vi "Actor Core.vi"(8 "error in":errorcluster, 11 "Composite User Interface in":refnum<class "GUI.lvclass">) -> (0 "error out":errorcluster, 3 "Actor out":refnum<class "Actor.lvclass">)   [LabVIEW 2020, in "GUI.lvlib" / "GUI.lvclass"]
doc: "The user interface for this panel.\n----\nCopyright: MGI 2016\nAuthor: Derek Trepanier"
uses:
  GUI.lvclass
  Task selection df.ctl
  Task info df.ctl
  C:/Program Files/National Instruments/LabVIEW 2020/vi.lib/MGI/Panel Manager/Panel Actor/Panel Actor/Panel Actor.lvclass
  C:/Program Files/National Instruments/LabVIEW 2020/vi.lib/ActorFramework/Actor/Actor.lvclass
  <vilib>/ActorFramework/Actor/Actor.lvclass
  Subject and File df.ctl
  Automate df.ctl
  <vilib>/MGI/Panel Manager/Panel/Window Position/Reference Position/Ref Display/Ref Display.lvclass
  C:/Program Files/National Instruments/LabVIEW 2020/vi.lib/MGI/Panel Manager/Panel/Window Position/Window Position.lvclass
  Acceleration Markers df.ctl
  EMG channels df.ctl
  Task Active Enum df.ctl
  Logging/Logging.lvclass
  GUI.lvclass/GUI.ctl
  NI Force Task/NI Force Task.lvclass
  <vilib>/ActorFramework/Actor/Actor.lvclass/Actor.ctl
  <vilib>/ActorFramework/Message Enqueuer/Message Enqueuer.lvclass/Message Enqueuer.ctl
  NI Force Task Messages/Update Template Graph Msg/Update Template Graph Msg.lvclass/Update Template Graph Msg.ctl
  Accelerometer/Accelerometer.lvclass
  Collection Type df.ctl
  Marker Enum.ctl
  <vilib>/ActorFramework/Message Enqueuer/Init from Existing Queue.vi
  <vilib>/ActorFramework/Message Enqueuer/Enqueue.vi
  <vilib>/MGI/Panel Manager/Panel/Panel/Window/Window.lvclass
  C:/Program Files/National Instruments/LabVIEW 2020/vi.lib/MGI/Panel Manager/Panel/Panel/Panel.lvclass
  NI Force Task Messages/Update Template Graph Msg/Update Template Graph Msg.lvclass
  C:/Program Files/National Instruments/LabVIEW 2020/vi.lib/ActorFramework/Message/Message.lvclass
  <vilib>/MGI/Panel Manager/Panel/Panel/Subpanel/Subpanel.lvclass
  <vilib>/ActorFramework/Stop Msg/Stop Msg.lvclass
  <vilib>/MGI/Panel Manager/Panel/Panel/Window/Window.vi
  <vilib>/ActorFramework/Message Priority Queue/Priority Enqueue.vi
  <vilib>/MGI/Panel Manager/Panel/Panel/Subpanel/Subpanel.vi
  <vilib>/ActorFramework/Message Enqueuer/Message Enqueuer.lvclass
  <vilib>/MGI/Panel Manager/Panel Actor/Panel Actor/Panel Actor.lvclass
  <vilib>/MGI/Panel Manager/Panel/Panel.lvlib
  GUI Messages/Set Template Data Msg/Set Template Data Msg.lvclass
  NI Force Task Messages/Start Trial Msg/Start Trial Msg.lvclass
  NI Force Task Messages/Stop Trial Msg/Stop Trial Msg.lvclass
  NI Force Task Messages/External Shutdown Msg/External Shutdown Msg.lvclass
  Accelerometer Messages/Stop Trial Msg/Stop Trial Msg.lvclass
  Accelerometer Messages/Initialize Accel Task Msg/Initialize Accel Task Msg.lvclass
  Accelerometer Messages/Start Trial Msg/Start Trial Msg.lvclass
  Accelerometer Messages/External Shutdown Msg/External Shutdown Msg.lvclass
  NI Force Task Messages/Calibrate Force Msg/Calibrate Force Msg.lvclass
  NI Force Task Messages/Collect MVC Msg/Collect MVC Msg.lvclass
  GUI Messages/Does File Exist Msg/Does File Exist Msg.lvclass
  Logging Messages/TDMS Cleanup Msg/TDMS Cleanup Msg.lvclass
  GUI Messages/Save or Load Config Msg/Save or Load Config Msg.lvclass
  GUI Messages/Delete Config Msg/Delete Config Msg.lvclass
  GUI Messages/MVC Collect File Check Msg/MVC Collect File Check Msg.lvclass
  NI Force Task Messages/Launch Viewer Msg/Launch Viewer Msg.lvclass
  NI Force Task Messages/Calibrate Potentiometers Msg/Calibrate Potentiometers Msg.lvclass
  NI Force Task Messages/Initialize Movement Task Msg/Initialize Movement Task Msg.lvclass
  NI Force Task Messages/Initialize Force Task Msg/Initialize Force Task Msg.lvclass
  GUI Messages/Update Patterns Array Msg/Update Patterns Array Msg.lvclass
  C:/Program Files/National Instruments/LabVIEW 2020/vi.lib/MGI/Panel Manager/Panel/Window Position/Reference Position/Reference Position.lvclass
  C:/Program Files/National Instruments/LabVIEW 2020/vi.lib/MGI/Panel Manager/Panel/Window Position/Reference Position/Ref Display/Ref Display.lvclass
  GUI Messages/Task Type Change Msg/Task Type Change Msg.lvclass
  GUI Messages/Accel Marker Update Msg/Accel Marker Update Msg.lvclass
  NI Force Task Messages/Initiallize EMG Task Msg/Initiallize EMG Task Msg.lvclass
  Logging Messages/TDMS Cleanup EMG only Msg/TDMS Cleanup EMG only Msg.lvclass
  GUI Messages/Scale Regression Msg/Scale Regression Msg.lvclass
panel:
  out "MVC Temp":dbl
  in  "Monitor Select":refnum<class "Ref Display.lvclass">
  out "Abort Signal":bool
  in  "Subject and File":T1={"File Save Path"=path "\\\\coe-fs.engr.tamu.edu\\Grads/renee.woodruff/Documents/LabVIEW Data/Bimanual Coord DAQ", "File Name "="test"}
  in  "Tab Control":T2(tab)
  in  "Abort Task":bool caption="Preview Task"
  in  "Task Previewed?":bool
  in  "Preview Task":bool
  in  "Task Selection":T3={"Task Type Select"=enum."Frequency Task", "Input Select Type"=enum."Force Input", "Collect EMG?"=FALSE, "Collect acceleration?"=TRUE, "EMG Rate"=1000, "Acceleration Rate"=50} {"Acceleration Rate" min=5 max=1000 step=1; "EMG Rate" min=1 step=1}
  in  "Task Info Cluster":T4={"Number of Trials"=1, "Sampling Rate (Hz)"=100, "Trial Duration (s)"=8, "Adjusted MVC (N)"=5.0, "R Phase"=0, "L Phase"=0, "L Pattern"=1, "R Pattern"=1, "Time Between Trials (s)"=5, "Lissajous Speed"=10} {"Lissajous Speed" min=1 max=200; "Time Between Trials (s)" min=1 step=1; "R Pattern" min=1 max=20 step=1; "L Pattern" min=1 max=20 step=1; "L Phase" max=360 step=1; "R Phase" max=360 step=1; "Adjusted MVC (N)" min=0.1 max=50.0 step=0.10000000149011612 format="%.1f"; "Trial Duration (s)" min=1 step=1; "Sampling Rate (Hz)" min=1 step=1; "Number of Trials" min=1 step=1}
  in  "Task Start":bool caption="Force Task Start"
  in  "Delete Config":bool
  in  "Config Select":string(combo) caption="Load or Save Config:"
  in  "Collect MVC":bool
  in  "MVC Cluster input":T5={"MVC Sampling Rate"=200, "MVC Duration"=3, "MVC Percent"=15} {"MVC Percent" max=100 step=1 scale=0.0..40.0; "MVC Duration" min=1 step=1; "MVC Sampling Rate" min=1 step=1}
  out "Raw MVC Clust":cluster{"Raw MVC Left":dbl, "Raw MVC Right":dbl}
  out "Adjusted MVC Cluster":T6
  out "Slope Int":dbl[][](array[numeric])
  in  "Calc Regression":bool
  in  "TScale Calibration":dbl[][](array[numeric])
  in  "Calibrate Pot":bool caption="Calibrate"
  in  "Calibrate Transducers":bool
  out "Force Calibration Cluster":cluster{"Left":dbl, "Right":dbl}
  in  "Force Calibration Input Cluster":T7={"Force Calib Sampling Rate"=200, "Force Calib Duration"=3}
  out "Pot Calibration Cluster":cluster{"Left 2":dbl, "Right 2":dbl}
  in  "Pot Calibration Input Clust":T7={"Force Calib Sampling Rate"=200, "Force Calib Duration"=3}
  in  "EMG Master Config":T8
  in  "DAQ Physical Channels":T9={"Force Transducer: Left"="Dev1/ai6", "Force Transducer: Right "="Dev1/ai8", "EMG: Left"="Dev1/ai1", "EMG: Right"="Dev1/ai9", "Potentiometer: Left"="Dev2/ai2", "Potentiometer: Right"="Dev2/ai3"}
  out "Trial Num":i32=1
  in  "Tab Control Automation":T10(tab)
  in  "Auto Clust":T11={"Automate?"=FALSE, "Num Parabs"=1, "Patterns Array"=[], "Phase Array"=[]} {"Num Parabs" min=1 step=1}
  in  "Acceleration Markers":T12
  in  "Second Monitor":bool caption="Display task on second monitor"
  in  "Task window closed?":bool
  # "Save File Information"
  # "(do not include file type)"
  # "Task Type"
  # "Left Arm"
  # "Right Arm"
  # "Force Calibration"
  # "Regression in Use"
  # "Weight (lbs)"
  # "Left (V)"
  # "Right (V)"
  # "Slope"
  # "Int."
  # "Left"
  # "Right"
  # "Re-calculates regression line to convert volts to Newtons for transducer.\nOnly needs to be done if transducer is changed."
  # "Potentiometer Calibration"
  # "Note: running EMG Master \nMode will simultaneously \ncollect EMG data from the \nspecified channels on the right.\nOnly 1 laptop should run EMG\nMaster Mode at a time\n\nForce/potentiometer data will\nNOT be collected in this mode"
  # "- Check the Device Configuration tab before running. Make sure that the Device Name is valid for each channel by selecting the dropdown menu to see if the value is listed. If yes, change nothing. If yes, change the channel to a listed Device Name/Channel combination. \n- Re-calibrate transducers every time 'gravity' is changed or starting a test session for the day in the Calibration tab\n- In the Task Config tab, it is best when Force Sampling Rate (Hz) is a multiple of the EMG Sampling Rate (Hz). If you are not collecting EMG, this doesn't matter\n- If the cursor ever becomes 'busy', seen as a blue circle, do not select anything until the cursor is no longer busy\n- If the config drop down does not work, open '/config/config_list.txt' and type in \"Create New...\". Save the .txt and then close it. Close the program and try again\n- Make sure that the headset is connected as the secondary display, if applicable\n- Note: Acceleration Markers will be cleared for each new set of trials \n- Acceleration markers can also be added using keyboard inputs. To add markers this way, make sure the User Interface window is in focus"
  # "Patterns"
  # "Phase"
  # "Left        Right"
  # "Left        Right"
  # "Insert Acceleration Markers"
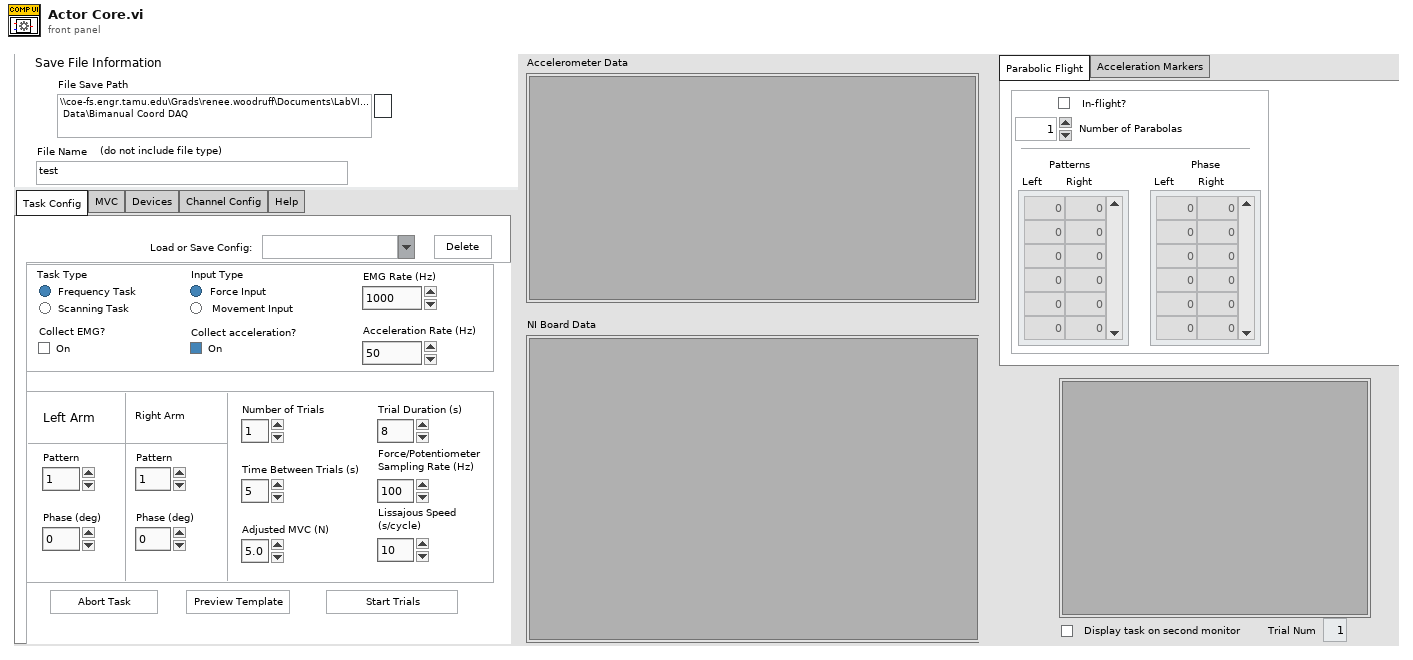
[diagram p1: front panel]
types:
  T1 = typedef "Subject and File df.ctl" = cluster{"File Save Path":path, "File Name ":string}
  T2 = enum32{"Task Config", "MVC", "Devices", "Channel Config", "Help"}
  T3 = typedef "Task selection df.ctl" = cluster{"Task Type Select":enum32{"Frequency Task", "Scanning Task"}, "Input Select Type":enum32{"Force Input", "Movement Input"}, "Collect EMG?":bool, "Collect acceleration?":bool, "EMG Rate":u16, "Acceleration Rate":u16}
  T4 = typedef "Task info df.ctl" = cluster{"Number of Trials":u8, "Sampling Rate (Hz)":u16, "Trial Duration (s)":u8, "Adjusted MVC (N)":dbl, "R Phase":i32, "L Phase":i32, "L Pattern":u8, "R Pattern":u8, "Time Between Trials (s)":u8, "Lissajous Speed":u16}
  T5 = cluster{"MVC Sampling Rate":u16, "MVC Duration":u8, "MVC Percent":u8}
  T6 = cluster{"Adjusted MVC Left":dbl, "Adjusted MVC Right":dbl}
  T7 = cluster{"Force Calib Sampling Rate":u16, "Force Calib Duration":u8}
  T8 = typedef "EMG channels df.ctl" = cluster{"EMG Master":bool, "EMGL1":tag, "EMGR1":tag, "EMGL2":tag, "EMGR2":tag, "EMGL3":tag, "EMGR3":tag, "EMGL4":tag, "EMGR4":tag, "EMGL5":tag, "EMGR5":tag, "EMGL6":tag, "EMGR6":tag, "EMGL7":tag, "EMGR7":tag, "EMGL8":tag, "EMGR8":tag}
  T9 = cluster{"Force Transducer: Left":tag, "Force Transducer: Right ":tag, "EMG: Left":tag, "EMG: Right":tag, "Potentiometer: Left":tag, "Potentiometer: Right":tag}
  T10 = enum32{"Parabolic Flight", "Acceleration Markers"}
  T11 = typedef "Automate df.ctl" = cluster{"Automate?":bool, "Num Parabs":u16, "Patterns Array":u8[][], "Phase Array":i32[][]}
  T12 = typedef "Acceleration Markers df.ctl" = cluster{"Partial g marker":bool, "1g marker":bool, "Hyper G marker":bool, "Custom Marker":bool, "Enter Marker Name":string, "Marker List":i32, "Delete Row":bool}
  T13 = typedef "Task Active Enum df.ctl" = enum16{"Idle", "Start Freq Task", "Start Freq Task and Accel", "Start Scanning Task", "Start Scanning Task and Accel", "Preview Template", "Collect MVC", "Calibrate Force", "Calibrate Potentiometers", "Stop Helper", "EMG Mode", "EMG and Accel Mode", "Task Config Update"}
  T14 = typedef "NI_LVConfig.lvlib/Config Data RefNum.ctl" = refnum<k1>
  T15 = cluster{"Preview Task":refnum<user-event>, "Calibration Val Update":refnum<user-event>, "Raw MVC update":refnum<user-event>, "Task Info Load":refnum<user-event>, "Task Select Load":refnum<user-event>, "Config Update":refnum<user-event>, "Task window update":refnum<user-event>, "Pot Cal Value Update":refnum<user-event>, "Auto Clust Update":refnum<user-event>, "Accel Markers":refnum<user-event>, "Slope Int":refnum<user-event>, "Trial Num Update":refnum<user-event>}
  T16 = cluster{"Event Registration Refnum":refnum<event-registration>, "Pnl Actor":refnum<event-registration>}
  T17 = enum8{"Enabled", "Disabled", "Disabled and Grayed Out"}
  T18 = typedef "Marker Enum.ctl" = enum16{"Predefined", "Custom", "Delete Row", "Clear all"}
  T19 = typedef "LVPoint32TypeDef.ctl" = cluster{"Horizontal":i32, "Vertical":i32}
  T20 = typedef "LVRowAndColumnTypeDef.ctl" = cluster{"Row":i32, "Column":i32}
  T21 = enum16{"open", "open or create", "create or replace", "create", "open (read-only)"}
  T22 = typedef "Collection Type df.ctl" = enum32{"Force Input", "Movement Input", "EMG only"}
  T23 = cluster{"Force Task":refnum<class "NI Force Task.lvclass">, "Window out":refnum<class "Window.lvclass">}
  T24 = cluster{"Accelerometer":refnum<class "Accelerometer.lvclass">, "Subpanel Out":refnum<class "Subpanel.lvclass">}
  T25 = cluster{"Accelerometer":refnum<class "Panel Actor.lvclass">, "Subpanel Out":refnum<class "Panel.lvclass">}[]
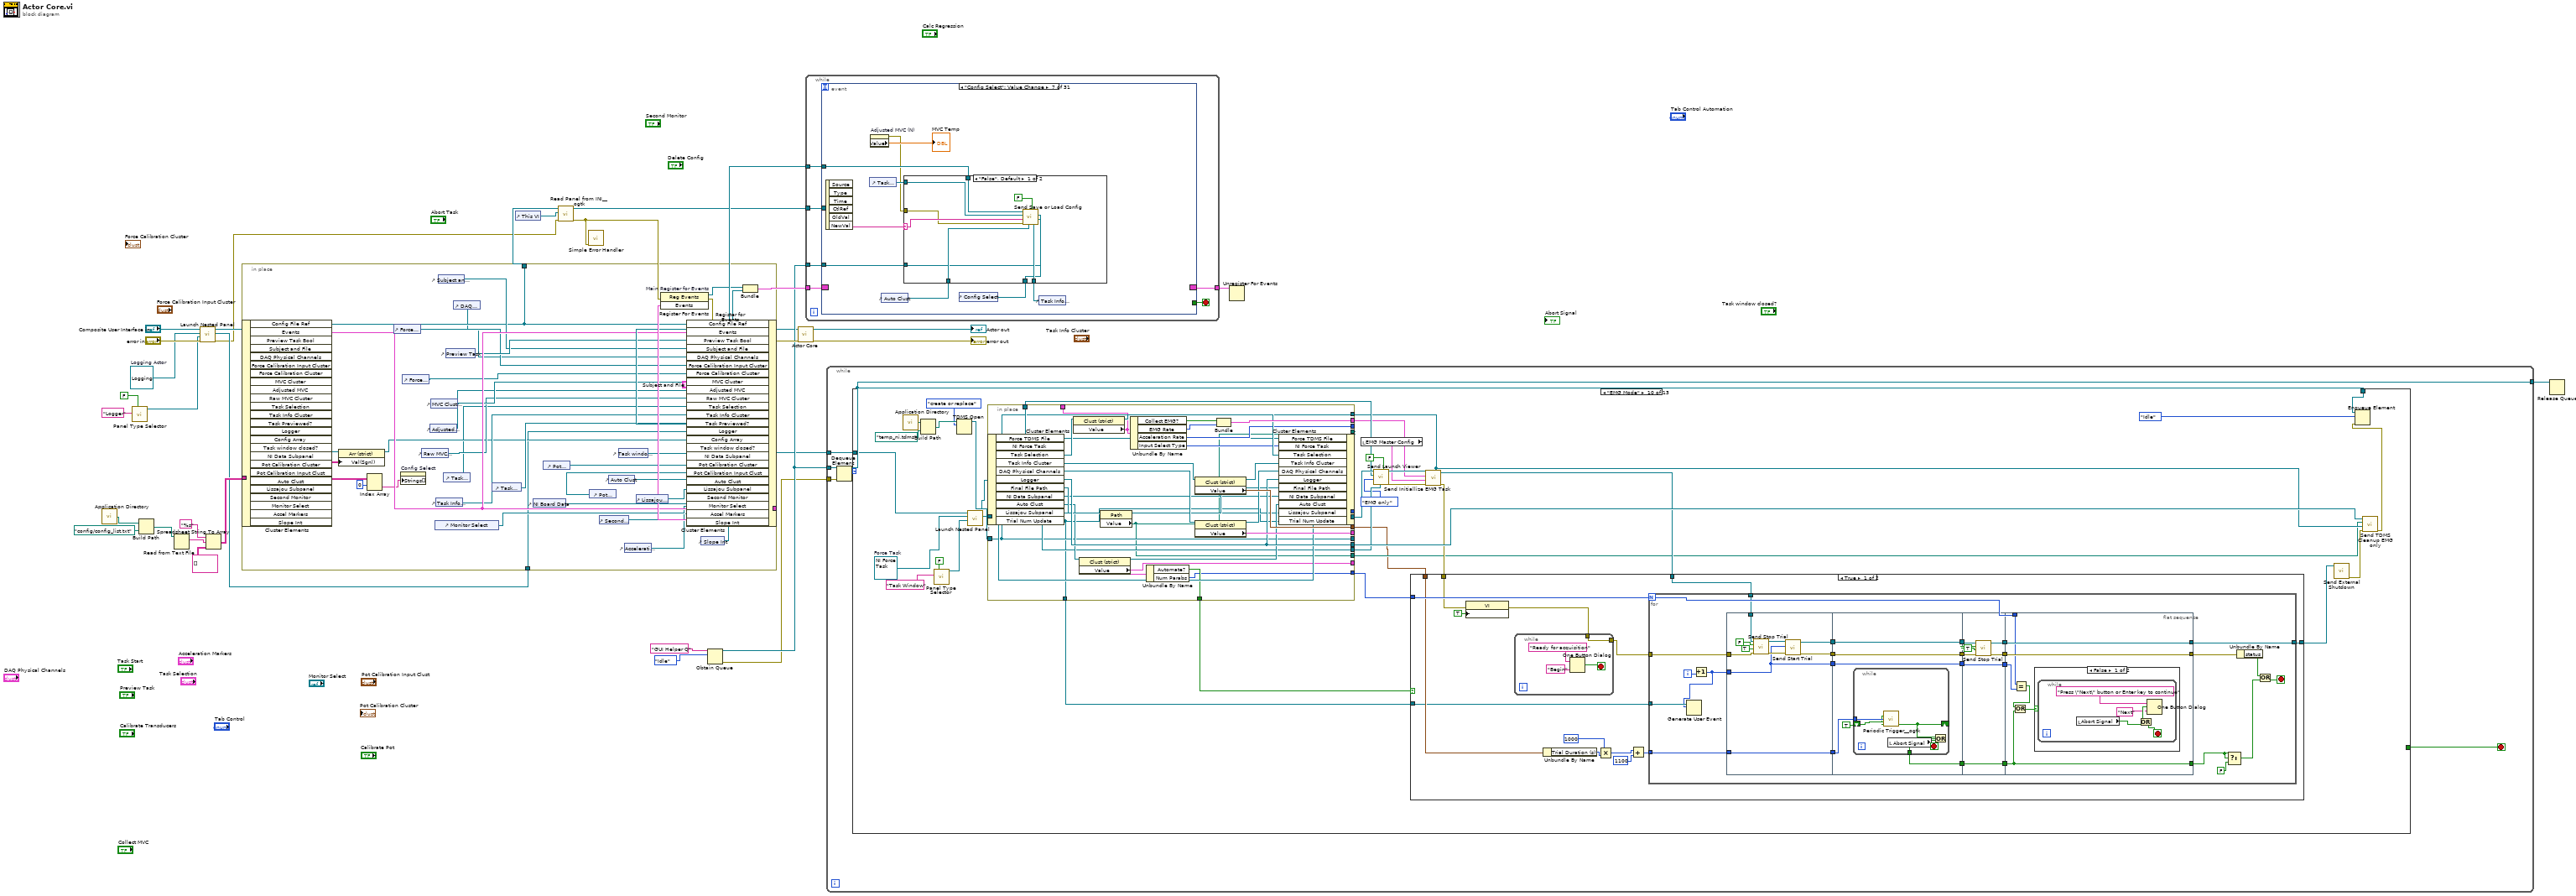
[diagram p0: block diagram]
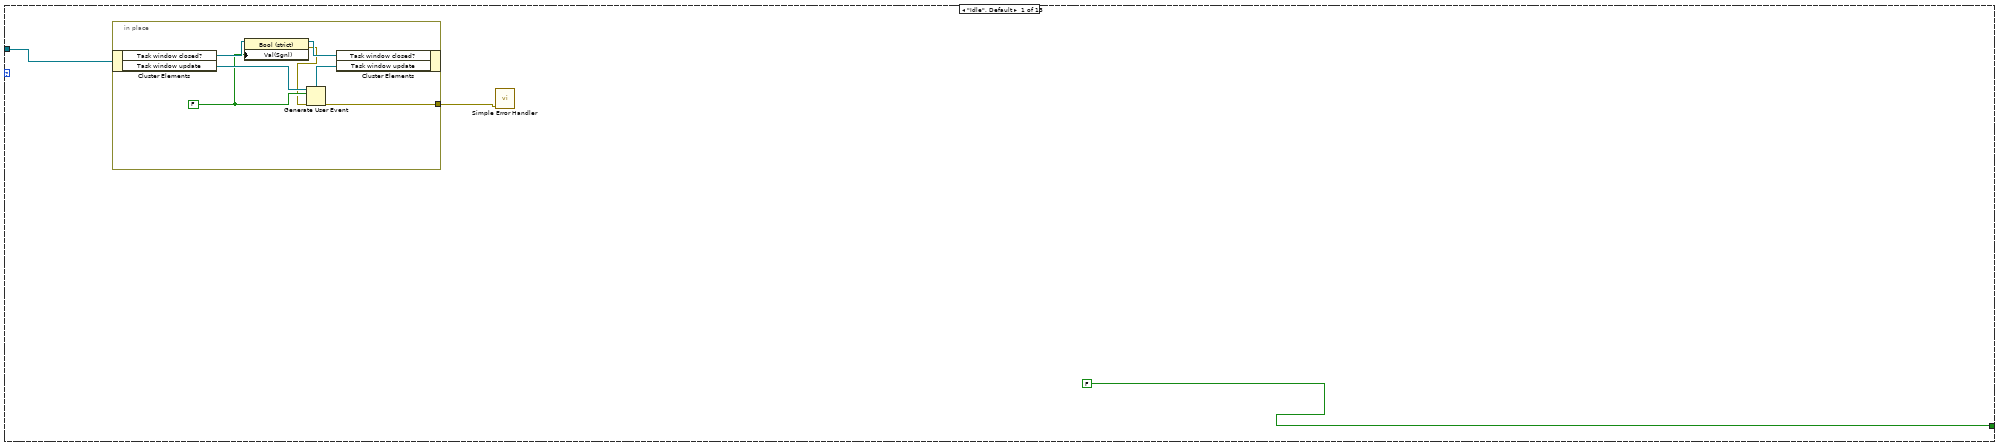
[diagram p2: hidden frame]
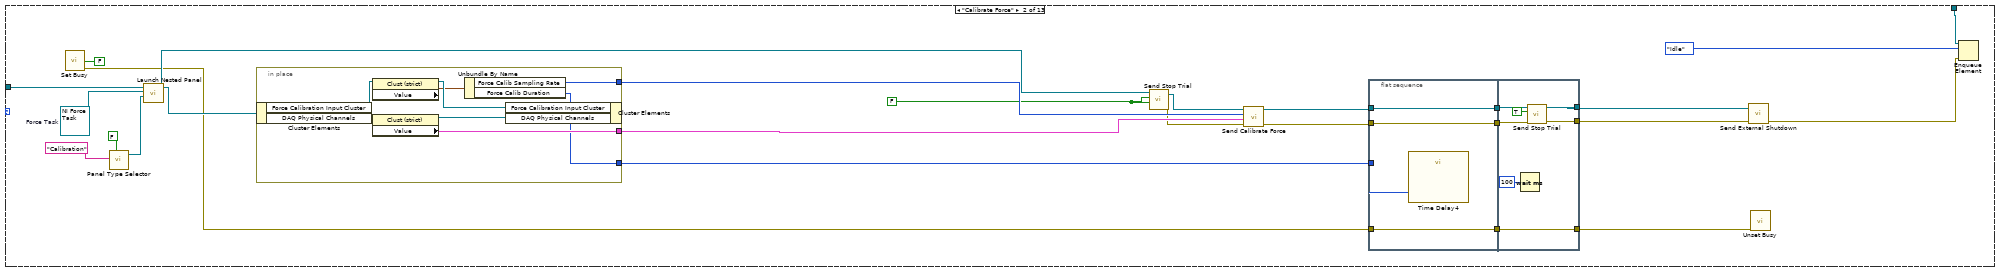
[diagram p3: hidden frame]
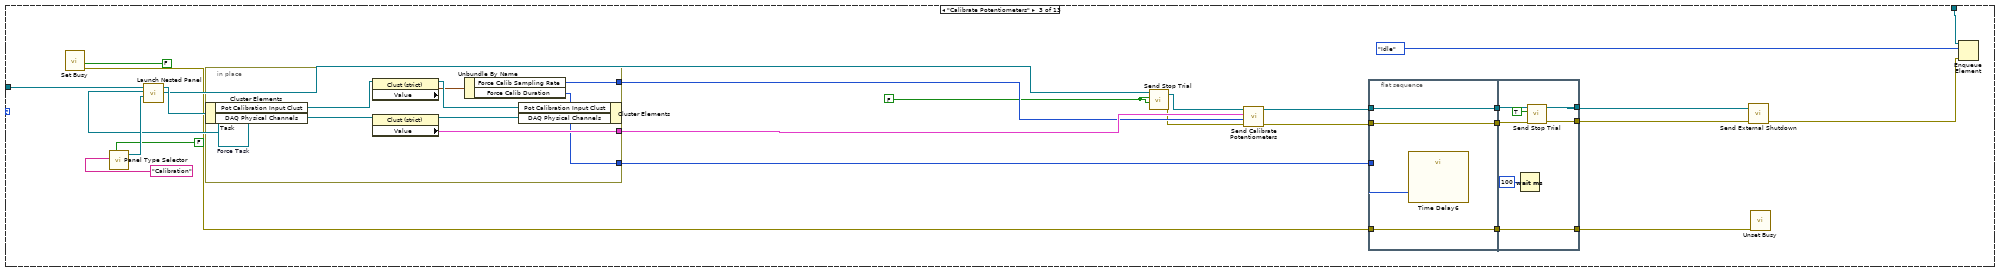
[diagram p4: hidden frame]
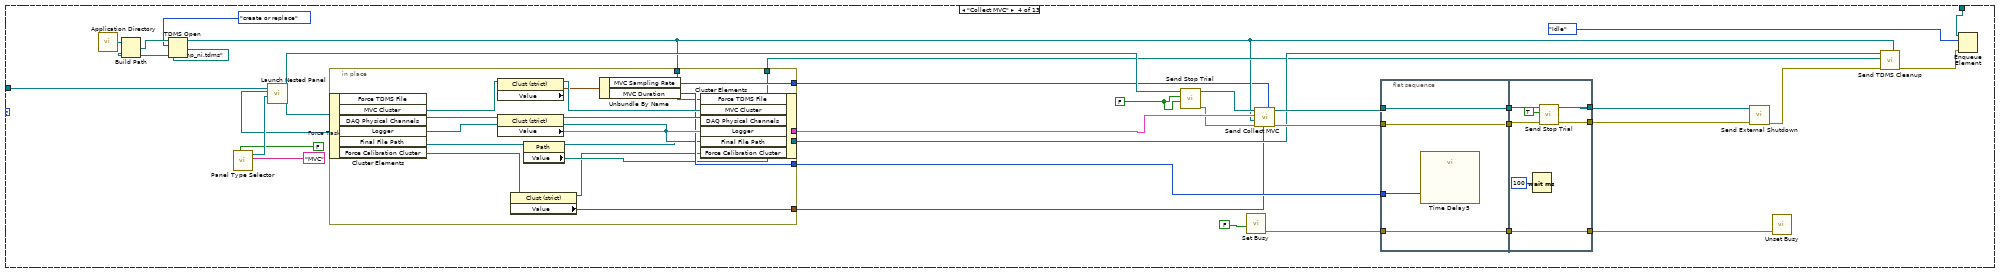
[diagram p5: hidden frame]
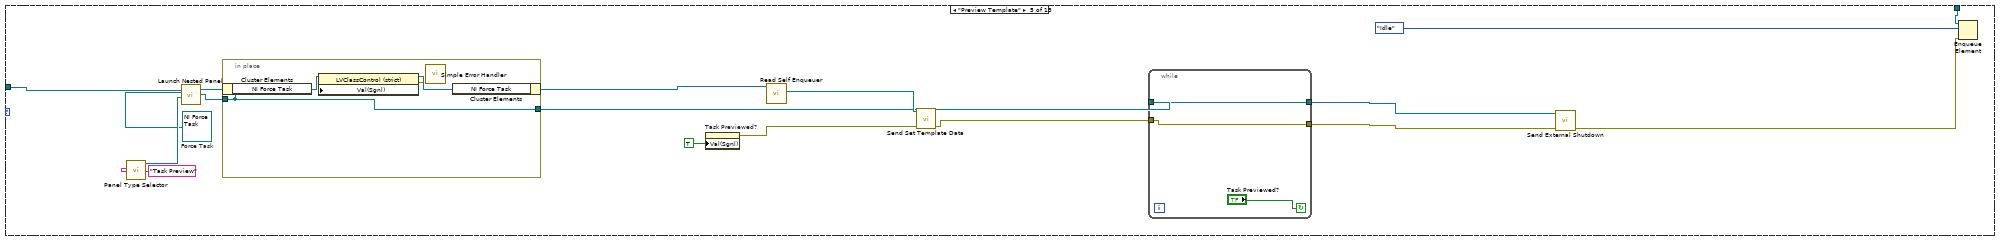
[diagram p6: hidden frame]
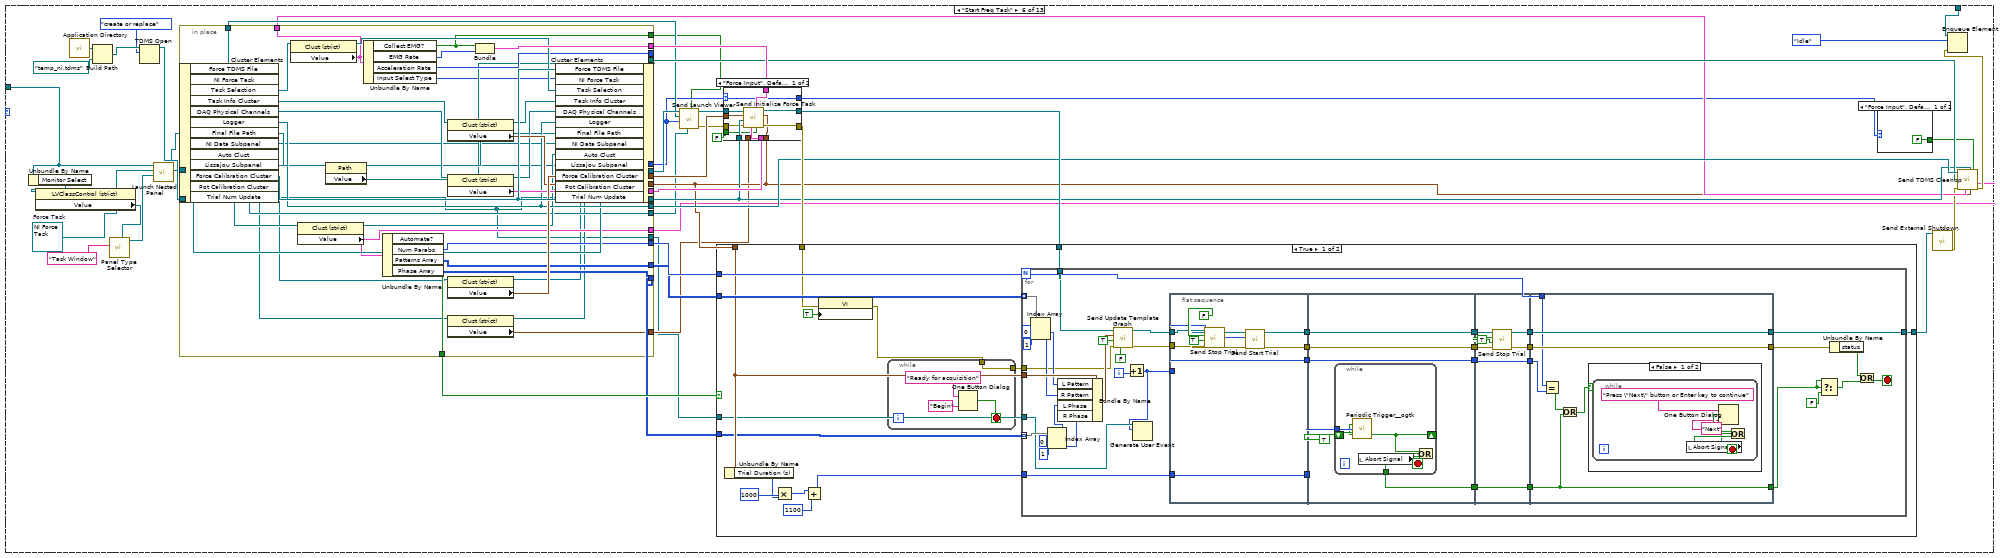
[diagram p7: hidden frame]
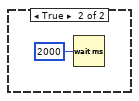
[diagram p8: hidden frame]
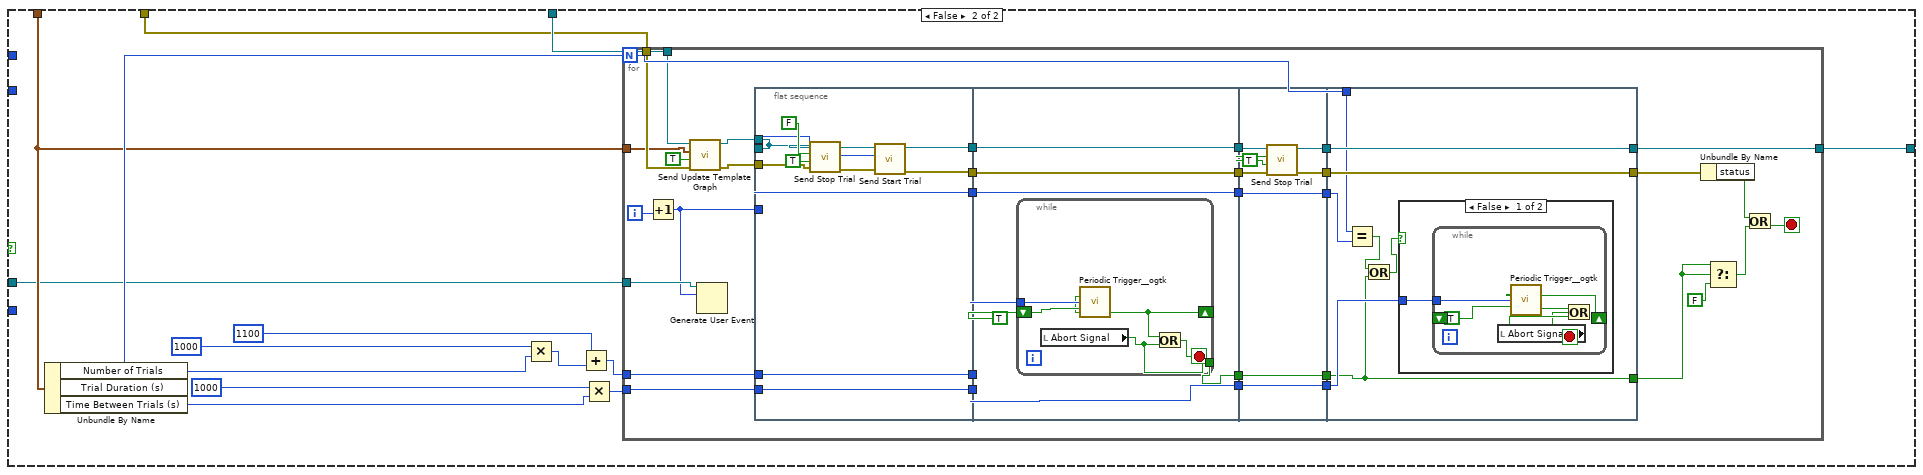
[diagram p9: hidden frame]
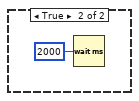
[diagram p10: hidden frame]
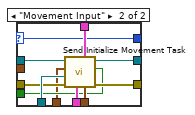
[diagram p11: hidden frame]
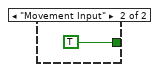
[diagram p12: hidden frame]
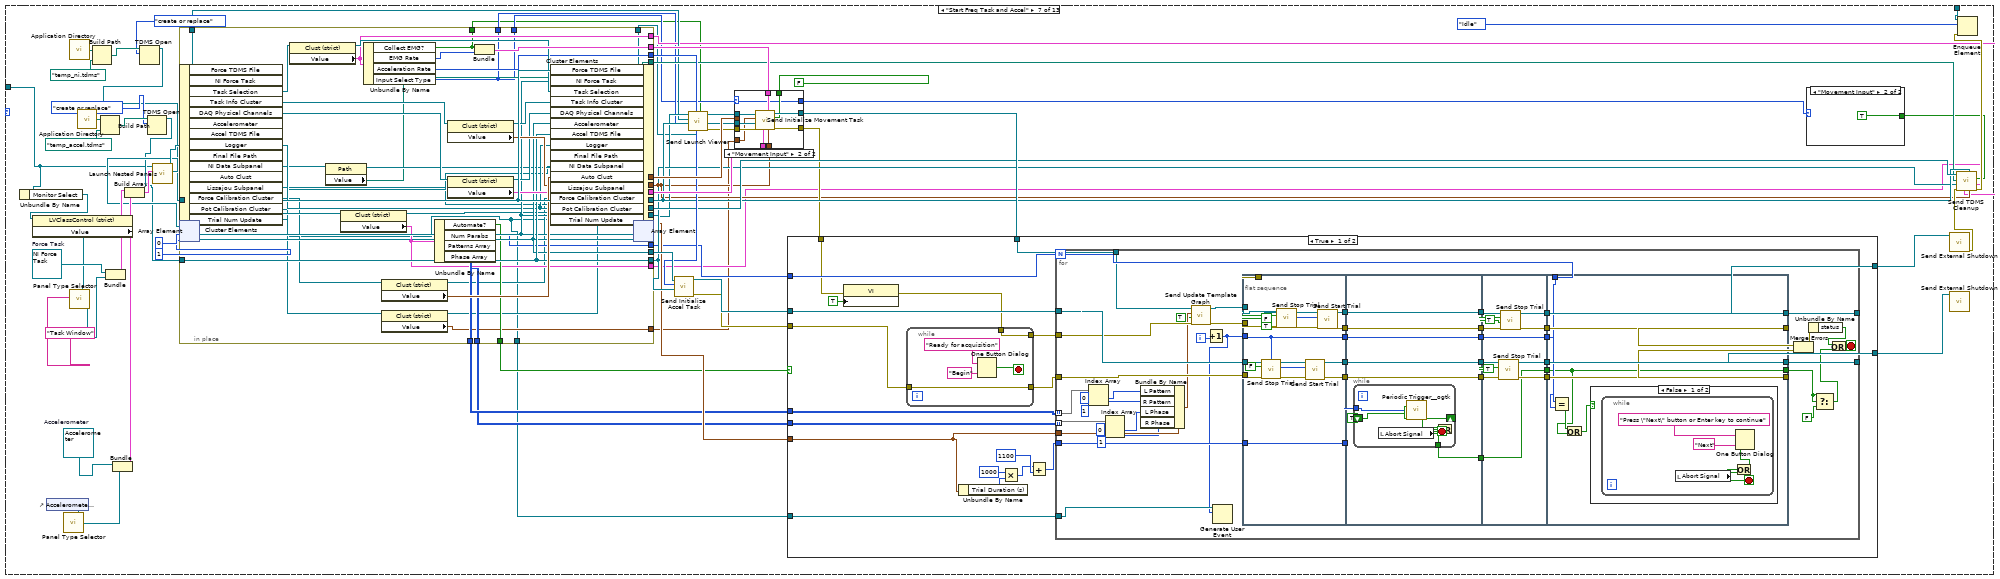
[diagram p13: hidden frame]
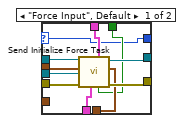
[diagram p14: hidden frame]
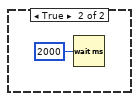
[diagram p15: hidden frame]
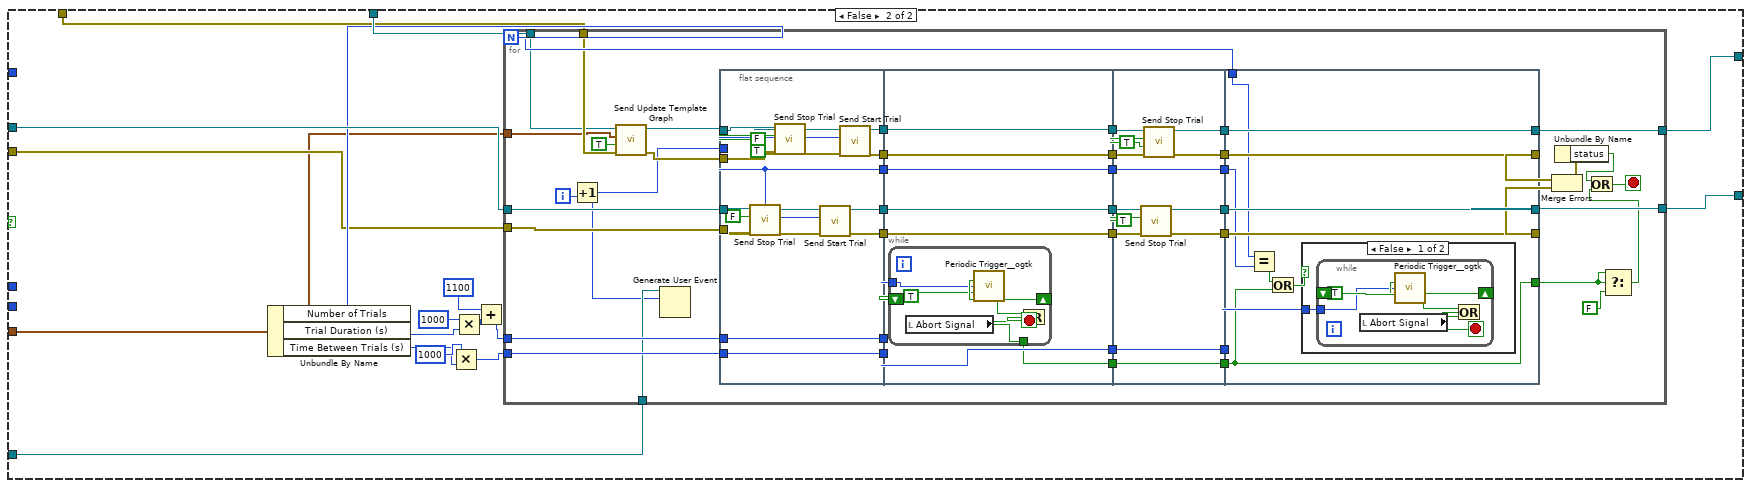
[diagram p16: hidden frame]
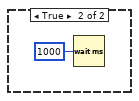
[diagram p17: hidden frame]
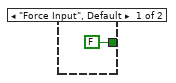
[diagram p18: hidden frame]
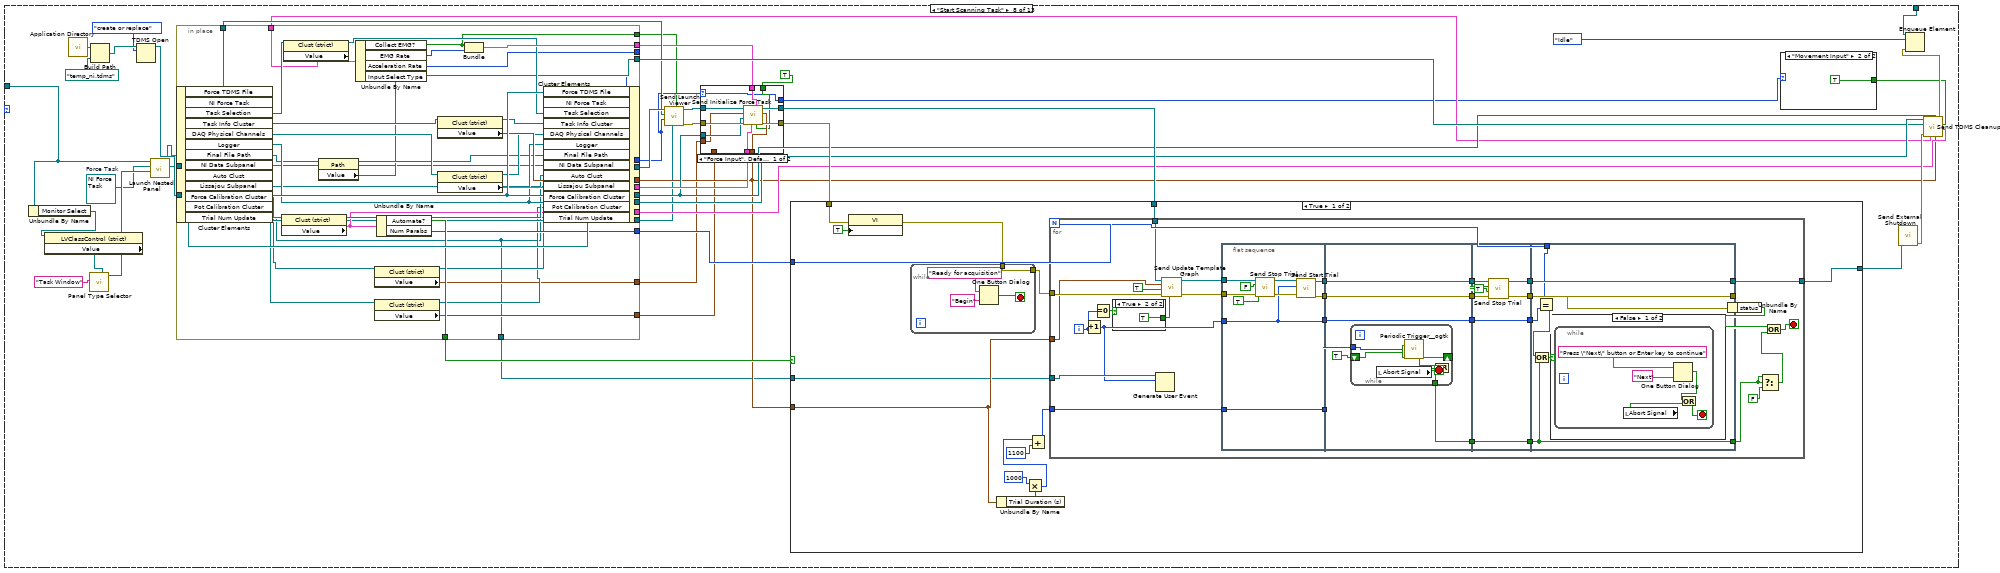
[diagram p19: hidden frame]
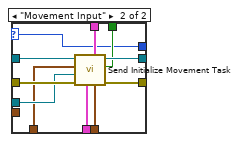
[diagram p20: hidden frame]
diagram:
  w5 = refnum<class "Logging.lvclass"> refnum  # Logging Actor
  n1 = call <vilib>:"Application Directory.vi"() -> ("Application Directory"=w15:path)
  n2 = call-poly <vilib>:"Panel Type Selector.vi"("Autoshow? (T)"=FALSE, "Default Title"="Logger") -> ("Window out"=w4:refnum<class "Window.lvclass">)  [unwired: 8 in, 1 out]
  n3 = Build Path(base path=w15, name or relative path=path "config/config_list.txt") -> (appended path=w13:path)
  n4 = Read from Text File(file (use dialog)=w13) -> (text=w12:string)  [unwired: 3 in, 3 out]
  n5 = call <vilib>:"Launch Nested Panel.vi"("error in (no error)"="error in", "Panel"=w4, "Nested Panel Actor"=w5, "Panel Actor in"="Composite User Interface in") -> ("error out"=w2:errorcluster, "Nested Actor's Enqueuer"=w3:refnum<class "Message Enqueuer.lvclass">, "Panel Actor out"=w20:refnum<class "GUI.lvclass">)  [unwired: 4 in, 1 out]
  n6 = Spreadsheet String To Array(format string="%s", spreadsheet string=w12, array type (2D Dbl)=string[][] []) -> (array=w9:string[][])  [unwired: 1 in]
  n7 = in-place {
    in-place-border: [w66] -> w19
    in-place-border: w9 -> [w53]
    in-place-border: [w52] -> w7
    in-place-border: w3 -> [w40]
    n8 = in-place-cluster #1(w20) -> ("Config File Ref"=w52:T14, "Events"=w66:T15, "Config Array"=w56:refnum<vi>)  [unwired: 22 out]
    n9 = property class="Arr (strict)"(reference=w56, "Val(Sgnl)"=w53) -> (reference out=w50:refnum<vi>)  [unwired: 1 in, 1 out]
    n10 = Index Array(array=w53, index (row)=0) -> (element=w54:string[])  [unwired: 1 in]
    n11 = control-ref of="Force Calibration Input Cluster"() -> (w59:refnum<vi>)
    n12 = property on="Config Select" class="CmbBox"("Strings[]"=w54) -> ()  [unwired: 2 in, 2 out]
    n13 = control-ref of="Force Calibration Cluster"() -> (w58:refnum<vi>)
    n14 = control-ref of="Raw MVC Clust"() -> (w61:refnum<vi>)
    n15 = control-ref of="Adjusted MVC Cluster"() -> (w60:refnum<vi>)
    n16 = control-ref of="MVC Cluster input"() -> (w62:refnum<vi>)
    n17 = control-ref of="Monitor Select"() -> (w41:refnum<vi>)
    n18 = control-ref of="Task Info Cluster"() -> (w63:refnum<vi>)
    n19 = control-ref of="Subject and File"() -> (w64:refnum<vi>)
    n20 = control-ref of="Task Selection"() -> (w45:refnum<vi>)
    n21 = control-ref of="Preview Task"() -> (w65:refnum<vi>)
    n22 = control-ref of="DAQ Physical Channels"() -> (w48:refnum<vi>)
    n23 = control-ref of="Task Previewed?"() -> (w57:refnum<vi>)
    n24 = control-ref of="NI Board Data"() -> (w49:refnum<vi>)
    n25 = control-ref of="Pot Calibration Cluster"() -> (w46:refnum<vi>)
    n26 = control-ref of="Pot Calibration Input Clust"() -> (w47:refnum<vi>)
    n27 = control-ref of="Second Monitor"() -> (w42:refnum<vi>)
    n28 = control-ref of="Auto Clust"() -> (w44:refnum<vi>)
    n29 = control-ref of="Task window closed?"() -> (w51:refnum<vi>)
    n30 = control-ref of="Acceleration Markers"() -> (w39:refnum<vi>)
    n31 = control-ref of="Lissajou Subpanel"() -> (w43:refnum<vi>)
    n32 = control-ref of="Slope Int"() -> (w38:refnum<vi>)
    n33 = in-place-cluster #1("Config File Ref"=w52, "Events"=w66, "Preview Task Bool"=w65, "Subject and File"=w64, "DAQ Physical Channels"=w48, "Force Calibration Input Cluster"=w59, "Force Calibration Cluster"=w58, "MVC Cluster"=w62, "Adjusted MVC"=w60, "Raw MVC Cluster"=w61, "Task Selection"=w45, "Task Info Cluster"=w63, "Task Previewed?"=w57, "Logger"=w40, "Config Array"=w50, "Task window closed?"=w51, "NI Data Subpanel"=w49, "Pot Calibration Cluster"=w46, "Pot Calibration Input Clust"=w47, "Auto Clust"=w44, "Lissajou Subpanel"=w43, "Second Monitor"=w42, "Monitor Select"=w41, "Accel Markers"=w39, "Slope Int"=w38) -> (w18:refnum<class "GUI.lvclass">)
  }
  n34 = control-ref of="This VI"() -> (w8:refnum<vi>)
  n35 = call <userlib>:"Read Panel from INI__ogtk.vi"("error in (no error)"=w2, "VI ref"=w8, "refnum"=w7) -> ("error out"=w1:errorcluster, "refnum out"=w6:T14)  [unwired: 7 in]
  n36 = call <vilib>:"Simple Error Handler.vi"("error in (no error)"=w1) -> ()  [unwired: 4 in, 5 out]
  n37 = register-events "Main Register for Events"(error in=w1, w19) -> (reference out=w29:refnum<event-registration>, error out=w30:errorcluster)  [unwired: 1 in]
  n38 = Obtain Queue(name (unnamed)="GUI Helper Q", element data type=Task_Active_Enum_df."Idle" ("Task Status Enum")) -> (queue out=w24:refnum<queue>, error out=w23:errorcluster)  [unwired: 3 in, 1 out]
  n39 = call <vilib>:"Register for Events.vi"("Error In"=w30, "Panel Actor in"=w18) -> ("Error Out"=w35:errorcluster, "Panel Actor out"=w22:refnum<class "GUI.lvclass">, "Pnl Actor"=w28:refnum<event-registration>, "Self Enqueuer"=w34:refnum<class "Message Enqueuer.lvclass">)  [unwired: 6 in]
  n40 = Bundle("Event Registration Refnum"=w29, "Pnl Actor"=w28) -> (w27:T16)  [unwired: 1 in]
  n41 = call-parent "Actor Core.vi"("error in"=w35, "Panel Actor in"=w22) -> ("error out"=→"error out":errorcluster, "Actor out"=→"Actor out":refnum<class "Actor.lvclass">)  [unwired: 8 in]
  n42 = while {
    tunnel: w27 -> [w72]
    tunnel: w34 -> [w71]
    tunnel: [w69] -> w33
    tunnel: w24 -> [w68]
    tunnel: w6 -> [w67]
    stop <- w70 stop-if-true
    n43 = event shown="[6] \"Config Select\": Value Change" {
      selector: w72 -> [_ _ _ _ _ _ _ _ _ _ _ _ _ _ _ _ _ _ _ _ _ _ _ _ _ _ _ _ _ _ _]
      dyn-events: [_ _ _ _ _ _ _ _ _ _ _ _ _ _ _ _ _ _ _ _ _ _ _ _ _ _ _ _ _ _ _] -> w69
      timeout: _ -> [_ _ _ _ _ _ _ _ _ _ _ _ _ _ _ _ _ _ _ _ _ _ _ _ _ _ _ _ _ _ _]
      tunnel: w71 -> [w75 _ w130 _ w139 _ w148 _ w179 w189 _ _ _ w251 w258 _ _ w265 _ _ w291 _ w297 w301 w307 w308 _ _ _ w334 _]
      tunnel: [_ _ _ _ _ _ _ _ _ _ _ _ _ _ _ _ _ _ _ _ _ _ _ _ _ _ _ _ _ _ w335] -> w70
      tunnel: w68 -> [w92 _ _ _ _ _ w143 _ _ _ _ _ _ _ _ w261 w263 w264 _ _ w290 _ _ _ _ _ _ _ w329 _ w336]
      tunnel: w67 -> [_ _ _ _ _ _ _ _ _ _ _ _ _ _ _ _ _ _ _ _ _ _ _ _ _ _ _ _ _ w332 _]
      event User Event {
        w78 = cluster{u32, u32}[] [{12369084, 12369084}, {12369084, 12369084}, {13816530, 13816530}] ("Colors [4]")
        n44 = event-data() -> ()  [unwired: 1 in, 1 out]
        n45 = control-ref of="Calibrate Pot"() -> (w82:refnum<vi>)
        n46 = control-ref of="Preview Task"() -> (w80:refnum<vi>)
        n47 = control-ref of="Delete Config"() -> (w84:refnum<vi>)
        n48 = Enqueue Element(queue=w92, element=Task_Active_Enum_df."Idle") -> ()  [unwired: 2 in, 3 out]
        n49 = property on="Acceleration Markers" class="Clust"() -> ("Controls[]"=w85:refnum<vi>[])  [unwired: 2 in, 2 out]
        n50 = call "Send Scale Regression.vi"("Read CSV"=TRUE, "Message Enqueuer in"=w75) -> ()  [unwired: 8 in, 2 out]
        n51 = control-ref of="Calibrate Transducers"() -> (w83:refnum<vi>)
        n52 = control-ref of="Collect MVC"() -> (w81:refnum<vi>)
        n53 = Build Array(w84, w83, w82, w81, w80) -> (w79:refnum<vi>[])
        n54 = for {
          tunnel: w79 -> [w93] mode=indexing
          tunnel: w78 -> [w94]
          n55 = property class="Bool"(reference=w93, "Colors [4]"=w94) -> ()  [unwired: 1 in, 2 out]
        }
        n56 = for {
          tunnel: w85 -> [w97]
          tunnel: w78 -> [w96]
          tunnel: i32[] [0, 1, 2, 3, 6] -> [w95] mode=indexing
          n57 = in-place {
            in-place-border: w96 -> [w101]
            w99 = refnum<vi> refnum  # Control
            w104 = refnum<vi> refnum  # Boolean
            n58 = in-place-array #2(w97, w95) -> (w105:refnum<vi>)
            n59 = To More Specific Class(target class=w104, reference=w105) -> (specific class reference=w103:refnum<vi>, error out=w102:errorcluster)  [unwired: 1 in]
            n60 = property class="Bool"(reference=w103, error in=w102, "Colors [4]"=w101) -> (reference out=w100:refnum<vi>)  [unwired: 1 out]
            n61 = To More Generic Class(target class=w99, reference=w100) -> (generic class reference=w98:refnum<vi>)
            n62 = in-place-array #2(w98) -> ()  [unwired: 2 out]
          }
        }
        n63 = property on="Auto Clust" class="Clust (strict)"() -> ("Controls[]"=w87:refnum<vi>[])  [unwired: 2 in, 2 out]
        n64 = property on="Task Selection" class="Clust (strict)"() -> ("Controls[]"=w90:refnum<vi>[])  [unwired: 2 in, 2 out]
        n65 = in-place {
          n66 = in-place-array #3(w90, 0, 1) -> (w117:refnum<vi>, w108:refnum<vi>)
          n67 = in-place-array #4(w87, 0) -> (w114:refnum<vi>)
          n68 = property class="Ctl"(reference=w114) -> (reference out=w113:refnum<vi>, "Value"=w111:variant)  [unwired: 1 in, 1 out]
          n69 = property class="Ctl"(reference=w117) -> (reference out=w116:refnum<vi>, "Value"=w115:variant)  [unwired: 1 in, 1 out]
          n70 = property class="Ctl"(reference=w108) -> (reference out=w109:refnum<vi>, "Value"=w110:variant)  [unwired: 1 in, 1 out]
          n71 = property class="Ctl"(reference=w113, "Val(Sgnl)"=w111) -> (reference out=w112:refnum<vi>)  [unwired: 1 in, 1 out]
          n72 = property class="Ctl"(reference=w116, "Val(Sgnl)"=w115) -> (reference out=w107:refnum<vi>)  [unwired: 1 in, 1 out]
          n73 = property class="Ctl"(reference=w109, "Val(Sgnl)"=w110) -> (reference out=w106:refnum<vi>)  [unwired: 1 in, 1 out]
          n74 = in-place-array #3(w107, w106) -> ()  [unwired: 3 out]
          n75 = in-place-array #4(w112) -> ()  [unwired: 2 out]
        }
        n76 = property on="Task Start" class="Bool"("Colors [4]"=cluster{u32, u32}[] [{50176, 50176}, {50176, 50176}, {6618880, 6618880}]) -> ()  [unwired: 2 in, 2 out]
        n77 = property on="Abort Task" class="Bool"("Colors [4]"=cluster{u32, u32}[] [{16711680, 16711680}, {16711680, 16711680}, {16711680, 16711680}]) -> ()  [unwired: 2 in, 2 out]
      }
      event Value Change {
        n78 = event-data() -> ("NewVal"=w120:bool)  [unwired: 1 in]
        n79 = case shown="False" w120 {
          tunnel: [T17."Disabled and Grayed Out" ("Disabled") T17."Enabled" ("Disabled")] -> w118
          frame False {
          }
          frame True {
          }
        }
        n80 = for {
          N: 8 -> [_]
          tunnel: w118 -> [w123]
          i -> [w124]
          n81 = Increment(x=w124) -> (x+1=w125:i32)
          n82 = property on="EMG Master Config" class="Clust (strict)"() -> ("Controls[]"=w126:refnum<vi>[])  [unwired: 2 in, 2 out]
          n83 = in-place {
            in-place-border: w123 -> [w127]
            n84 = in-place-array #5(w126, w125) -> (w129:refnum<vi>)
            n85 = property class="Ctl"(reference=w129, "DisabledEnum"=w127) -> (reference out=w128:refnum<vi>)  [unwired: 1 in, 1 out]
            n86 = in-place-array #5(w128) -> ()  [unwired: 2 out]
          }
        }
      }
      event Value Change {
        n87 = event-data() -> ("NewVal"=w131:u16, "OldVal"=w132:u16)  [unwired: 1 in]
        n88 = call "Send Update Patterns Array.vi"("Old Num of Parabolas"=w132, "Num of Parabolas"=w131, "Message Enqueuer in"=w130) -> ()  [unwired: 7 in, 2 out]
      }
      event User Event {
        n89 = event-data() -> ("Patterns Array"=w135:u8[][], "Phase Array"=w133:i32[][])  [unwired: 1 in]
        n90 = Bundle By Name(cluster="Auto Clust", "Patterns Array"=w135, "Phase Array"=w133) -> (w134:T11)
        n91 = property on="Auto Clust" class="Clust (strict)"("Value"=w134) -> ()  [unwired: 2 in, 2 out]
      }
      event "Calc Regression": Value Change {
        n92 = event-data() -> ()  [unwired: 1 in, 1 out]
        n93 = call "Send Scale Regression.vi"("Read CSV"=FALSE, "TScale Calibration"="TScale Calibration", "Message Enqueuer in"=w139) -> ()  [unwired: 7 in, 2 out]
      }
      event User Event {
        n94 = event-data() -> ("Slope Int"=→"Slope Int":dbl[][])  [unwired: 1 in]
      }
      event "Config Select": Value Change {
        n95 = event-data() -> ("NewVal"=w149:string)  [unwired: 1 in, 5 out]
        n96 = control-ref of="Task Selection"() -> (w146:refnum<vi>)
        n97 = property on="Adjusted MVC (N)" class="DigNum (strict)"() -> (error out=w141:errorcluster, "Value"=→"MVC Temp":dbl)  [unwired: 2 in, 1 out]
        n98 = control-ref of="Auto Clust"() -> (w144:refnum<vi>)
        n99 = control-ref of="Config Select"() -> (w145:refnum<vi>)
        n100 = control-ref of="Task Info Cluster"() -> (w147:refnum<vi>)
        n101 = case shown="\"False\", Default" w149 {
          selector: w149 -> [w157 _]
          tunnel: w148 -> [w158 w164]
          tunnel: w147 -> [w153 w163]
          tunnel: w146 -> [w154 w161]
          tunnel: w145 -> [w152 w160]
          tunnel: w144 -> [w155 w159]
          tunnel: w143 -> [w151 _]
          tunnel: w141 -> [w150 _]
          frame "False", Default {
            n102 = call "Send Save or Load Config.vi"("GUI Helper Q"=w151, "Config Select Ref"=w152, "Task Info in"=w153, "Save?"=FALSE, "Auto Clust"=w155, "error in (no error)"=w150, "Task Configuration Name"=w157, "Task Selection in"=w154, "Message Enqueuer in"=w158) -> ()  [unwired: 1 in, 2 out]
          }
          frame "Create New..." {
            n103 = call "Create New Task Configuration"() -> ("Task Configuration Name"=w162:string, "OK"=w165:bool)  [unwired: 17 in, 1 out]
            n104 = case shown="True" w165 {
              tunnel: w164 -> [_ w172]
              tunnel: w163 -> [_ w168]
              tunnel: w162 -> [_ w171]
              tunnel: w161 -> [_ w167]
              tunnel: w160 -> [_ w166]
              tunnel: w159 -> [_ w169]
              frame False {
              }
              frame True {
                n105 = call "Send Save or Load Config.vi"("Config Select Ref"=w166, "Task Info in"=w168, "Save?"=TRUE, "Auto Clust"=w169, "Task Configuration Name"=w171, "Task Selection in"=w167, "Message Enqueuer in"=w172) -> ()  [unwired: 3 in, 2 out]
              }
            }
          }
        }
      }
      event User Event {
        n106 = event-data() -> ("Config Array"=w175:string[][])  [unwired: 1 in, 4 out]
        n107 = Index Array(array=w175, index (row)=0) -> (element=w173:string[])  [unwired: 1 in]
        n108 = property on="Config Select" class="CmbBox"("Strings[]"=w173) -> ()  [unwired: 2 in, 2 out]
      }
      event "Delete Config": Value Change {
        n109 = event-data() -> ()  [unwired: 1 in, 6 out]
        n110 = property on="Config Select" class="CmbBox"() -> ("Value"=w178:string)  [unwired: 2 in, 2 out]
        n111 = Equal?(x="Create New...", y=w178) -> (x = y?=w176:bool)
        n112 = case shown="False" w176 {
          tunnel: w179 -> [w181 _]
          tunnel: w178 -> [w180 _]
          frame False {
            n113 = Two Button Dialog(message="Are you sure you would like to delete this task configuration setting?", 1:"No" ("F button name (\"Cancel\")"), 2:"Yes" ("T button name (\"OK\")")) -> (T button?=w182:bool)
            n114 = case shown="True" w182 {
              tunnel: w181 -> [_ w188]
              tunnel: w180 -> [_ w186]
              frame False {
              }
              frame True {
                n115 = control-ref of="Config Select"() -> (w187:refnum<vi>)
                n116 = call "Send Delete Config.vi"("Config Selected"=w186, "Config Select Ref"=w187, "Message Enqueuer in"=w188) -> ()  [unwired: 7 in, 2 out]
              }
            }
          }
          frame True {
          }
        }
      }
      event Value Change {
        # "9: Lissajous speed control"
        n117 = event-data() -> ("NewVal"=w195:enum32{"Frequency Task", "Scanning Task"})  [unwired: 1 in]
        n118 = case shown="\"Scanning Task\"" w195 {
          tunnel: [T17."Disabled and Grayed Out" ("Disabled") T17."Enabled" ("Disabled")] -> w193
          frame "Frequency Task", Default {
          }
          frame "Scanning Task" {
          }
        }
        n119 = property on="Task Info Cluster" class="Clust (strict)"() -> ("Controls[]"=w194:refnum<vi>[])  [unwired: 2 in, 2 out]
        n120 = Index Array(array=w194, index=9) -> (element=w191:refnum<vi>)
        n121 = property class="Ctl"(reference=w191, "DisabledEnum"=w193) -> (error out=w190:errorcluster)  [unwired: 1 in, 1 out]
        n122 = call "Send Task Type Change.vi"("error in (no error)"=w190, "Message Enqueuer in"=w189) -> ()  [unwired: 8 in, 2 out]
      }
      event Value Change {
        # "1: Sampling rate control\n3: MVC/Scaling control\n9: Lissajous speed control"
        n123 = event-data() -> ("NewVal"=w205:enum32{"Force Input", "Movement Input"})  [unwired: 1 in]
        n124 = case shown="\"Movement Input\"" w205 {
          tunnel: ["Adjusted MVC (N)" ("Caption.Text") "Scaling Factor" ("Caption.Text")] -> w199
          tunnel: ["Force\nSampling Rate (Hz)" ("Caption.Text") "Potentiometer\nSampling Rate (Hz)" ("Caption.Text")] -> w198
          frame "Force Input", Default {
          }
          frame "Movement Input" {
          }
        }
        n125 = property on="Task Info Cluster" class="Clust (strict)"() -> ("Controls[]"=w204:refnum<vi>[])  [unwired: 2 in, 2 out]
        n126 = Index Array(array=w204, index #1=1 ("index"), index #2=3 ("index")) -> (element #1=w202:refnum<vi>, element #2=w200:refnum<vi>)  [unwired: 1 in, 1 out]
        n127 = property class="Ctl"(reference=w202, "Caption.Text"=w198) -> ()  [unwired: 1 in, 2 out]
        n128 = property class="Ctl"(reference=w200, "Caption.Text"=w199) -> ()  [unwired: 1 in, 2 out]
      }
      event Value Change {
        n129 = event-data() -> ("NewVal"=w236:bool)  [unwired: 1 in]
        n130 = local read "Task Selection"() -> (w213:T3)
        n131 = Unbundle By Name(w213) -> ("Task Type Select"=w212:enum32{"Frequency Task", "Scanning Task"})
        n132 = case shown="False" w236 {
          tunnel: [w238 w243] -> w214
          tunnel: [w237 w242] -> w217
          tunnel: w212 -> [_ w241]
          tunnel: [w238 w240] -> w211
          tunnel: [w237 w239] -> w210
          frame False {
            w237 = T17."Enabled" ("Disabled")
            w238 = T17."Disabled and Grayed Out" ("Disabled")
          }
          frame True {
            n133 = case shown="\"Scanning Task\"" w241 {
              tunnel: [w245 w246] -> w243
              tunnel: [w244 w247] -> w242
              tunnel: [w245 w247] -> w240
              tunnel: [w244 w246] -> w239
              frame "Frequency Task", Default {
                w244 = T17."Disabled and Grayed Out" ("Disabled")
                w245 = T17."Enabled" ("Disabled")
              }
              frame "Scanning Task" {
                w247 = T17."Disabled and Grayed Out" ("Disabled")
                w246 = T17."Enabled" ("Disabled")
              }
            }
          }
        }
        n134 = property on="Task Info Cluster" class="Clust (strict)"() -> ("Controls[]"=w230:refnum<vi>[])  [unwired: 2 in, 2 out]
        n135 = property on="Auto Clust" class="Clust (strict)"() -> ("Controls[]"=w235:refnum<vi>[])  [unwired: 2 in, 2 out]
        n136 = Index Array(array=w235, index #1=1 ("index"), index #2=2 ("index"), index #3=3 ("index")) -> (element #1=w232:refnum<vi>, element #2=w231:refnum<vi>, element #3=w215:refnum<vi>)
        n137 = Index Array(array=w230, index #1=0 ("index"), index #2=4 ("index"), index #3=5 ("index"), index #4=6 ("index"), index #5=7 ("index"), index #6=8 ("index")) -> (element #1=w223:refnum<vi>, element #2=w222:refnum<vi>, element #3=w221:refnum<vi>, element #4=w220:refnum<vi>, element #5=w219:refnum<vi>, element #6=w218:refnum<vi>)
        n138 = property class="Ctl"(reference=w215, "DisabledEnum"=w211) -> ()  [unwired: 1 in, 2 out]
        n139 = property class="Ctl"(reference=w232, "DisabledEnum"=w214) -> ()  [unwired: 1 in, 2 out]
        n140 = property class="Ctl"(reference=w231, "DisabledEnum"=w211) -> ()  [unwired: 1 in, 2 out]
        n141 = property class="Ctl"(reference=w218, "DisabledEnum"=w217) -> ()  [unwired: 1 in, 2 out]
        n142 = property class="Ctl"(reference=w220, "DisabledEnum"=w210) -> ()  [unwired: 1 in, 2 out]
        n143 = property class="Ctl"(reference=w219, "DisabledEnum"=w210) -> ()  [unwired: 1 in, 2 out]
        n144 = property class="Ctl"(reference=w223, "DisabledEnum"=w217) -> ()  [unwired: 1 in, 2 out]
        n145 = property class="Ctl"(reference=w222, "DisabledEnum"=w210) -> ()  [unwired: 1 in, 2 out]
        n146 = property class="Ctl"(reference=w221, "DisabledEnum"=w210) -> ()  [unwired: 1 in, 2 out]
      }
      event User Event {
        n147 = event-data() -> ("Item Names"=w248:string[][])  [unwired: 1 in]
        n148 = property on="Marker List" class="MCListbox (strict)"("ItemNames"=w248) -> ()  [unwired: 2 in, 2 out]
      }
      event Mouse Down {
        n149 = event-data() -> ("CtlRef"=w256:refnum<vi>, "Coords"=w255:T19)  [unwired: 1 in, 3 out]
        n150 = invoke class="MCListbox (strict)" method="Point To Row Column"(reference=w256, "Point"=w255) -> ("InBounds"=w252:bool, "CellPosition"=w254:T20)  [unwired: 5 in, 5 out]
        n151 = Unbundle By Name(w254) -> ("Row"=w253:i32)
        n152 = Bundle("InBounds"=w252, "Row"=w253) -> (w250:cluster{"InBounds":bool, "Row":i32})  [unwired: 1 in]
        n153 = call "Send Accel Marker Update.vi"("Listbox info"=w250, "Select Active Row"=TRUE, "Message Enqueuer in"=w251) -> ()  [unwired: 7 in, 2 out]
      }
      event Value Change {
        n154 = event-data() -> ()  [unwired: 1 in, 6 out]
        n155 = property on="Task Previewed?" class="Bool (strict)"() -> ("Value"=w257:bool)  [unwired: 2 in, 2 out]
        n156 = case shown="True" w257 {
          tunnel: w258 -> [_ w259]
          frame False {
          }
          frame True {
            n157 = call "Send Set Template Data.vi"("Message Enqueuer in"=w259) -> ()  [unwired: 9 in, 2 out]
          }
        }
      }
      event "Calibrate Transducers": Value Change {
        n158 = event-data() -> ()  [unwired: 1 in, 6 out]
        n159 = Enqueue Element(queue=w261, element=Task_Active_Enum_df."Calibrate Force") -> ()  [unwired: 2 in, 3 out]
      }
      event "Calibrate Pot": Value Change {
        n160 = event-data() -> ()  [unwired: 1 in, 1 out]
        n161 = Enqueue Element(queue=w263, element=Task_Active_Enum_df."Calibrate Potentiometers") -> ()  [unwired: 2 in, 3 out]
      }
      event "Collect MVC": Value Change {
        n162 = event-data() -> ()  [unwired: 1 in, 6 out]
        n163 = call "Send MVC Collect File Check.vi"("GUI helper Q"=w264, "Message Enqueuer in"=w265) -> ()  [unwired: 8 in, 2 out]
      }
      event User Event {
        n164 = event-data() -> ("Left"=w269:dbl, "Right"=w268:dbl)  [unwired: 1 in, 4 out]
        n165 = in-place {
          in-place-border: w269 -> [w275]
          in-place-border: w268 -> [w274]
          in-place-border: [w271] -> w266
          w277 = 0.01 ("value")
          n166 = in-place-cluster #6("MVC Cluster input") -> ("MVC Percent"=w276:u8)
          n167 = Compound Arithmetic op=MULTIPLY(w277, w276, w275) -> (w273:dbl)
          n168 = Compound Arithmetic op=MULTIPLY(w277, w276, w274) -> (w272:dbl)
          n169 = in-place-cluster #6("MVC Percent"=w276) -> ()  [unwired: 1 out]
          n170 = Bundle(w273, w272) -> (w271:cluster{dbl, dbl})  [unwired: 1 in]
        }
        n171 = Bundle("Left"=w269, "Right"=w268) -> (→"Raw MVC Clust":cluster{"Left":dbl, "Right":dbl})  [unwired: 1 in]
        n172 = property on="Adjusted MVC Cluster" class="Clust (strict)"("Val(Sgnl)"=w266) -> ()  [unwired: 2 in, 2 out]
      }
      event "MVC Cluster input.MVC Percent": Value Change {
        n173 = event-data() -> ("NewVal"=w279:u8)  [unwired: 1 in]
        n174 = property on="Raw MVC Clust" class="Clust (strict)"() -> ("Value"=w280:cluster{"Raw MVC Left":dbl, "Raw MVC Right":dbl})  [unwired: 2 in, 2 out]
        n175 = in-place {
          in-place-border: w279 -> [w286]
          in-place-border: [w281] -> w278
          w287 = 0.01 ("value")
          n176 = in-place-cluster #7(w280) -> ("Raw MVC Left"=w285:dbl, "Raw MVC Right"=w284:dbl)
          n177 = Compound Arithmetic op=MULTIPLY(w287, w286, w285) -> (w283:dbl)
          n178 = Compound Arithmetic op=MULTIPLY(w287, w286, w284) -> (w282:dbl)
          n179 = in-place-cluster #7("Raw MVC Left"=w285, "Raw MVC Right"=w284) -> ()  [unwired: 1 out]
          n180 = Bundle(w283, w282) -> (w281:cluster{dbl, dbl})  [unwired: 1 in]
        }
        "Adjusted MVC Cluster" <- w278
      }
      event "Task Start": Value Change {
        n181 = event-data() -> ()  [unwired: 1 in, 1 out]
        n182 = Unbundle By Name("EMG Master Config") -> ("EMG Master"=w288:bool)
        n183 = call "Send Does File Exist.vi"("GUI helper Q"=w290, "EMG Mode"=w288, "Message Enqueuer in"=w291) -> ()  [unwired: 7 in, 2 out]
      }
      event User Event {
        n184 = event-data() -> ("Trial Num"=→"Trial Num":i32)  [unwired: 1 in]
      }
      event Value Change {
        n185 = event-data() -> ("CtlRef"=w298:refnum<vi>)  [unwired: 1 in, 2 out]
        n186 = property class="Bool"(reference=w298) -> (error out=w295:errorcluster, "Caption.Text"=w296:string)  [unwired: 1 in, 1 out]
        n187 = call "Send Accel Marker Update.vi"("Marker Enum"=Marker_Enum."Predefined", "error in (no error)"=w295, "Select Active Row"=FALSE ("Custom Marker?"), "Marker Name"=w296, "Message Enqueuer in"=w297) -> ()  [unwired: 5 in, 2 out]
      }
      event Value Change {
        n188 = event-data() -> ("CtlRef"=w300:refnum<vi>)  [unwired: 1 in]
        n189 = property class="Bool"(reference=w300) -> (error out=w303:errorcluster, "Caption.Text"=w304:string)  [unwired: 1 in, 1 out]
        n190 = call "Send Accel Marker Update.vi"("Marker Enum"=Marker_Enum."Custom", "error in (no error)"=w303, "Select Active Row"=FALSE ("Custom Marker?"), "Marker Name"=w304, "Message Enqueuer in"=w301) -> ()  [unwired: 5 in, 2 out]
      }
      event Value Change {
        n191 = event-data() -> ()  [unwired: 1 in, 6 out]
        n192 = call "Send Accel Marker Update.vi"("Marker Enum"=Marker_Enum."Delete Row", "Select Active Row"=FALSE, "Message Enqueuer in"=w307) -> ()  [unwired: 7 in, 2 out]
      }
      event Key Down {
        n193 = event-data() -> ("Char"=w309:i16)  [unwired: 1 in, 2 out]
        n194 = case shown="48" w309 {
          tunnel: w308 -> [w312 w316 w319 _]
          frame 48 {
            # "Partial g marker"
            n195 = call "Send Accel Marker Update.vi"("Marker Enum"=Marker_Enum."Predefined", "Select Active Row"=FALSE, "Marker Name"="Partial g", "Message Enqueuer in"=w312) -> ()  [unwired: 6 in, 2 out]
          }
          frame 49 {
            # "1 g marker"
            n196 = call "Send Accel Marker Update.vi"("Marker Enum"=Marker_Enum."Predefined", "Marker Name"="1 g", "Message Enqueuer in"=w316) -> ()  [unwired: 7 in, 2 out]
          }
          frame 50 {
            # "Hyper g marker"
            n197 = call "Send Accel Marker Update.vi"("Marker Enum"=Marker_Enum."Predefined", "Marker Name"="Hyper g", "Message Enqueuer in"=w319) -> ()  [unwired: 7 in, 2 out]
          }
          frame 51, Default {
          }
        }
      }
      event "Abort Task": Value Change {
        n198 = event-data() -> ()  [unwired: 1 in, 6 out]
        n199 = Two Button Dialog(message="Are you sure you want to abort data collection? This will stop all data collection trials. ", 1:"Cancel" ("F button name (\"Cancel\")"), 2:"Yes" ("T button name (\"OK\")")) -> (T button?=w320:bool)
        n200 = case shown="True" w320 {
          selector: w320 -> [_ w324]
          frame False {
          }
          frame True {
            n201 = local write "Abort Signal"(w324) -> ()
          }
        }
      }
      event "Task window closed?": Value Change {
        n202 = event-data() -> ("NewVal"=w325:bool)  [unwired: 1 in]
        n203 = case shown="True" w325 {
          selector: w325 -> [w326 w327]
          frame False {
            n204 = local write "Abort Signal"(w326) -> ()
          }
          frame True {
            n205 = local write "Abort Signal"(w327) -> ()
          }
        }
      }
      event "Preview Task": Value Change {
        n206 = event-data() -> ()  [unwired: 1 in, 6 out]
        n207 = Enqueue Element(queue=w329, element=Task_Active_Enum_df."Preview Template") -> ()  [unwired: 2 in, 3 out]
      }
      event Panel Close? {
        n208 = event-data() -> ()  [unwired: 1 in, 1 out]
        n209 = control-ref of="This VI"() -> (w331:refnum<vi>)
        n210 = call <userlib>:"Write Panel to INI__ogtk.vi"("VI ref"=w331, "refnum"=w332) -> ("error out"=w330:errorcluster)  [unwired: 8 in, 1 out]
        n211 = call <vilib>:"Send Normal Stop.vi"("error in (no error)"=w330, "Message Enqueuer"=w334) -> ()  [unwired: 9 in, 1 out]
        n212 = event-data("Discard?"=TRUE) -> ()  [unwired: 1 in, 1 out]
      }
      event User Event {
        n213 = event-data() -> ()  [unwired: 1 in, 1 out]
        n214 = flat-sequence {
          tunnel: w336 -> [w338]
          tunnel: [TRUE] -> w335
          frame #0 {
            n215 = Enqueue Element(queue=w338, element=Task_Active_Enum_df."Stop Helper") -> ()  [unwired: 2 in, 3 out]
          }
          frame #1 {
          }
        }
      }
    }
  }
  n216 = while {
    tunnel: w22 -> [w345]
    tunnel: w24 -> [w343]
    tunnel: w23 -> [w342]
    tunnel: [w340] -> w21
    stop <- w344 stop-if-true
    n217 = Dequeue Element(queue=w343, error in (no error)=w342) -> (queue out=w340:refnum<queue>, element=w341:T13)  [unwired: 1 in, 2 out]
    n218 = case shown="\"EMG Mode\"" w341 {
      tunnel: w345 -> [w347 w381 w426 w469 w521 w537 w840 w1223 w1515 w1898 w2143 _ _]
      tunnel: [FALSE _ _ _ _ _ _ _ _ _ _ TRUE _] -> w344
      tunnel: w340 -> [_ w358 w403 w449 w509 w557 w862 w1243 w1539 w1907 w2168 _ _]
      frame "Idle", Default {
        n219 = in-place {
          in-place-border: [w349] -> w346
          w351 = FALSE ("Value (Signaling)")
          n220 = in-place-cluster #8(w347) -> ("Task window closed?"=w355:refnum<vi>, "Task window update"=w353:refnum<user-event>)
          n221 = property class="Bool (strict)"(reference=w355, "Val(Sgnl)"=w351) -> (reference out=w354:refnum<vi>, error out=w350:errorcluster)  [unwired: 1 in]
          n222 = Generate User Event(user event=w353, event data cluster=w351, error in=w350) -> (user event out=w352:refnum<user-event>, error out=w349:errorcluster)  [unwired: 1 in]
          n223 = in-place-cluster #8("Task window closed?"=w354, "Task window update"=w352) -> ()  [unwired: 1 out]
        }
        n224 = call <vilib>:"Simple Error Handler.vi"("error in (no error)"=w346) -> ()  [unwired: 4 in, 5 out]
      }
      frame "Calibrate Force" {
        w356 = FALSE ("Stop Acquiring")
        w379 = refnum<class "NI Force Task.lvclass"> refnum  # Force Task
        n225 = call <vilib>:"Set Busy.vi"("disable click? (T)"=FALSE) -> ("error out"=w362:errorcluster)  [unwired: 9 in, 1 out]
        n226 = call-poly <vilib>:"Panel Type Selector.vi"("Autoshow? (T)"=FALSE, "Default Title"="Calibration") -> ("Window out"=w380:refnum<class "Window.lvclass">)  [unwired: 8 in, 1 out]
        n227 = call <vilib>:"Launch Nested Panel.vi"("Panel"=w380, "Nested Panel Actor"=w379, "Panel Actor in"=w381) -> ("Nested Actor's Enqueuer"=w366:refnum<class "Message Enqueuer.lvclass">, "Panel Actor out"=w378:refnum<class "GUI.lvclass">)  [unwired: 5 in, 2 out]
        n228 = in-place {
          in-place-border: [w396] -> w377
          in-place-border: [w394] -> w376
          in-place-border: [w393] -> w375
          n229 = in-place-cluster #9(w378) -> ("Force Calibration Input Cluster"=w400:refnum<vi>, "DAQ Physical Channels"=w398:refnum<vi>)
          n230 = property class="Clust (strict)"(reference=w400) -> (reference out=w399:refnum<vi>, "Value"=w395:T7)  [unwired: 1 in, 1 out]
          n231 = property class="Clust (strict)"(reference=w398) -> (reference out=w397:refnum<vi>, "Value"=w396:T9)  [unwired: 1 in, 1 out]
          n232 = Unbundle By Name(w395) -> ("Force Calib Sampling Rate"=w394:u16, "Force Calib Duration"=w393:u8)
          n233 = in-place-cluster #9("Force Calibration Input Cluster"=w399, "DAQ Physical Channels"=w397) -> ()  [unwired: 1 out]
        }
        n234 = call "Send Stop Trial.vi"("DAQ Task"=w356, "Stop Acquiring"=w356, "Message Enqueuer in"=w366) -> ("error out"=w365:errorcluster, "Message Enqueuer out"=w367:refnum<class "Message Enqueuer.lvclass">)  [unwired: 7 in]
        n235 = call "Send Calibrate Force.vi"("error in (no error)"=w365, "DAQ  Channels In"=w377, "rate"=w376, "Message Enqueuer in"=w367) -> ("error out"=w371:errorcluster, "Message Enqueuer out"=w373:refnum<class "Message Enqueuer.lvclass">)  [unwired: 6 in]
        n236 = flat-sequence {
          tunnel: w375 -> [w385]
          tunnel: [w384] -> w374
          tunnel: w373 -> [w384]
          tunnel: [w383] -> w372
          tunnel: w371 -> [w383]
          tunnel: w362 -> [w382]
          tunnel: [w382] -> w361
          tunnel: w374 -> [w392]
          tunnel: w372 -> [w391]
          tunnel: [w390] -> w370
          tunnel: [w389] -> w369
          tunnel: [w386] -> w360
          tunnel: w361 -> [w386]
          frame #0 {
            n237 = call "Time Delay4"("Delay Time (s)"=w385) -> ()  [unwired: 10 in, 1 out]
          }
          frame #1 {
            n238 = Wait (ms)(milliseconds to wait=u32 100) -> ()  [unwired: 1 out]
            n239 = call "Send Stop Trial.vi"("error in (no error)"=w391, "Stop Acquiring"=TRUE, "Message Enqueuer in"=w392) -> ("error out"=w389:errorcluster, "Message Enqueuer out"=w390:refnum<class "Message Enqueuer.lvclass">)  [unwired: 7 in]
          }
        }
        n240 = call "Send External Shutdown.vi"("error in (no error)"=w369, "Message Enqueuer in"=w370) -> ("error out"=w357:errorcluster)  [unwired: 8 in, 1 out]
        n241 = call <vilib>:"Unset Busy.vi"("error in (no error)"=w360) -> ()  [unwired: 10 in, 1 out]
        n242 = Enqueue Element(queue=w358, element=Task_Active_Enum_df."Idle", error in (no error)=w357) -> ()  [unwired: 1 in, 3 out]
      }
      frame "Calibrate Potentiometers" {
        w401 = FALSE ("Stop Acquiring")
        w424 = refnum<class "NI Force Task.lvclass"> refnum  # Force Task
        n243 = call <vilib>:"Set Busy.vi"("disable click? (T)"=FALSE) -> ("error out"=w407:errorcluster)  [unwired: 9 in, 1 out]
        n244 = call-poly <vilib>:"Panel Type Selector.vi"("Autoshow? (T)"=FALSE, "Default Title"="Calibration") -> ("Window out"=w425:refnum<class "Window.lvclass">)  [unwired: 8 in, 1 out]
        n245 = call <vilib>:"Launch Nested Panel.vi"("Panel"=w425, "Nested Panel Actor"=w424, "Panel Actor in"=w426) -> ("Nested Actor's Enqueuer"=w411:refnum<class "Message Enqueuer.lvclass">, "Panel Actor out"=w423:refnum<class "GUI.lvclass">)  [unwired: 5 in, 2 out]
        n246 = in-place {
          in-place-border: [w441] -> w422
          in-place-border: [w439] -> w421
          in-place-border: [w438] -> w420
          n247 = in-place-cluster #10(w423) -> ("Pot Calibration Input Clust"=w445:refnum<vi>, "DAQ Physical Channels"=w443:refnum<vi>)
          n248 = property class="Clust (strict)"(reference=w445) -> (reference out=w444:refnum<vi>, "Value"=w440:T7)  [unwired: 1 in, 1 out]
          n249 = property class="Clust (strict)"(reference=w443) -> (reference out=w442:refnum<vi>, "Value"=w441:T9)  [unwired: 1 in, 1 out]
          n250 = Unbundle By Name(w440) -> ("Force Calib Sampling Rate"=w439:u16, "Force Calib Duration"=w438:u8)
          n251 = in-place-cluster #10("Pot Calibration Input Clust"=w444, "DAQ Physical Channels"=w442) -> ()  [unwired: 1 out]
        }
        n252 = call "Send Stop Trial.vi"("DAQ Task"=w401, "Stop Acquiring"=w401, "Message Enqueuer in"=w411) -> ("error out"=w410:errorcluster, "Message Enqueuer out"=w412:refnum<class "Message Enqueuer.lvclass">)  [unwired: 7 in]
        n253 = call "Send Calibrate Potentiometers.vi"("error in (no error)"=w410, "rate"=w421, "DAQ  Channels In"=w422, "Message Enqueuer in"=w412) -> ("error out"=w416:errorcluster, "Message Enqueuer out"=w418:refnum<class "Message Enqueuer.lvclass">)  [unwired: 6 in]
        n254 = flat-sequence {
          tunnel: w420 -> [w430]
          tunnel: [w429] -> w419
          tunnel: w418 -> [w429]
          tunnel: [w428] -> w417
          tunnel: w416 -> [w428]
          tunnel: w407 -> [w427]
          tunnel: [w427] -> w406
          tunnel: w419 -> [w437]
          tunnel: w417 -> [w436]
          tunnel: [w435] -> w415
          tunnel: [w434] -> w414
          tunnel: [w431] -> w405
          tunnel: w406 -> [w431]
          frame #0 {
            n255 = call "Time Delay6"("Delay Time (s)"=w430) -> ()  [unwired: 10 in, 1 out]
          }
          frame #1 {
            n256 = Wait (ms)(milliseconds to wait=u32 100) -> ()  [unwired: 1 out]
            n257 = call "Send Stop Trial.vi"("error in (no error)"=w436, "Stop Acquiring"=TRUE, "Message Enqueuer in"=w437) -> ("error out"=w434:errorcluster, "Message Enqueuer out"=w435:refnum<class "Message Enqueuer.lvclass">)  [unwired: 7 in]
          }
        }
        n258 = call "Send External Shutdown.vi"("error in (no error)"=w414, "Message Enqueuer in"=w415) -> ("error out"=w402:errorcluster)  [unwired: 8 in, 1 out]
        n259 = call <vilib>:"Unset Busy.vi"("error in (no error)"=w405) -> ()  [unwired: 10 in, 1 out]
        n260 = Enqueue Element(queue=w403, element=Task_Active_Enum_df."Idle", error in (no error)=w402) -> ()  [unwired: 1 in, 3 out]
      }
      frame "Collect MVC" {
        w446 = FALSE ("Stop Acquiring")
        w471 = refnum<class "NI Force Task.lvclass"> refnum  # Force Task
        n261 = call <vilib>:"Application Directory.vi"() -> ("Application Directory"=w458:path)
        n262 = Build Path(base path=w458, name or relative path=path "temp_ni.tdms") -> (appended path=w459:path)
        n263 = TDMS Open(10:T21."create or replace" ("operation (0:open)"), 11:w459) -> (3:w452:refnum<k34>)  [unwired: 5 in, 1 out]
        n264 = call-poly <vilib>:"Panel Type Selector.vi"("Autoshow? (T)"=FALSE, "Default Title"="MVC") -> ("Window out"=w473:refnum<class "Window.lvclass">)  [unwired: 8 in, 1 out]
        n265 = call <vilib>:"Launch Nested Panel.vi"("Panel"=w473, "Nested Panel Actor"=w471, "Panel Actor in"=w469) -> ("Nested Actor's Enqueuer"=w467:refnum<class "Message Enqueuer.lvclass">, "Panel Actor out"=w470:refnum<class "GUI.lvclass">)  [unwired: 5 in, 2 out]
        n266 = in-place {
          in-place-border: [w503] -> w468
          in-place-border: [w501] -> w451
          in-place-border: [w500] -> w474
          in-place-border: w452 -> [w499]
          in-place-border: [w498] -> w454
          in-place-border: [w495] -> w453
          in-place-border: [w492] -> w450
          n267 = in-place-cluster #11(w470) -> ("MVC Cluster"=w507:refnum<vi>, "DAQ Physical Channels"=w505:refnum<vi>, "Logger"=w498:refnum<class "Message Enqueuer.lvclass">, "Final File Path"=w497:refnum<vi>, "Force Calibration Cluster"=w494:refnum<vi>)  [unwired: 1 out]
          n268 = property class="Clust (strict)"(reference=w507) -> (reference out=w506:refnum<vi>, "Value"=w502:T5)  [unwired: 1 in, 1 out]
          n269 = property class="Clust (strict)"(reference=w505) -> (reference out=w504:refnum<vi>, "Value"=w503:T9)  [unwired: 1 in, 1 out]
          n270 = property class="Clust (strict)"(reference=w494) -> (reference out=w493:refnum<vi>, "Value"=w492:cluster{"Left":dbl, "Right":dbl})  [unwired: 1 in, 1 out]
          n271 = property class="Path"(reference=w497) -> (reference out=w496:refnum<vi>, "Value"=w495:path)  [unwired: 1 in, 1 out]
          n272 = Unbundle By Name(w502) -> ("MVC Sampling Rate"=w501:u16, "MVC Duration"=w500:u8)
          n273 = in-place-cluster #11("Force TDMS File"=w499, "MVC Cluster"=w506, "DAQ Physical Channels"=w504, "Logger"=w498, "Final File Path"=w496, "Force Calibration Cluster"=w493) -> ()  [unwired: 1 out]
        }
        n274 = call "Send Stop Trial.vi"("DAQ Task"=w446, "Stop Acquiring"=w446, "Message Enqueuer in"=w467) -> ("error out"=w465:errorcluster, "Message Enqueuer out"=w466:refnum<class "Message Enqueuer.lvclass">)  [unwired: 7 in]
        n275 = call <vilib>:"Set Busy.vi"("disable click? (T)"=FALSE) -> ("error out"=w462:errorcluster)  [unwired: 9 in, 1 out]
        n276 = call "Send Collect MVC.vi"("Rate Hz"=w451, "Force Calibration Cluster"=w450, "error in (no error)"=w465, "TDMS file"=w452, "DAQ  Channels In"=w468, "Message Enqueuer in"=w466) -> ("error out"=w476:errorcluster, "Message Enqueuer out"=w475:refnum<class "Message Enqueuer.lvclass">)  [unwired: 4 in]
        n277 = flat-sequence {
          tunnel: w474 -> [w484]
          tunnel: [w483] -> w480
          tunnel: w475 -> [w483]
          tunnel: [w482] -> w479
          tunnel: w476 -> [w482]
          tunnel: [w481] -> w463
          tunnel: w462 -> [w481]
          tunnel: w480 -> [w491]
          tunnel: w479 -> [w490]
          tunnel: [w489] -> w477
          tunnel: [w488] -> w478
          tunnel: w463 -> [w485]
          tunnel: [w485] -> w461
          frame #0 {
            n278 = call "Time Delay5"("Delay Time (s)"=w484) -> ()  [unwired: 10 in, 1 out]
          }
          frame #1 {
            n279 = Wait (ms)(milliseconds to wait=u32 100) -> ()  [unwired: 1 out]
            n280 = call "Send Stop Trial.vi"("error in (no error)"=w490, "Stop Acquiring"=TRUE, "Message Enqueuer in"=w491) -> ("error out"=w488:errorcluster, "Message Enqueuer out"=w489:refnum<class "Message Enqueuer.lvclass">)  [unwired: 7 in]
          }
        }
        n281 = call "Send External Shutdown.vi"("error in (no error)"=w478, "Message Enqueuer in"=w477) -> ("error out"=w455:errorcluster)  [unwired: 8 in, 1 out]
        n282 = call <vilib>:"Unset Busy.vi"("error in (no error)"=w461) -> ()  [unwired: 10 in, 1 out]
        n283 = call "Send TDMS Cleanup.vi"("Force TDMS File"=w452, "error in (no error)"=w455, "TDMS File"=w453, "Message Enqueuer in"=w454) -> ("error out"=w448:errorcluster)  [unwired: 6 in, 1 out]
        n284 = Enqueue Element(queue=w449, element=Task_Active_Enum_df."Idle", error in (no error)=w448) -> ()  [unwired: 1 in, 3 out]
      }
      frame "Preview Template" {
        w523 = refnum<class "NI Force Task.lvclass"> refnum  # Force Task
        n285 = call-poly <vilib>:"Panel Type Selector.vi"("Default Title"="Task Preview") -> ("Window out"=w524:refnum<class "Window.lvclass">)  [unwired: 9 in, 1 out]
        n286 = call <vilib>:"Launch Nested Panel.vi"("Panel"=w524, "Nested Panel Actor"=w523, "Panel Actor in"=w521) -> ("Nested Actor's Enqueuer"=w518:refnum<class "Message Enqueuer.lvclass">, "Panel Actor out"=w519:refnum<class "GUI.lvclass">)  [unwired: 5 in, 2 out]
        n287 = in-place {
          in-place-border: w518 -> [w526]
          in-place-border: [w526] -> w513
          n288 = in-place-cluster #12(w519) -> ("NI Force Task"=w528:refnum<vi>)
          n289 = property class="LVClassControl (strict)"(reference=w528, "Val(Sgnl)"=w526) -> (reference out=w527:refnum<vi>, error out=w525:errorcluster)  [unwired: 1 in]
          n290 = call <vilib>:"Simple Error Handler.vi"("error in (no error)"=w525) -> ()  [unwired: 4 in, 5 out]
          n291 = in-place-cluster #12("NI Force Task"=w527) -> (w517:refnum<class "GUI.lvclass">)
        }
        n292 = property on="Task Previewed?" class="Bool (strict)"("Val(Sgnl)"=TRUE ("Value (Signaling)")) -> (error out=w511:errorcluster)  [unwired: 2 in, 1 out]
        n293 = call <vilib>:"Read Self Enqueuer.vi"("Actor"=w517) -> ("Self Enqueuer"=w520:refnum<class "Message Enqueuer.lvclass">)  [unwired: 10 in]
        n294 = call "Send Set Template Data.vi"("error in (no error)"=w511, "Message Enqueuer in"=w520) -> ("error out"=w516:errorcluster)  [unwired: 8 in, 1 out]
        n295 = while {
          tunnel: w516 -> [w531]
          tunnel: [w531] -> w515
          tunnel: w513 -> [w530]
          tunnel: [w530] -> w514
          stop <- "Task Previewed?" continue-if-true
        }
        n296 = call "Send External Shutdown.vi"("error in (no error)"=w515, "Message Enqueuer in"=w514) -> ("error out"=w508:errorcluster)  [unwired: 8 in, 1 out]
        n297 = Enqueue Element(queue=w509, element=Task_Active_Enum_df."Idle", error in (no error)=w508) -> ()  [unwired: 1 in, 3 out]
      }
      frame "Start Freq Task" {
        w555 = refnum<class "NI Force Task.lvclass"> refnum  # Force Task
        n298 = Unbundle By Name(w537) -> ("Monitor Select"=w536:refnum<vi>)
        n299 = property class="LVClassControl (strict)"(reference=w536) -> ("Value"=w535:refnum<class "Ref Display.lvclass">)  [unwired: 1 in, 2 out]
        n300 = call <vilib>:"Application Directory.vi"() -> ("Application Directory"=w575:path)
        n301 = Build Path(base path=w575, name or relative path=path "temp_ni.tdms") -> (appended path=w573:path)
        n302 = call-poly <vilib>:"Panel Type Selector.vi"("Window Position"=w535, "Default Title"="Task Window") -> ("Window out"=w562:refnum<class "Window.lvclass">)  [unwired: 8 in, 1 out]
        n303 = TDMS Open(10:T21."create or replace" ("operation (0:open)"), 11:w573) -> (3:w564:refnum<k34>)  [unwired: 5 in, 1 out]
        n304 = call <vilib>:"Launch Nested Panel.vi"("Panel"=w562, "Nested Panel Actor"=w555, "Panel Actor in"=w537) -> ("Nested Actor's Enqueuer"=w560:refnum<class "Message Enqueuer.lvclass">, "Panel Actor out"=w561:refnum<class "GUI.lvclass">)  [unwired: 5 in, 2 out]
        n305 = in-place {
          in-place-border: [w832] -> w566
          in-place-border: w564 -> [w831]
          in-place-border: [w831] -> w559
          in-place-border: [w830] -> w568
          in-place-border: [w825] -> w549
          in-place-border: [w822] -> w567
          in-place-border: [w820] -> _
          in-place-border: [w819] -> w565
          in-place-border: [w816] -> w563
          in-place-border: w560 -> [w815]
          in-place-border: [w815] -> w554
          in-place-border: [w814] -> w551
          in-place-border: [w813] -> w550
          in-place-border: [w812] -> w548
          in-place-border: [w809] -> w543
          in-place-border: [w808] -> w542
          in-place-border: [w807] -> w541
          in-place-border: [w806] -> w540
          in-place-border: [w805] -> w539
          in-place-border: [w804] -> w538
          in-place-border: [w799] -> w534
          in-place-border: [w798] -> w533
          in-place-border: [w797] -> w532
          n306 = in-place-cluster #13(w561) -> ("Task Selection"=w829:refnum<vi>, "Task Info Cluster"=w827:refnum<vi>, "DAQ Physical Channels"=w823:refnum<vi>, "Logger"=w819:refnum<class "Message Enqueuer.lvclass">, "Final File Path"=w818:refnum<vi>, "NI Data Subpanel"=w814:refnum<vi>, "Auto Clust"=w811:refnum<vi>, "Lissajou Subpanel"=w804:refnum<vi>, "Force Calibration Cluster"=w803:refnum<vi>, "Pot Calibration Cluster"=w802:refnum<vi>, "Trial Num Update"=w797:refnum<user-event>)  [unwired: 2 out]
          n307 = property class="Clust (strict)"(reference=w829) -> (reference out=w828:refnum<vi>, "Value"=w813:T3)  [unwired: 1 in, 1 out]
          n308 = property class="Clust (strict)"(reference=w811) -> (reference out=w810:refnum<vi>, "Value"=w806:T11)  [unwired: 1 in, 1 out]
          n309 = property class="Path"(reference=w818) -> (reference out=w817:refnum<vi>, "Value"=w816:path)  [unwired: 1 in, 1 out]
          n310 = Unbundle By Name(w813) -> ("Collect EMG?"=w798:bool, "EMG Rate"=w821:u16, "Acceleration Rate"=w820:u16, "Input Select Type"=w812:enum32{"Force Input", "Movement Input"})
          n311 = Unbundle By Name(w806) -> ("Automate?"=w809:bool, "Num Parabs"=w808:u16, "Patterns Array"=w807:u8[][], "Phase Array"=w805:i32[][])
          n312 = property class="Clust (strict)"(reference=w827) -> (reference out=w826:refnum<vi>, "Value"=w825:T4)  [unwired: 1 in, 1 out]
          n313 = property class="Clust (strict)"(reference=w823) -> (reference out=w824:refnum<vi>, "Value"=w822:T9)  [unwired: 1 in, 1 out]
          n314 = property class="Clust (strict)"(reference=w803) -> (reference out=w800:refnum<vi>, "Value"=w830:cluster{"Left":dbl, "Right":dbl})  [unwired: 1 in, 1 out]
          n315 = property class="Clust (strict)"(reference=w802) -> (reference out=w801:refnum<vi>, "Value"=w799:cluster{"Left 2":dbl, "Right 2":dbl})  [unwired: 1 in, 1 out]
          n316 = Bundle("Collect EMG?"=w798, "EMG Rate"=w821) -> (w832:cluster{"Collect EMG?":bool, "EMG Rate":u16})  [unwired: 1 in]
          n317 = in-place-cluster #13("Force TDMS File"=w831, "NI Force Task"=w815, "Task Selection"=w828, "Task Info Cluster"=w826, "DAQ Physical Channels"=w824, "Logger"=w819, "Final File Path"=w817, "NI Data Subpanel"=w814, "Auto Clust"=w810, "Lissajou Subpanel"=w804, "Force Calibration Cluster"=w800, "Pot Calibration Cluster"=w801, "Trial Num Update"=w797) -> ()  [unwired: 1 out]
        }
        n318 = call "Send Launch Viewer.vi"("EMG?"=w533, "Subpanel ref lissajous"=w538, "Collection Type"=w548, "Subpanel ref task"=w551, "Message Enqueuer in"=w554) -> ("error out"=w552:errorcluster, "Message Enqueuer out"=w553:refnum<class "Message Enqueuer.lvclass">)  [unwired: 5 in]
        n319 = case shown="\"Force Input\", Default" w548 {
          selector: w548 -> [w775 w787]
          tunnel: [w784 w796] -> w576
          tunnel: [w778 w795] -> w571
          tunnel: w568 -> [w780 _]
          tunnel: w567 -> [w782 w794]
          tunnel: w566 -> [w783 w793]
          tunnel: w559 -> [w781 w792]
          tunnel: w553 -> [w785 w791]
          tunnel: w552 -> [w779 w790]
          tunnel: w549 -> [w777 w789]
          tunnel: FALSE ("Scanning?") -> [w776 w788]
          tunnel: [w775 w787] -> w546
          tunnel: w534 -> [_ w786]
          frame "Force Input", Default {
            n320 = call "Send Initialize Force Task.vi"("Task Info In"=w777, "Scanning?"=w776, "EMG info"=w783, "DAQ  Channels In"=w782, "error in (no error)"=w779, "TDMS File"=w781, "Force Calibration Cluster"=w780, "Message Enqueuer in"=w785) -> ("error out"=w778:errorcluster, "Message Enqueuer out"=w784:refnum<class "Message Enqueuer.lvclass">)  [unwired: 2 in]
          }
          frame "Movement Input" {
            n321 = call "Send Initialize Movement Task.vi"("Scanning?"=w788, "Task Info In"=w789, "EMG info"=w793, "DAQ  Channels In"=w794, "error in (no error)"=w790, "TDMS File"=w792, "Pot Calibration Cluster"=w786, "Message Enqueuer in"=w791) -> ("error out"=w795:errorcluster, "Message Enqueuer out"=w796:refnum<class "Message Enqueuer.lvclass">)  [unwired: 2 in]
          }
        }
        n322 = case shown="True" w543 {
          tunnel: w576 -> [w592 w693]
          tunnel: w571 -> [w577 w692]
          tunnel: [w591 w691] -> w569
          tunnel: w549 -> [w586 w681]
          tunnel: w542 -> [w588 _]
          tunnel: w541 -> [w587 _]
          tunnel: w539 -> [w585 _]
          tunnel: w532 -> [w581 w680]
          frame True {
            n323 = Unbundle By Name(w586) -> ("Trial Duration (s)"=w589:u8)
            n324 = Multiply(x=1000, y=w589) -> (x*y=w583:i32)
            n325 = Add(x=w583, y=1100) -> (x+y=w582:i32)
            n326 = property class="VI"(error in=w577, "Front Panel.IsFrontmost"=TRUE ("Front Panel Window:Is Frontmost")) -> (error out=w578:errorcluster)  [unwired: 1 in, 1 out]
            n327 = while {
              tunnel: w578 -> [w593]
              tunnel: [w593] -> w580
              stop <- w596 stop-if-true
              n328 = One Button Dialog(message="Ready for acquisition", button name ("OK")="Begin") -> (true=w596:bool)
            }
            n329 = for {
              N: w588 -> [w622]
              tunnel: w592 -> [w615]
              tunnel: [w630] -> w591
              tunnel: w582 -> [w628]
              tunnel: w587 -> [w620] mode=indexing
              tunnel: w586 -> [w621]
              tunnel: w585 -> [w609] mode=indexing
              tunnel: w581 -> [w604]
              tunnel: w580 -> [w597]
              i -> [w638]
              stop <- w626 stop-if-true
              n330 = Index Array(array=w620, index #1=0 ("index"), index #2=1 ("index")) -> (element #1=w617:u8, element #2=w616:u8)
              n331 = Index Array(array=w609, index #1=0 ("index"), index #2=1 ("index")) -> (element #1=w608:i32, element #2=w607:i32)
              n332 = Bundle By Name(cluster=w621, "L Pattern"=w617, "R Pattern"=w616, "L Phase"=w608, "R Phase"=w607) -> (w614:T4)
              n333 = call "Send Update Template Graph.vi"("Set Task Info?"=FALSE, "error in (no error)"=w597, "Update Axes Scale"=TRUE, "Task Info In"=w614, "Message Enqueuer in"=w615) -> ("error out"=w612:errorcluster, "Message Enqueuer out"=w613:refnum<class "Message Enqueuer.lvclass">)  [unwired: 5 in]
              n334 = Increment(x=w638) -> (x+1=w603:i32)
              n335 = Generate User Event(user event=w604, event data cluster=w603) -> ()  [unwired: 2 in, 2 out]
              n336 = flat-sequence {
                tunnel: w613 -> [w646]
                tunnel: w603 -> [w640]
                tunnel: [w648] -> w636
                tunnel: [w643] -> w634
                tunnel: w612 -> [w642]
                tunnel: [w641] -> w629
                tunnel: w628 -> [w641]
                tunnel: [w640] -> w623
                tunnel: [w654] -> w637
                tunnel: w636 -> [w654]
                tunnel: [w653] -> w635
                tunnel: w634 -> [w653]
                tunnel: w629 -> [w652]
                tunnel: [w650] -> w624
                tunnel: w623 -> [w650]
                tunnel: [w649] -> w599
                tunnel: w637 -> [w666]
                tunnel: w635 -> [w665]
                tunnel: [w664] -> w633
                tunnel: [w663] -> w631
                tunnel: [w662] -> w625
                tunnel: w624 -> [w662]
                tunnel: [w660] -> w600
                tunnel: w599 -> [w660]
                tunnel: w633 -> [w673]
                tunnel: [w673] -> w632
                tunnel: [w672] -> w630
                tunnel: w631 -> [w672]
                tunnel: w625 -> [w670]
                tunnel: w622 -> [w671]
                tunnel: w600 -> [w667]
                tunnel: [w667] -> w598
                frame #0 {
                  n337 = call "Send Stop Trial.vi"("error in (no error)"=w642, "DAQ Task"=TRUE, "Stop Acquiring"=FALSE, "Message Enqueuer in"=w646) -> ("error out"=w644:errorcluster, "Message Enqueuer out"=w645:refnum<class "Message Enqueuer.lvclass">)  [unwired: 6 in]
                  n338 = call "Send Start Trial.vi"("error in (no error)"=w644, "Trial Number"=w640, "Message Enqueuer in"=w645) -> ("error out"=w643:errorcluster, "Message Enqueuer out"=w648:refnum<class "Message Enqueuer.lvclass">)  [unwired: 7 in]
                }
                frame #1 {
                  n339 = while {
                    tunnel: w652 -> [w659]
                    shift-right: [w657] -> _
                    shift-left: TRUE ("reset") -> [w658]
                    tunnel: [w655] -> w649
                    stop <- w656 stop-if-true
                    n340 = call <userlib>:"Periodic Trigger__ogtk.vi"("time (ms)"=w659, "reset"=w658) -> ("Triggered"=w657:bool)  [unwired: 11 in, 2 out]
                    n341 = local read "Abort Signal"() -> (w655:bool)
                    n342 = Or(x=w657, y=w655) -> (x .or. y?=w656:bool)
                  }
                }
                frame #2 {
                  w661 = TRUE ("Stop Acquiring")
                  n343 = call "Send Stop Trial.vi"("error in (no error)"=w665, "DAQ Task"=w661, "Stop Acquiring"=w661, "Message Enqueuer in"=w666) -> ("error out"=w664:errorcluster, "Message Enqueuer out"=w663:refnum<class "Message Enqueuer.lvclass">)  [unwired: 6 in]
                }
                frame #3 {
                  n344 = Equal?(x=w671, y=w670) -> (x = y?=w669:bool)
                  n345 = Or(x=w669, y=w667) -> (x .or. y?=w668:bool)
                  n346 = case shown="False" w668 {
                    frame False {
                      n347 = while {
                        stop <- w677 stop-if-true
                        n348 = local read "Abort Signal"() -> (w678:bool)
                        n349 = One Button Dialog(message="Press \"Next\" button or Enter key to continue", button name ("OK")="Next") -> (true=w676:bool)
                        n350 = Or(x=w676, y=w678) -> (x .or. y?=w677:bool)
                      }
                    }
                    frame True {
                      n351 = Wait (ms)(milliseconds to wait=u32 2000) -> ()  [unwired: 1 out]
                    }
                  }
                }
              }
              n352 = Select(t=w598, s=w598, f=FALSE) -> (s? t:f=w601:bool)
              n353 = Unbundle By Name(w632) -> ("status"=w627:bool)
              n354 = Or(x=w627, y=w601) -> (x .or. y?=w626:bool)
            }
          }
          frame False {
            n355 = Unbundle By Name(w681) -> ("Number of Trials"=w690:u8, "Trial Duration (s)"=w688:u8, "Time Between Trials (s)"=w687:u8)
            n356 = Multiply(x=1000, y=w688) -> (x*y=w684:i32)
            n357 = Add(x=1100 ("y"), y=w684) -> (x+y=w682:i32)
            n358 = Multiply(x=1000, y=w687) -> (x*y=w685:i32)
            n359 = for {
              N: w690 -> [w707]
              tunnel: w693 -> [w705]
              tunnel: w692 -> [w706]
              tunnel: [w719] -> w691
              tunnel: w682 -> [w717]
              tunnel: w685 -> [w715]
              tunnel: w681 -> [w701]
              tunnel: w680 -> [w700]
              i -> [w727]
              stop <- w711 stop-if-true
              n360 = Increment(x=w727) -> (x+1=w699:i32)
              n361 = call "Send Update Template Graph.vi"("error in (no error)"=w706, "Update Axes Scale"=TRUE, "Task Info In"=w701, "Message Enqueuer in"=w705) -> ("error out"=w702:errorcluster, "Message Enqueuer out"=w703:refnum<class "Message Enqueuer.lvclass">)  [unwired: 6 in]
              n362 = Generate User Event(user event=w700, event data cluster=w699) -> ()  [unwired: 2 in, 2 out]
              n363 = flat-sequence {
                tunnel: [w730] -> _
                tunnel: w699 -> [w731]
                tunnel: [w738] -> w725
                tunnel: [w734] -> w723
                tunnel: [w733] -> w718
                tunnel: w717 -> [w733]
                tunnel: [w732] -> w716
                tunnel: w715 -> [w732]
                tunnel: [w731] -> w708
                tunnel: w703 -> [w730]
                tunnel: w702 -> [w729]
                tunnel: [w745] -> w726
                tunnel: w725 -> [w745]
                tunnel: [w744] -> w724
                tunnel: w723 -> [w744]
                tunnel: w718 -> [w742]
                tunnel: w716 -> [w743]
                tunnel: [w743] -> w713
                tunnel: [w740] -> w709
                tunnel: w708 -> [w740]
                tunnel: [w739] -> w698
                tunnel: w726 -> [w758]
                tunnel: w724 -> [w757]
                tunnel: [w756] -> w722
                tunnel: [w755] -> w720
                tunnel: [w754] -> w714
                tunnel: w713 -> [w754]
                tunnel: [w753] -> w710
                tunnel: w709 -> [w753]
                tunnel: w698 -> [w751]
                tunnel: [w751] -> w697
                tunnel: w722 -> [w766]
                tunnel: [w766] -> w721
                tunnel: [w765] -> w719
                tunnel: w720 -> [w765]
                tunnel: w714 -> [w762]
                tunnel: w710 -> [w763]
                tunnel: w707 -> [w764]
                tunnel: [w759] -> w696
                tunnel: w697 -> [w759]
                frame #0 {
                  n364 = call "Send Stop Trial.vi"("error in (no error)"=w729, "DAQ Task"=TRUE, "Stop Acquiring"=FALSE, "Message Enqueuer in"=w730) -> ("error out"=w735:errorcluster, "Message Enqueuer out"=w736:refnum<class "Message Enqueuer.lvclass">)  [unwired: 6 in]
                  n365 = call "Send Start Trial.vi"("error in (no error)"=w735, "Trial Number"=w731, "Message Enqueuer in"=w736) -> ("error out"=w734:errorcluster, "Message Enqueuer out"=w738:refnum<class "Message Enqueuer.lvclass">)  [unwired: 7 in]
                }
                frame #1 {
                  n366 = while {
                    tunnel: w742 -> [w750]
                    shift-right: [w748] -> _
                    shift-left: TRUE ("reset") -> [w749]
                    tunnel: [w746] -> w739
                    stop <- w747 stop-if-true
                    n367 = local read "Abort Signal"() -> (w746:bool)
                    n368 = call <userlib>:"Periodic Trigger__ogtk.vi"("time (ms)"=w750, "reset"=w749) -> ("Triggered"=w748:bool)  [unwired: 11 in, 2 out]
                    n369 = Or(x=w748, y=w746) -> (x .or. y?=w747:bool)
                  }
                }
                frame #2 {
                  w752 = TRUE ("Stop Acquiring")
                  n370 = call "Send Stop Trial.vi"("error in (no error)"=w757, "DAQ Task"=w752, "Stop Acquiring"=w752, "Message Enqueuer in"=w758) -> ("error out"=w756:errorcluster, "Message Enqueuer out"=w755:refnum<class "Message Enqueuer.lvclass">)  [unwired: 6 in]
                }
                frame #3 {
                  n371 = Equal?(x=w764, y=w763) -> (x = y?=w761:bool)
                  n372 = Or(x=w761, y=w759) -> (x .or. y?=w760:bool)
                  n373 = case shown="False" w760 {
                    tunnel: w762 -> [w768 _]
                    frame False {
                      n374 = while {
                        tunnel: w768 -> [w773]
                        shift-right: [w771] -> _
                        shift-left: TRUE ("reset") -> [w772]
                        stop <- w769 stop-if-true
                        n375 = local read "Abort Signal"() -> (w770:bool)
                        n376 = call <userlib>:"Periodic Trigger__ogtk.vi"("time (ms)"=w773, "reset"=w772) -> ("Triggered"=w771:bool)  [unwired: 11 in, 2 out]
                        n377 = Or(x=w771, y=w770) -> (x .or. y?=w769:bool)
                      }
                    }
                    frame True {
                      n378 = Wait (ms)(milliseconds to wait=u32 2000) -> ()  [unwired: 1 out]
                    }
                  }
                }
              }
              n379 = Unbundle By Name(w721) -> ("status"=w712:bool)
              n380 = Select(t=w696, s=w696, f=FALSE) -> (s? t:f=w694:bool)
              n381 = Or(x=w712, y=w694) -> (x .or. y?=w711:bool)
            }
          }
        }
        n382 = case shown="\"Force Input\", Default" w546 {
          tunnel: [FALSE TRUE] -> w545
          frame "Force Input", Default {
          }
          frame "Movement Input" {
          }
        }
        n383 = call "Send External Shutdown.vi"("Message Enqueuer in"=w569) -> ("error out"=w544:errorcluster)  [unwired: 9 in, 1 out]
        n384 = call "Send TDMS Cleanup.vi"("Auto Clust"=w540, "Movement?"=w545, "Task info"=w549, "Force TDMS File"=w559, "Task Selection"=w550, "error in (no error)"=w544, "TDMS File"=w563, "Message Enqueuer in"=w565) -> ("error out"=w556:errorcluster)  [unwired: 2 in, 1 out]
        n385 = Enqueue Element(queue=w557, element=Task_Active_Enum_df."Idle", error in (no error)=w556) -> ()  [unwired: 1 in, 3 out]
      }
      frame "Start Freq Task and Accel" {
        w885 = refnum<class "Accelerometer.lvclass"> refnum  # Accelerometer
        w888 = refnum<class "NI Force Task.lvclass"> refnum  # Force Task
        n386 = Unbundle By Name(w840) -> ("Monitor Select"=w839:refnum<vi>)
        n387 = property class="LVClassControl (strict)"(reference=w839) -> ("Value"=w838:refnum<class "Ref Display.lvclass">)  [unwired: 1 in, 2 out]
        n388 = control-ref of="Accelerometer Data"() -> (w889:refnum<vi>)
        n389 = call-poly <vilib>:"Panel Type Selector.vi"("Sub Panel"=w889) -> ("Subpanel Out"=w886:refnum<class "Subpanel.lvclass">)  [unwired: 9 in, 1 out]
        n390 = call <vilib>:"Application Directory.vi"() -> ("Application Directory"=w898:path)
        n391 = call-poly <vilib>:"Panel Type Selector.vi"("Window Position"=w838, "Default Title"="Task Window") -> ("Window out"=w887:refnum<class "Window.lvclass">)  [unwired: 8 in, 1 out]
        n392 = call <vilib>:"Application Directory.vi"() -> ("Application Directory"=w875:path)
        n393 = Build Path(base path=w898, name or relative path=path "temp_ni.tdms") -> (appended path=w897:path)
        n394 = Build Path(base path=w875, name or relative path=path "temp_accel.tdms") -> (appended path=w873:path)
        n395 = Bundle("Force Task"=w888, "Window out"=w887) -> (w883:T23)  [unwired: 1 in]
        n396 = Bundle("Accelerometer"=w885, "Subpanel Out"=w886) -> (w884:T24)  [unwired: 1 in]
        n397 = Build Array(w883, w884) -> (w882:T25)
        n398 = TDMS Open(10:T21."create or replace" ("operation (0:open)"), 11:w897) -> (3:w868:refnum<k34>)  [unwired: 5 in, 1 out]
        n399 = TDMS Open(10:T21."create or replace" ("operation (0:open)"), 11:w873) -> (3:w869:refnum<k34>)  [unwired: 5 in, 1 out]
        n400 = call <vilib>:"Launch Nested Panels.vi"("Nested Panel Actors"=w882, "Panel Actor in"=w840) -> ("Nested Actor's Enqueuers"=w881:refnum<class "Message Enqueuer.lvclass">[], "Panel Actor out"=w890:refnum<class "GUI.lvclass">)  [unwired: 6 in, 2 out]
        n401 = in-place {
          in-place-border: [w959] -> w891
          in-place-border: w868 -> [w958]
          in-place-border: [w958] -> w866
          in-place-border: [w957] -> w893
          in-place-border: [w952] -> w852
          in-place-border: [w949] -> w892
          in-place-border: [w945] -> w877
          in-place-border: [w947] -> w876
          in-place-border: w869 -> [w946]
          in-place-border: [w946] -> w865
          in-place-border: [w944] -> w858
          in-place-border: [w943] -> w870
          in-place-border: [w940] -> w864
          in-place-border: [w939] -> w854
          in-place-border: [w938] -> w851
          in-place-border: [w937] -> w850
          in-place-border: [w937] -> w849
          in-place-border: [w934] -> w846
          in-place-border: [w933] -> w845
          in-place-border: [w932] -> w844
          in-place-border: [w931] -> w843
          in-place-border: [w930] -> w842
          in-place-border: [w929] -> w841
          in-place-border: [w924] -> w837
          in-place-border: [w923] -> w836
          in-place-border: [w922] -> w835
          n402 = in-place-cluster #14(w890) -> ("Task Selection"=w956:refnum<vi>, "Task Info Cluster"=w954:refnum<vi>, "DAQ Physical Channels"=w950:refnum<vi>, "Logger"=w943:refnum<class "Message Enqueuer.lvclass">, "Final File Path"=w942:refnum<vi>, "NI Data Subpanel"=w939:refnum<vi>, "Auto Clust"=w936:refnum<vi>, "Lissajou Subpanel"=w929:refnum<vi>, "Force Calibration Cluster"=w928:refnum<vi>, "Pot Calibration Cluster"=w927:refnum<vi>, "Trial Num Update"=w922:refnum<user-event>)  [unwired: 4 out]
          n403 = in-place-array #15(w881, 0, 1) -> (w944:refnum<class "Message Enqueuer.lvclass">, w945:refnum<class "Message Enqueuer.lvclass">)
          n404 = property class="Clust (strict)"(reference=w956) -> (reference out=w955:refnum<vi>, "Value"=w938:T3)  [unwired: 1 in, 1 out]
          n405 = property class="Path"(reference=w942) -> (reference out=w941:refnum<vi>, "Value"=w940:path)  [unwired: 1 in, 1 out]
          n406 = property class="Clust (strict)"(reference=w936) -> (reference out=w935:refnum<vi>, "Value"=w931:T11)  [unwired: 1 in, 1 out]
          n407 = Unbundle By Name(w938) -> ("Collect EMG?"=w923:bool, "EMG Rate"=w948:u16, "Acceleration Rate"=w947:u16, "Input Select Type"=w937:enum32{"Force Input", "Movement Input"})
          n408 = property class="Clust (strict)"(reference=w928) -> (reference out=w926:refnum<vi>, "Value"=w957:cluster{"Left":dbl, "Right":dbl})  [unwired: 1 in, 1 out]
          n409 = property class="Clust (strict)"(reference=w927) -> (reference out=w925:refnum<vi>, "Value"=w924:cluster{"Left 2":dbl, "Right 2":dbl})  [unwired: 1 in, 1 out]
          n410 = Unbundle By Name(w931) -> ("Automate?"=w934:bool, "Num Parabs"=w933:u16, "Patterns Array"=w932:u8[][], "Phase Array"=w930:i32[][])
          n411 = property class="Clust (strict)"(reference=w954) -> (reference out=w953:refnum<vi>, "Value"=w952:T4)  [unwired: 1 in, 1 out]
          n412 = property class="Clust (strict)"(reference=w950) -> (reference out=w951:refnum<vi>, "Value"=w949:T9)  [unwired: 1 in, 1 out]
          n413 = Bundle("Collect EMG?"=w923, "EMG Rate"=w948) -> (w959:cluster{"Collect EMG?":bool, "EMG Rate":u16})  [unwired: 1 in]
          n414 = in-place-cluster #14("Force TDMS File"=w958, "NI Force Task"=w944, "Task Selection"=w955, "Task Info Cluster"=w953, "DAQ Physical Channels"=w951, "Accelerometer"=w945, "Accel TDMS File"=w946, "Logger"=w943, "Final File Path"=w941, "NI Data Subpanel"=w939, "Auto Clust"=w935, "Lissajou Subpanel"=w929, "Force Calibration Cluster"=w926, "Pot Calibration Cluster"=w925, "Trial Num Update"=w922) -> ()  [unwired: 1 out]
          n415 = in-place-array #15(w944, w945) -> ()  [unwired: 3 out]
        }
        n416 = call "Send Initialize Accel Task.vi"("Accel TDMS File"=w865, "Accel Rate"=w876, "Message Enqueuer in"=w877) -> ("error out"=w855:errorcluster, "Message Enqueuer out"=w878:refnum<class "Message Enqueuer.lvclass">)  [unwired: 7 in]
        n417 = call "Send Launch Viewer.vi"("EMG?"=w836, "Subpanel ref lissajous"=w841, "Collection Type"=w850, "Subpanel ref task"=w854, "Message Enqueuer in"=w858) -> ("error out"=w857:errorcluster, "Message Enqueuer out"=w859:refnum<class "Message Enqueuer.lvclass">)  [unwired: 5 in]
        n418 = case shown="\"Movement Input\"" w849 {
          selector: w849 -> [w900 w912]
          tunnel: [w904 w921] -> w899
          tunnel: w893 -> [w909 _]
          tunnel: w892 -> [w906 w920]
          tunnel: w891 -> [w903 w919]
          tunnel: w866 -> [w908 w918]
          tunnel: w859 -> [w910 w917]
          tunnel: w857 -> [w907 w916]
          tunnel: [w905 w915] -> w856
          tunnel: w852 -> [w902 w914]
          tunnel: FALSE -> [w901 w913]
          tunnel: [w900 w912] -> w847
          tunnel: w837 -> [_ w911]
          frame "Force Input", Default {
            n419 = call "Send Initialize Force Task.vi"("Task Info In"=w902, "Scanning?"=w901, "EMG info"=w903, "DAQ  Channels In"=w906, "error in (no error)"=w907, "TDMS File"=w908, "Force Calibration Cluster"=w909, "Message Enqueuer in"=w910) -> ("error out"=w905:errorcluster, "Message Enqueuer out"=w904:refnum<class "Message Enqueuer.lvclass">)  [unwired: 2 in]
          }
          frame "Movement Input" {
            n420 = call "Send Initialize Movement Task.vi"("Scanning?"=w913, "Task Info In"=w914, "EMG info"=w919, "DAQ  Channels In"=w920, "error in (no error)"=w916, "TDMS File"=w918, "Pot Calibration Cluster"=w911, "Message Enqueuer in"=w917) -> ("error out"=w915:errorcluster, "Message Enqueuer out"=w921:refnum<class "Message Enqueuer.lvclass">)  [unwired: 2 in]
          }
        }
        n421 = case shown="True" w846 {
          tunnel: w899 -> [w979 w1106]
          tunnel: [w978 w1105] -> w894
          tunnel: w878 -> [w977 w1104]
          tunnel: [w976 w1103] -> w871
          tunnel: w856 -> [w964 w1101]
          tunnel: w855 -> [w961 w1100]
          tunnel: w852 -> [w971 w1091]
          tunnel: w845 -> [w973 _]
          tunnel: w844 -> [w972 _]
          tunnel: w842 -> [w970 _]
          tunnel: w835 -> [w966 w1090]
          frame True {
            n422 = property class="VI"(error in=w964, "Front Panel.IsFrontmost"=TRUE ("Front Panel Window:Is Frontmost")) -> (error out=w962:errorcluster)  [unwired: 1 in, 1 out]
            n423 = while {
              tunnel: w962 -> [w981]
              tunnel: [w981] -> w963
              tunnel: [w980] -> w960
              tunnel: w961 -> [w980]
              stop <- w984 stop-if-true
              n424 = One Button Dialog(message="Ready for acquisition", button name ("OK")="Begin") -> (true=w984:bool)
            }
            n425 = Unbundle By Name(w971) -> ("Trial Duration (s)"=w974:u8)
            n426 = Multiply(x=1000, y=w974) -> (x*y=w968:i32)
            n427 = Add(x=w968, y=1100) -> (x+y=w967:i32)
            n428 = for {
              N: w973 -> [w1014]
              tunnel: w979 -> [w1001]
              tunnel: [w1025] -> w978
              tunnel: w967 -> [w1023]
              tunnel: w977 -> [w1005]
              tunnel: [w1016] -> w976
              tunnel: w963 -> [w1000]
              tunnel: w960 -> [w1015]
              tunnel: w972 -> [w1004] mode=indexing
              tunnel: w971 -> [w997]
              tunnel: w970 -> [w995] mode=indexing
              tunnel: w966 -> [w991]
              i -> [w1032]
              stop <- w1006 stop-if-true
              (unwired) 1 ("index")
              (unwired) 0 ("index")
              (unwired) 1 ("index")
              (unwired) 0 ("index")
              n429 = Index Array(array=w1004) -> (element #1=w1003:u8, element #2=w1002:u8)  [unwired: 2 in]
              n430 = Index Array(array=w995) -> (element #1=w994:i32, element #2=w993:i32)  [unwired: 2 in]
              n431 = Bundle By Name(cluster=w997, "L Pattern"=w1003, "R Pattern"=w1002, "L Phase"=w994, "R Phase"=w993) -> (w996:T4)
              n432 = call "Send Update Template Graph.vi"("error in (no error)"=w1000, "Update Axes Scale"=TRUE, "Task Info In"=w996, "Message Enqueuer in"=w1001) -> ("error out"=w998:errorcluster, "Message Enqueuer out"=w999:refnum<class "Message Enqueuer.lvclass">)  [unwired: 6 in]
              n433 = Increment(x=w1032) -> (x+1=w990:i32)
              n434 = Generate User Event(user event=w991, event data cluster=w990) -> ()  [unwired: 2 in, 2 out]
              n435 = flat-sequence {
                tunnel: w990 -> [w1036]
                tunnel: [w1049] -> w1030
                tunnel: [w1045] -> w1028
                tunnel: [w1044] -> w1024
                tunnel: w1023 -> [w1044]
                tunnel: w1005 -> [w1043]
                tunnel: [w1039] -> w1021
                tunnel: [w1038] -> w1019
                tunnel: [w1034] -> _
                tunnel: w1015 -> [w1037]
                tunnel: [w1036] -> w1013
                tunnel: w999 -> [w1035]
                tunnel: w998 -> [w1034]
                tunnel: [w1057] -> w1031
                tunnel: w1030 -> [w1057]
                tunnel: [w1056] -> w1029
                tunnel: w1028 -> [w1056]
                tunnel: w1024 -> [w1052]
                tunnel: [w1055] -> w1022
                tunnel: w1021 -> [w1055]
                tunnel: [w1054] -> w1020
                tunnel: w1019 -> [w1054]
                tunnel: w1013 -> [w1051]
                tunnel: [w1051] -> w1012
                tunnel: [w1050] -> w986
                tunnel: w1031 -> [w1074]
                tunnel: w1029 -> [w1073]
                tunnel: [w1072] -> w1027
                tunnel: [w1071] -> w1026
                tunnel: w1022 -> [w1069]
                tunnel: w1020 -> [w1068]
                tunnel: [w1067] -> w1018
                tunnel: [w1066] -> w1017
                tunnel: w1012 -> [w1065]
                tunnel: [w1065] -> w1011
                tunnel: [w1063] -> w987
                tunnel: w986 -> [w1063]
                tunnel: w1027 -> [w1083]
                tunnel: [w1083] -> w1010
                tunnel: [w1082] -> w1025
                tunnel: w1026 -> [w1082]
                tunnel: [w1081] -> w1009
                tunnel: w1018 -> [w1081]
                tunnel: w1017 -> [w1080]
                tunnel: [w1080] -> w1016
                tunnel: w1014 -> [w1079]
                tunnel: w1011 -> [w1078]
                tunnel: [w1075] -> w985
                tunnel: w987 -> [w1075]
                frame #0 {
                  n436 = call "Send Stop Trial.vi"("error in (no error)"=w1037, "Stop Acquiring"=FALSE, "Message Enqueuer in"=w1043) -> ("error out"=w1040:errorcluster, "Message Enqueuer out"=w1041:refnum<class "Message Enqueuer.lvclass">)  [unwired: 7 in]
                  n437 = call "Send Stop Trial.vi"("error in (no error)"=w1034, "DAQ Task"=TRUE, "Stop Acquiring"=FALSE, "Message Enqueuer in"=w1035) -> ("error out"=w1046:errorcluster, "Message Enqueuer out"=w1047:refnum<class "Message Enqueuer.lvclass">)  [unwired: 6 in]
                  n438 = call "Send Start Trial.vi"("error in (no error)"=w1040, "Trial Number"=w1036, "Message Enqueuer in"=w1041) -> ("error out"=w1038:errorcluster, "Message Enqueuer out"=w1039:refnum<class "Message Enqueuer.lvclass">)  [unwired: 7 in]
                  n439 = call "Send Start Trial.vi"("error in (no error)"=w1046, "Trial Number"=w1036, "Message Enqueuer in"=w1047) -> ("error out"=w1045:errorcluster, "Message Enqueuer out"=w1049:refnum<class "Message Enqueuer.lvclass">)  [unwired: 7 in]
                }
                frame #1 {
                  n440 = while {
                    shift-right: [w1061] -> _
                    shift-left: TRUE -> [w1060]
                    tunnel: w1052 -> [w1059]
                    tunnel: [w1058] -> w1050
                    stop <- w1062 stop-if-true
                    n441 = local read "Abort Signal"() -> (w1058:bool)
                    n442 = call <userlib>:"Periodic Trigger__ogtk.vi"("time (ms)"=w1059, "reset"=w1060) -> ("Triggered"=w1061:bool)  [unwired: 11 in, 2 out]
                    n443 = Or(x=w1061, y=w1058) -> (x .or. y?=w1062:bool)
                  }
                }
                frame #2 {
                  w1064 = TRUE ("Stop Acquiring")
                  n444 = call "Send Stop Trial.vi"("error in (no error)"=w1068, "Stop Acquiring"=TRUE, "Message Enqueuer in"=w1069) -> ("error out"=w1067:errorcluster, "Message Enqueuer out"=w1066:refnum<class "Message Enqueuer.lvclass">)  [unwired: 7 in]
                  n445 = call "Send Stop Trial.vi"("error in (no error)"=w1073, "DAQ Task"=w1064, "Stop Acquiring"=w1064, "Message Enqueuer in"=w1074) -> ("error out"=w1072:errorcluster, "Message Enqueuer out"=w1071:refnum<class "Message Enqueuer.lvclass">)  [unwired: 6 in]
                }
                frame #3 {
                  n446 = Equal?(x=w1079, y=w1078) -> (x = y?=w1077:bool)
                  n447 = Or(x=w1077, y=w1075) -> (x .or. y?=w1076:bool)
                  n448 = case shown="False" w1076 {
                    frame False {
                      n449 = while {
                        stop <- w1088 stop-if-true
                        n450 = local read "Abort Signal"() -> (w1087:bool)
                        n451 = One Button Dialog(message="Press \"Next\" button or Enter key to continue", button name ("OK")="Next") -> (true=w1084:bool)
                        n452 = Or(x=w1084, y=w1087) -> (x .or. y?=w1088:bool)
                      }
                    }
                    frame True {
                      n453 = Wait (ms)(milliseconds to wait=u32 2000) -> ()  [unwired: 1 out]
                    }
                  }
                }
              }
              n454 = Merge Errors(w1010, w1009) -> (w1008:errorcluster)
              n455 = Unbundle By Name(w1008) -> ("status"=w1007:bool)
              n456 = Select(t=w985, s=w985, f=FALSE) -> (s? t:f=w988:bool)
              n457 = Or(x=w1007, y=w988) -> (x .or. y?=w1006:bool)
            }
          }
          frame False {
            n458 = Unbundle By Name(w1091) -> ("Number of Trials"=w1102:u8, "Trial Duration (s)"=w1097:u8, "Time Between Trials (s)"=w1096:u8)
            n459 = Multiply(x=1000, y=w1096) -> (x*y=w1095:i32)
            n460 = Multiply(x=1000, y=w1097) -> (x*y=w1093:i32)
            n461 = Add(x=1100 ("y"), y=w1093) -> (x+y=w1092:i32)
            n462 = for {
              N: w1102 -> [w1128]
              tunnel: w1106 -> [w1118]
              tunnel: [w1144] -> w1105
              tunnel: w1092 -> [w1142]
              tunnel: w1095 -> [w1140]
              tunnel: w1104 -> [w1137]
              tunnel: [w1130] -> w1103
              tunnel: w1101 -> [w1119]
              tunnel: w1100 -> [w1129]
              tunnel: w1091 -> [w1114]
              tunnel: w1090 -> [w1113]
              i -> [w1151]
              stop <- w1120 stop-if-true
              n463 = Increment(x=w1151) -> (x+1=w1112:i32)
              n464 = call "Send Update Template Graph.vi"("error in (no error)"=w1119, "Update Axes Scale"=TRUE, "Task Info In"=w1114, "Message Enqueuer in"=w1118) -> ("error out"=w1115:errorcluster, "Message Enqueuer out"=w1116:refnum<class "Message Enqueuer.lvclass">)  [unwired: 6 in]
              n465 = Generate User Event(user event=w1113, event data cluster=w1112) -> ()  [unwired: 2 in, 2 out]
              n466 = flat-sequence {
                tunnel: w1116 -> [w1167]
                tunnel: w1112 -> [w1154]
                tunnel: [w1169] -> w1149
                tunnel: [w1164] -> w1147
                tunnel: [w1163] -> w1143
                tunnel: w1142 -> [w1163]
                tunnel: [w1162] -> w1141
                tunnel: w1140 -> [w1162]
                tunnel: w1137 -> [w1161]
                tunnel: [w1157] -> w1135
                tunnel: [w1156] -> w1133
                tunnel: w1129 -> [w1155]
                tunnel: [w1154] -> w1127
                tunnel: w1115 -> [w1153]
                tunnel: [w1178] -> w1150
                tunnel: w1149 -> [w1178]
                tunnel: [w1177] -> w1148
                tunnel: w1147 -> [w1177]
                tunnel: w1143 -> [w1172]
                tunnel: w1141 -> [w1176]
                tunnel: [w1176] -> w1138
                tunnel: [w1175] -> w1136
                tunnel: w1135 -> [w1175]
                tunnel: [w1174] -> w1134
                tunnel: w1133 -> [w1174]
                tunnel: w1127 -> [w1171]
                tunnel: [w1171] -> w1126
                tunnel: [w1170] -> w1109
                tunnel: w1150 -> [w1196]
                tunnel: w1148 -> [w1195]
                tunnel: [w1194] -> w1146
                tunnel: [w1193] -> w1145
                tunnel: [w1192] -> w1139
                tunnel: w1138 -> [w1192]
                tunnel: w1136 -> [w1190]
                tunnel: w1134 -> [w1189]
                tunnel: [w1188] -> w1132
                tunnel: [w1187] -> w1131
                tunnel: w1126 -> [w1186]
                tunnel: [w1186] -> w1125
                tunnel: w1109 -> [w1184]
                tunnel: [w1184] -> w1108
                tunnel: w1146 -> [w1206]
                tunnel: [w1206] -> w1124
                tunnel: [w1205] -> w1144
                tunnel: w1145 -> [w1205]
                tunnel: w1139 -> [w1200]
                tunnel: [w1204] -> w1123
                tunnel: w1132 -> [w1204]
                tunnel: w1131 -> [w1203]
                tunnel: [w1203] -> w1130
                tunnel: w1128 -> [w1202]
                tunnel: w1125 -> [w1201]
                tunnel: [w1197] -> w1107
                tunnel: w1108 -> [w1197]
                frame #0 {
                  n467 = call "Send Stop Trial.vi"("error in (no error)"=w1155, "Stop Acquiring"=FALSE, "Message Enqueuer in"=w1161) -> ("error out"=w1158:errorcluster, "Message Enqueuer out"=w1159:refnum<class "Message Enqueuer.lvclass">)  [unwired: 7 in]
                  n468 = call "Send Stop Trial.vi"("error in (no error)"=w1153, "DAQ Task"=TRUE, "Stop Acquiring"=FALSE, "Message Enqueuer in"=w1167) -> ("error out"=w1165:errorcluster, "Message Enqueuer out"=w1166:refnum<class "Message Enqueuer.lvclass">)  [unwired: 6 in]
                  n469 = call "Send Start Trial.vi"("error in (no error)"=w1158, "Trial Number"=w1154, "Message Enqueuer in"=w1159) -> ("error out"=w1156:errorcluster, "Message Enqueuer out"=w1157:refnum<class "Message Enqueuer.lvclass">)  [unwired: 7 in]
                  n470 = call "Send Start Trial.vi"("error in (no error)"=w1165, "Trial Number"=w1154, "Message Enqueuer in"=w1166) -> ("error out"=w1164:errorcluster, "Message Enqueuer out"=w1169:refnum<class "Message Enqueuer.lvclass">)  [unwired: 7 in]
                }
                frame #1 {
                  n471 = while {
                    shift-right: [w1182] -> _
                    shift-left: TRUE -> [w1181]
                    tunnel: w1172 -> [w1180]
                    tunnel: [w1179] -> w1170
                    stop <- w1183 stop-if-true
                    n472 = local read "Abort Signal"() -> (w1179:bool)
                    n473 = call <userlib>:"Periodic Trigger__ogtk.vi"("time (ms)"=w1180, "reset"=w1181) -> ("Triggered"=w1182:bool)  [unwired: 11 in, 2 out]
                    n474 = Or(x=w1182, y=w1179) -> (x .or. y?=w1183:bool)
                  }
                }
                frame #2 {
                  w1185 = TRUE ("Stop Acquiring")
                  n475 = call "Send Stop Trial.vi"("error in (no error)"=w1189, "Stop Acquiring"=TRUE, "Message Enqueuer in"=w1190) -> ("error out"=w1188:errorcluster, "Message Enqueuer out"=w1187:refnum<class "Message Enqueuer.lvclass">)  [unwired: 7 in]
                  n476 = call "Send Stop Trial.vi"("error in (no error)"=w1195, "DAQ Task"=w1185, "Stop Acquiring"=w1185, "Message Enqueuer in"=w1196) -> ("error out"=w1194:errorcluster, "Message Enqueuer out"=w1193:refnum<class "Message Enqueuer.lvclass">)  [unwired: 6 in]
                }
                frame #3 {
                  n477 = Equal?(x=w1202, y=w1201) -> (x = y?=w1199:bool)
                  n478 = Or(x=w1199, y=w1197) -> (x .or. y?=w1198:bool)
                  n479 = case shown="False" w1198 {
                    tunnel: w1200 -> [w1207 _]
                    frame False {
                      n480 = while {
                        shift-right: [w1211] -> _
                        shift-left: TRUE ("reset") -> [w1213]
                        tunnel: w1207 -> [w1209]
                        stop <- w1212 stop-if-true
                        n481 = local read "Abort Signal"() -> (w1210:bool)
                        n482 = call <userlib>:"Periodic Trigger__ogtk.vi"("time (ms)"=w1209, "reset"=w1213) -> ("Triggered"=w1211:bool)  [unwired: 11 in, 2 out]
                        n483 = Or(x=w1211, y=w1210) -> (x .or. y?=w1212:bool)
                      }
                    }
                    frame True {
                      n484 = Wait (ms)(milliseconds to wait=u32 1000) -> ()  [unwired: 1 out]
                    }
                  }
                }
              }
              n485 = Merge Errors(w1124, w1123) -> (w1122:errorcluster)
              n486 = Unbundle By Name(w1122) -> ("status"=w1121:bool)
              n487 = Select(t=w1107, s=w1107, f=FALSE) -> (s? t:f=w1110:bool)
              n488 = Or(x=w1121, y=w1110) -> (x .or. y?=w1120:bool)
            }
          }
        }
        n489 = case shown="\"Movement Input\"" w847 {
          tunnel: [FALSE ("Movement?") TRUE ("Movement?")] -> w853
          frame "Force Input", Default {
          }
          frame "Movement Input" {
          }
        }
        n490 = call "Send External Shutdown.vi"("Message Enqueuer in"=w894) -> ("error out"=w867:errorcluster)  [unwired: 9 in, 1 out]
        n491 = call "Send External Shutdown.vi"("Message Enqueuer in"=w871) -> ()  [unwired: 9 in, 2 out]
        n492 = call "Send TDMS Cleanup.vi"("Auto Clust"=w843, "Movement?"=w853, "Task info"=w852, "Force TDMS File"=w866, "Task Selection"=w851, "error in (no error)"=w867, "Accel TDMS File"=w865, "TDMS File"=w864, "Message Enqueuer in"=w870) -> ("error out"=w860:errorcluster)  [unwired: 1 in, 1 out]
        n493 = Enqueue Element(queue=w862, element=Task_Active_Enum_df."Idle", error in (no error)=w860) -> ()  [unwired: 1 in, 3 out]
      }
      frame "Start Scanning Task" {
        w1241 = refnum<class "NI Force Task.lvclass"> refnum  # Force Task
        n494 = Unbundle By Name(w1223) -> ("Monitor Select"=w1222:refnum<vi>)
        n495 = property class="LVClassControl (strict)"(reference=w1222) -> ("Value"=w1221:refnum<class "Ref Display.lvclass">)  [unwired: 1 in, 2 out]
        n496 = call <vilib>:"Application Directory.vi"() -> ("Application Directory"=w1258:path)
        n497 = call-poly <vilib>:"Panel Type Selector.vi"("Window Position"=w1221, "Default Title"="Task Window") -> ("Window out"=w1247:refnum<class "Window.lvclass">)  [unwired: 8 in, 1 out]
        n498 = Build Path(base path=w1258, name or relative path=path "temp_ni.tdms") -> (appended path=w1256:path)
        n499 = TDMS Open(10:T21."create or replace" ("operation (0:open)"), 11:w1256) -> (3:w1250:refnum<k34>)  [unwired: 5 in, 1 out]
        n500 = call <vilib>:"Launch Nested Panel.vi"("Panel"=w1247, "Nested Panel Actor"=w1241, "Panel Actor in"=w1223) -> ("Nested Actor's Enqueuer"=w1245:refnum<class "Message Enqueuer.lvclass">, "Panel Actor out"=w1246:refnum<class "GUI.lvclass">)  [unwired: 5 in, 2 out]
        n501 = in-place {
          in-place-border: [w1315] -> w1236
          in-place-border: w1250 -> [w1314]
          in-place-border: [w1314] -> w1234
          in-place-border: [w1309] -> w1225
          in-place-border: [w1306] -> w1235
          in-place-border: [w1304] -> _
          in-place-border: [w1303] -> w1251
          in-place-border: [w1300] -> w1248
          in-place-border: w1245 -> [w1299]
          in-place-border: [w1299] -> w1240
          in-place-border: [w1298] -> w1237
          in-place-border: [w1297] -> w1233
          in-place-border: [w1296] -> w1232
          in-place-border: [w1293] -> w1228
          in-place-border: [w1292] -> w1227
          in-place-border: [w1291] -> w1226
          in-place-border: [w1290] -> w1224
          in-place-border: [w1285] -> w1220
          in-place-border: [w1284] -> w1219
          in-place-border: [w1283] -> w1218
          in-place-border: [w1282] -> w1217
          n502 = in-place-cluster #16(w1246) -> ("Task Selection"=w1313:refnum<vi>, "Task Info Cluster"=w1311:refnum<vi>, "DAQ Physical Channels"=w1307:refnum<vi>, "Logger"=w1303:refnum<class "Message Enqueuer.lvclass">, "Final File Path"=w1302:refnum<vi>, "NI Data Subpanel"=w1298:refnum<vi>, "Auto Clust"=w1295:refnum<vi>, "Lissajou Subpanel"=w1290:refnum<vi>, "Force Calibration Cluster"=w1289:refnum<vi>, "Pot Calibration Cluster"=w1287:refnum<vi>, "Trial Num Update"=w1282:refnum<user-event>)  [unwired: 2 out]
          n503 = property class="Clust (strict)"(reference=w1295) -> (reference out=w1294:refnum<vi>, "Value"=w1291:T11)  [unwired: 1 in, 1 out]
          n504 = property class="Clust (strict)"(reference=w1313) -> (reference out=w1312:refnum<vi>, "Value"=w1297:T3)  [unwired: 1 in, 1 out]
          n505 = property class="Path"(reference=w1302) -> (reference out=w1301:refnum<vi>, "Value"=w1300:path)  [unwired: 1 in, 1 out]
          n506 = Unbundle By Name(w1297) -> ("Collect EMG?"=w1283:bool, "EMG Rate"=w1305:u16, "Acceleration Rate"=w1304:u16, "Input Select Type"=w1296:enum32{"Force Input", "Movement Input"})
          n507 = property class="Clust (strict)"(reference=w1289) -> (reference out=w1288:refnum<vi>, "Value"=w1285:cluster{"Left":dbl, "Right":dbl})  [unwired: 1 in, 1 out]
          n508 = property class="Clust (strict)"(reference=w1287) -> (reference out=w1286:refnum<vi>, "Value"=w1284:cluster{"Left 2":dbl, "Right 2":dbl})  [unwired: 1 in, 1 out]
          n509 = Unbundle By Name(w1291) -> ("Automate?"=w1293:bool, "Num Parabs"=w1292:u16)
          n510 = property class="Clust (strict)"(reference=w1311) -> (reference out=w1310:refnum<vi>, "Value"=w1309:T4)  [unwired: 1 in, 1 out]
          n511 = property class="Clust (strict)"(reference=w1307) -> (reference out=w1308:refnum<vi>, "Value"=w1306:T9)  [unwired: 1 in, 1 out]
          n512 = Bundle("Collect EMG?"=w1283, "EMG Rate"=w1305) -> (w1315:cluster{"Collect EMG?":bool, "EMG Rate":u16})  [unwired: 1 in]
          n513 = in-place-cluster #16("Force TDMS File"=w1314, "NI Force Task"=w1299, "Task Selection"=w1312, "Task Info Cluster"=w1310, "DAQ Physical Channels"=w1308, "Logger"=w1303, "Final File Path"=w1301, "NI Data Subpanel"=w1298, "Auto Clust"=w1294, "Lissajou Subpanel"=w1290, "Force Calibration Cluster"=w1288, "Pot Calibration Cluster"=w1286, "Trial Num Update"=w1282) -> ()  [unwired: 1 out]
        }
        n514 = call "Send Launch Viewer.vi"("EMG?"=w1218, "Subpanel ref lissajous"=w1224, "Collection Type"=w1232, "Subpanel ref task"=w1237, "Message Enqueuer in"=w1240) -> ("error out"=w1238:errorcluster, "Message Enqueuer out"=w1239:refnum<class "Message Enqueuer.lvclass">)  [unwired: 5 in]
        n515 = case shown="\"Force Input\", Default" w1232 {
          selector: w1232 -> [w1261 w1273]
          tunnel: [w1265 w1281] -> w1259
          tunnel: [w1266 w1280] -> w1254
          tunnel: w1239 -> [w1270 w1279]
          tunnel: w1238 -> [w1269 w1278]
          tunnel: w1236 -> [w1264 w1277]
          tunnel: w1235 -> [w1267 w1276]
          tunnel: w1234 -> [w1268 w1275]
          tunnel: w1225 -> [w1263 w1271]
          tunnel: TRUE -> [w1262 w1274]
          tunnel: [w1261 w1273] -> w1229
          tunnel: w1220 -> [w1260 _]
          tunnel: w1219 -> [_ w1272]
          frame "Force Input", Default {
            n516 = call "Send Initialize Force Task.vi"("Task Info In"=w1263, "Scanning?"=w1262, "EMG info"=w1264, "DAQ  Channels In"=w1267, "error in (no error)"=w1269, "TDMS File"=w1268, "Force Calibration Cluster"=w1260, "Message Enqueuer in"=w1270) -> ("error out"=w1266:errorcluster, "Message Enqueuer out"=w1265:refnum<class "Message Enqueuer.lvclass">)  [unwired: 2 in]
          }
          frame "Movement Input" {
            n517 = call "Send Initialize Movement Task.vi"("Scanning?"=w1274, "Task Info In"=w1271, "EMG info"=w1277, "DAQ  Channels In"=w1276, "error in (no error)"=w1278, "TDMS File"=w1275, "Pot Calibration Cluster"=w1272, "Message Enqueuer in"=w1279) -> ("error out"=w1280:errorcluster, "Message Enqueuer out"=w1281:refnum<class "Message Enqueuer.lvclass">)  [unwired: 2 in]
          }
        }
        n518 = case shown="True" w1228 {
          tunnel: w1259 -> [w1329 w1422]
          tunnel: w1254 -> [w1317 w1421]
          tunnel: [w1328 w1420] -> w1252
          tunnel: w1225 -> [w1324 w1413]
          tunnel: w1227 -> [w1325 _]
          tunnel: w1217 -> [w1320 w1409]
          frame True {
            n519 = property class="VI"(error in=w1317, "Front Panel.IsFrontmost"=TRUE ("Front Panel Window:Is Frontmost")) -> (error out=w1316:errorcluster)  [unwired: 1 in, 1 out]
            n520 = while {
              tunnel: w1316 -> [w1330]
              tunnel: [w1330] -> w1318
              stop <- w1333 stop-if-true
              n521 = One Button Dialog(message="Ready for acquisition", button name ("OK")="Begin") -> (true=w1333:bool)
            }
            n522 = Unbundle By Name(w1324) -> ("Trial Duration (s)"=w1326:u8)
            n523 = Multiply(x=1000, y=w1326) -> (x*y=w1322:i32)
            n524 = Add(x=w1322, y=1100) -> (x+y=w1321:i32)
            n525 = for {
              N: w1325 -> [w1353]
              tunnel: w1329 -> [w1349]
              tunnel: w1318 -> [w1346]
              tunnel: [w1358] -> w1328
              tunnel: w1321 -> [w1356]
              tunnel: w1324 -> [w1341]
              tunnel: w1320 -> [w1340]
              i -> [w1343]
              stop <- w1354 stop-if-true
              n526 = Increment(x=w1343) -> (x+1=w1339:i32)
              n527 = Equal To 0?(x=w1343) -> (x = 0?=w1344:bool)
              n528 = case shown="True" w1344 {
                tunnel: [FALSE ("Set Task Info?") TRUE ("Set Task Info?")] -> w1342
                frame False {
                }
                frame True {
                }
              }
              n529 = Generate User Event(user event=w1340, event data cluster=w1339) -> ()  [unwired: 2 in, 2 out]
              n530 = call "Send Update Template Graph.vi"("Set Task Info?"=w1342, "error in (no error)"=w1346, "Update Axes Scale"=TRUE ("Set Task Info?"), "Task Info In"=w1341, "Message Enqueuer in"=w1349) -> ("error out"=w1347:errorcluster, "Message Enqueuer out"=w1348:refnum<class "Message Enqueuer.lvclass">)  [unwired: 5 in]
              n531 = flat-sequence {
                tunnel: w1339 -> [w1371]
                tunnel: [w1377] -> w1364
                tunnel: [w1373] -> w1362
                tunnel: [w1372] -> w1357
                tunnel: w1356 -> [w1372]
                tunnel: [w1371] -> w1352
                tunnel: w1348 -> [w1370]
                tunnel: w1347 -> [w1369]
                tunnel: [w1383] -> w1365
                tunnel: w1364 -> [w1383]
                tunnel: [w1382] -> w1363
                tunnel: w1362 -> [w1382]
                tunnel: w1357 -> [w1381]
                tunnel: w1352 -> [w1379]
                tunnel: [w1379] -> w1351
                tunnel: [w1378] -> w1335
                tunnel: w1365 -> [w1395]
                tunnel: w1363 -> [w1394]
                tunnel: [w1393] -> w1361
                tunnel: [w1392] -> w1359
                tunnel: w1351 -> [w1391]
                tunnel: [w1391] -> w1350
                tunnel: [w1389] -> w1336
                tunnel: w1335 -> [w1389]
                tunnel: w1361 -> [w1402]
                tunnel: [w1402] -> w1360
                tunnel: [w1401] -> w1358
                tunnel: w1359 -> [w1401]
                tunnel: w1353 -> [w1400]
                tunnel: w1350 -> [w1399]
                tunnel: [w1396] -> w1334
                tunnel: w1336 -> [w1396]
                frame #0 {
                  n532 = call "Send Stop Trial.vi"("error in (no error)"=w1369, "DAQ Task"=TRUE, "Stop Acquiring"=FALSE, "Message Enqueuer in"=w1370) -> ("error out"=w1374:errorcluster, "Message Enqueuer out"=w1375:refnum<class "Message Enqueuer.lvclass">)  [unwired: 6 in]
                  n533 = call "Send Start Trial.vi"("error in (no error)"=w1374, "Trial Number"=w1371, "Message Enqueuer in"=w1375) -> ("error out"=w1373:errorcluster, "Message Enqueuer out"=w1377:refnum<class "Message Enqueuer.lvclass">)  [unwired: 7 in]
                }
                frame #1 {
                  n534 = while {
                    shift-right: [w1387] -> _
                    shift-left: TRUE ("Triggered") -> [w1386]
                    tunnel: w1381 -> [w1385]
                    tunnel: [w1384] -> w1378
                    stop <- w1388 stop-if-true
                    n535 = local read "Abort Signal"() -> (w1384:bool)
                    n536 = call <userlib>:"Periodic Trigger__ogtk.vi"("time (ms)"=w1385, "reset"=w1386) -> ("Triggered"=w1387:bool)  [unwired: 11 in, 2 out]
                    n537 = Or(x=w1387, y=w1384) -> (x .or. y?=w1388:bool)
                  }
                }
                frame #2 {
                  w1390 = TRUE ("Stop Acquiring")
                  n538 = call "Send Stop Trial.vi"("error in (no error)"=w1394, "DAQ Task"=w1390, "Stop Acquiring"=w1390, "Message Enqueuer in"=w1395) -> ("error out"=w1393:errorcluster, "Message Enqueuer out"=w1392:refnum<class "Message Enqueuer.lvclass">)  [unwired: 6 in]
                }
                frame #3 {
                  n539 = Equal?(x=w1400, y=w1399) -> (x = y?=w1397:bool)
                  n540 = Or(x=w1397, y=w1396) -> (x .or. y?=w1398:bool)
                  n541 = case shown="False" w1398 {
                    frame False {
                      n542 = while {
                        stop <- w1407 stop-if-true
                        n543 = local read "Abort Signal"() -> (w1406:bool)
                        n544 = One Button Dialog(message="Press \"Next\" button or Enter key to continue", button name ("OK")="Next") -> (true=w1403:bool)
                        n545 = Or(x=w1403, y=w1406) -> (x .or. y?=w1407:bool)
                      }
                    }
                    frame True {
                      n546 = Wait (ms)(milliseconds to wait=u32 2000) -> ()  [unwired: 1 out]
                    }
                  }
                }
              }
              n547 = Unbundle By Name(w1360) -> ("status"=w1355:bool)
              n548 = Select(t=w1334, s=w1334, f=FALSE) -> (s? t:f=w1337:bool)
              n549 = Or(x=w1355, y=w1337) -> (x .or. y?=w1354:bool)
            }
          }
          frame False {
            n550 = Unbundle By Name(w1413) -> ("Number of Trials"=w1419:u8, "Trial Duration (s)"=w1416:u8, "Time Between Trials (s)"=w1415:u8)
            n551 = Multiply(x=1000, y=w1416) -> (x*y=w1411:i32)
            n552 = Multiply(x=1000, y=w1415) -> (x*y=w1414:i32)
            n553 = Add(x=w1411, y=1100) -> (x+y=w1410:i32)
            n554 = for {
              N: w1419 -> [w1442]
              tunnel: w1422 -> [w1435]
              tunnel: w1421 -> [w1432]
              tunnel: [w1451] -> w1420
              tunnel: w1410 -> [w1449]
              tunnel: w1414 -> [w1447]
              tunnel: w1413 -> [w1430]
              tunnel: w1409 -> [w1429]
              i -> [w1431]
              stop <- w1443 stop-if-true
              n555 = Increment(x=w1431) -> (x+1=w1428:i32)
              n556 = Equal To 0?(x=w1431) -> (x = 0?=w1437:bool)
              n557 = case shown="True" w1437 {
                tunnel: [FALSE ("Set Task Info?") TRUE ("Set Task Info?")] -> w1436
                frame False {
                }
                frame True {
                }
              }
              n558 = Generate User Event(user event=w1429, event data cluster=w1428) -> ()  [unwired: 2 in, 2 out]
              n559 = call "Send Update Template Graph.vi"("Set Task Info?"=w1436, "error in (no error)"=w1432, "Update Axes Scale"=TRUE ("Set Task Info?"), "Task Info In"=w1430, "Message Enqueuer in"=w1435) -> ("error out"=w1433:errorcluster, "Message Enqueuer out"=w1434:refnum<class "Message Enqueuer.lvclass">)  [unwired: 5 in]
              n560 = flat-sequence {
                tunnel: w1428 -> [w1464]
                tunnel: [w1471] -> w1457
                tunnel: [w1467] -> w1455
                tunnel: [w1466] -> w1450
                tunnel: w1449 -> [w1466]
                tunnel: [w1465] -> w1448
                tunnel: w1447 -> [w1465]
                tunnel: [w1464] -> w1441
                tunnel: w1434 -> [w1463]
                tunnel: w1433 -> [w1462]
                tunnel: [w1478] -> w1458
                tunnel: w1457 -> [w1478]
                tunnel: [w1477] -> w1456
                tunnel: w1455 -> [w1477]
                tunnel: w1450 -> [w1475]
                tunnel: w1448 -> [w1476]
                tunnel: [w1476] -> w1445
                tunnel: w1441 -> [w1473]
                tunnel: [w1473] -> w1440
                tunnel: [w1472] -> w1425
                tunnel: w1458 -> [w1491]
                tunnel: w1456 -> [w1490]
                tunnel: [w1489] -> w1454
                tunnel: [w1488] -> w1452
                tunnel: [w1487] -> w1446
                tunnel: w1445 -> [w1487]
                tunnel: w1440 -> [w1486]
                tunnel: [w1486] -> w1439
                tunnel: w1425 -> [w1484]
                tunnel: [w1484] -> w1424
                tunnel: w1454 -> [w1499]
                tunnel: [w1499] -> w1453
                tunnel: [w1498] -> w1451
                tunnel: w1452 -> [w1498]
                tunnel: w1446 -> [w1495]
                tunnel: w1442 -> [w1497]
                tunnel: w1439 -> [w1496]
                tunnel: [w1492] -> w1423
                tunnel: w1424 -> [w1492]
                frame #0 {
                  n561 = call "Send Stop Trial.vi"("error in (no error)"=w1462, "DAQ Task"=TRUE, "Stop Acquiring"=FALSE, "Message Enqueuer in"=w1463) -> ("error out"=w1468:errorcluster, "Message Enqueuer out"=w1469:refnum<class "Message Enqueuer.lvclass">)  [unwired: 6 in]
                  n562 = call "Send Start Trial.vi"("error in (no error)"=w1468, "Trial Number"=w1464, "Message Enqueuer in"=w1469) -> ("error out"=w1467:errorcluster, "Message Enqueuer out"=w1471:refnum<class "Message Enqueuer.lvclass">)  [unwired: 7 in]
                }
                frame #1 {
                  n563 = while {
                    shift-right: [w1482] -> _
                    shift-left: TRUE ("Triggered") -> [w1481]
                    tunnel: w1475 -> [w1480]
                    tunnel: [w1479] -> w1472
                    stop <- w1483 stop-if-true
                    n564 = local read "Abort Signal"() -> (w1479:bool)
                    n565 = call <userlib>:"Periodic Trigger__ogtk.vi"("time (ms)"=w1480, "reset"=w1481) -> ("Triggered"=w1482:bool)  [unwired: 11 in, 2 out]
                    n566 = Or(x=w1482, y=w1479) -> (x .or. y?=w1483:bool)
                  }
                }
                frame #2 {
                  w1485 = TRUE ("Stop Acquiring")
                  n567 = call "Send Stop Trial.vi"("error in (no error)"=w1490, "DAQ Task"=w1485, "Stop Acquiring"=w1485, "Message Enqueuer in"=w1491) -> ("error out"=w1489:errorcluster, "Message Enqueuer out"=w1488:refnum<class "Message Enqueuer.lvclass">)  [unwired: 6 in]
                }
                frame #3 {
                  n568 = Equal?(x=w1497, y=w1496) -> (x = y?=w1493:bool)
                  n569 = Or(x=w1493, y=w1492) -> (x .or. y?=w1494:bool)
                  n570 = case shown="False" w1494 {
                    tunnel: w1495 -> [w1501 _]
                    frame False {
                      n571 = while {
                        shift-right: [w1505] -> _
                        shift-left: TRUE ("Triggered") -> [w1504]
                        tunnel: w1501 -> [w1502]
                        stop <- w1506 stop-if-true
                        n572 = local read "Abort Signal"() -> (w1503:bool)
                        n573 = call <userlib>:"Periodic Trigger__ogtk.vi"("time (ms)"=w1502, "reset"=w1504) -> ("Triggered"=w1505:bool)  [unwired: 11 in, 2 out]
                        n574 = Or(x=w1505, y=w1503) -> (x .or. y?=w1506:bool)
                      }
                    }
                    frame True {
                      n575 = Wait (ms)(milliseconds to wait=u32 1000) -> ()  [unwired: 1 out]
                    }
                  }
                }
              }
              n576 = Unbundle By Name(w1453) -> ("status"=w1444:bool)
              n577 = Select(t=w1423, s=w1423, f=FALSE) -> (s? t:f=w1426:bool)
              n578 = Or(x=w1444, y=w1426) -> (x .or. y?=w1443:bool)
            }
          }
        }
        n579 = case shown="\"Movement Input\"" w1229 {
          tunnel: [FALSE ("Movement?") TRUE ("Movement?")] -> w1230
          frame "Force Input", Default {
          }
          frame "Movement Input" {
          }
        }
        n580 = call "Send External Shutdown.vi"("Message Enqueuer in"=w1252) -> ("error out"=w1249:errorcluster)  [unwired: 9 in, 1 out]
        n581 = call "Send TDMS Cleanup.vi"("Auto Clust"=w1226, "Movement?"=w1230, "Task info"=w1225, "Force TDMS File"=w1234, "Task Selection"=w1233, "error in (no error)"=w1249, "TDMS File"=w1248, "Message Enqueuer in"=w1251) -> ("error out"=w1242:errorcluster)  [unwired: 2 in, 1 out]
        n582 = Enqueue Element(queue=w1243, element=Task_Active_Enum_df."Idle", error in (no error)=w1242) -> ()  [unwired: 1 in, 3 out]
      }
      frame "Start Scanning Task and Accel" {
        w1560 = refnum<class "Accelerometer.lvclass"> refnum  # Accelerometer
        w1563 = refnum<class "NI Force Task.lvclass"> refnum  # Force Task
        n583 = Unbundle By Name(w1515) -> ("Monitor Select"=w1514:refnum<vi>)
        n584 = property class="LVClassControl (strict)"(reference=w1514) -> ("Value"=w1513:refnum<class "Ref Display.lvclass">)  [unwired: 1 in, 2 out]
        n585 = control-ref of="Accelerometer Data"() -> (w1564:refnum<vi>)
        n586 = call-poly <vilib>:"Panel Type Selector.vi"("Sub Panel"=w1564) -> ("Subpanel Out"=w1561:refnum<class "Subpanel.lvclass">)  [unwired: 9 in, 1 out]
        n587 = call-poly <vilib>:"Panel Type Selector.vi"("Window Position"=w1513, "Default Title"="Task Window") -> ("Window out"=w1562:refnum<class "Window.lvclass">)  [unwired: 8 in, 1 out]
        n588 = call <vilib>:"Application Directory.vi"() -> ("Application Directory"=w1570:path)
        n589 = call <vilib>:"Application Directory.vi"() -> ("Application Directory"=w1551:path)
        n590 = Bundle("Force Task"=w1563, "Window out"=w1562) -> (w1558:T23)  [unwired: 1 in]
        n591 = Build Path(base path=w1570, name or relative path=path "temp_ni.tdms") -> (appended path=w1569:path)
        n592 = Build Path(base path=w1551, name or relative path=path "temp_accel.tdms") -> (appended path=w1549:path)
        n593 = Bundle("Accelerometer"=w1560, "Subpanel Out"=w1561) -> (w1559:T24)  [unwired: 1 in]
        n594 = Build Array(w1558, w1559) -> (w1557:T25)
        n595 = TDMS Open(10:T21."create or replace" ("operation (0:open)"), 11:w1569) -> (3:w1544:refnum<k34>)  [unwired: 5 in, 1 out]
        n596 = TDMS Open(10:T21."create or replace" ("operation (0:open)"), 11:w1549) -> (3:w1545:refnum<k34>)  [unwired: 5 in, 1 out]
        n597 = call <vilib>:"Launch Nested Panels.vi"("Nested Panel Actors"=w1557, "Panel Actor in"=w1515) -> ("Nested Actor's Enqueuers"=w1556:refnum<class "Message Enqueuer.lvclass">[], "Panel Actor out"=w1565:refnum<class "GUI.lvclass">)  [unwired: 6 in, 2 out]
        n598 = in-place {
          in-place-border: [w1629] -> w1529
          in-place-border: w1544 -> [w1628]
          in-place-border: [w1628] -> w1527
          in-place-border: [w1627] -> w1530
          in-place-border: [w1622] -> w1525
          in-place-border: [w1619] -> w1528
          in-place-border: [w1615] -> w1520
          in-place-border: [w1617] -> w1552
          in-place-border: w1545 -> [w1616]
          in-place-border: [w1616] -> w1542
          in-place-border: [w1614] -> w1535
          in-place-border: [w1613] -> w1546
          in-place-border: [w1610] -> w1541
          in-place-border: [w1609] -> w1531
          in-place-border: [w1608] -> w1526
          in-place-border: [w1607] -> w1524
          in-place-border: [w1604] -> w1519
          in-place-border: [w1603] -> w1518
          in-place-border: [w1602] -> w1517
          in-place-border: [w1601] -> w1516
          in-place-border: [w1596] -> w1512
          in-place-border: [w1595] -> w1511
          in-place-border: [w1594] -> w1510
          n599 = in-place-cluster #17(w1565) -> ("Task Selection"=w1626:refnum<vi>, "Task Info Cluster"=w1624:refnum<vi>, "DAQ Physical Channels"=w1620:refnum<vi>, "Logger"=w1613:refnum<class "Message Enqueuer.lvclass">, "Final File Path"=w1612:refnum<vi>, "NI Data Subpanel"=w1609:refnum<vi>, "Auto Clust"=w1606:refnum<vi>, "Lissajou Subpanel"=w1601:refnum<vi>, "Force Calibration Cluster"=w1600:refnum<vi>, "Pot Calibration Cluster"=w1599:refnum<vi>, "Trial Num Update"=w1594:refnum<user-event>)  [unwired: 4 out]
          n600 = in-place-array #18(w1556, 0, 1) -> (w1614:refnum<class "Message Enqueuer.lvclass">, w1615:refnum<class "Message Enqueuer.lvclass">)
          n601 = property class="Clust (strict)"(reference=w1606) -> (reference out=w1605:refnum<vi>, "Value"=w1602:T11)  [unwired: 1 in, 1 out]
          n602 = property class="Clust (strict)"(reference=w1626) -> (reference out=w1625:refnum<vi>, "Value"=w1608:T3)  [unwired: 1 in, 1 out]
          n603 = property class="Path"(reference=w1612) -> (reference out=w1611:refnum<vi>, "Value"=w1610:path)  [unwired: 1 in, 1 out]
          n604 = property class="Clust (strict)"(reference=w1600) -> (reference out=w1598:refnum<vi>, "Value"=w1627:cluster{"Left":dbl, "Right":dbl})  [unwired: 1 in, 1 out]
          n605 = property class="Clust (strict)"(reference=w1599) -> (reference out=w1597:refnum<vi>, "Value"=w1596:cluster{"Left 2":dbl, "Right 2":dbl})  [unwired: 1 in, 1 out]
          n606 = Unbundle By Name(w1608) -> ("Collect EMG?"=w1595:bool, "EMG Rate"=w1618:u16, "Acceleration Rate"=w1617:u16, "Input Select Type"=w1607:enum32{"Force Input", "Movement Input"})
          n607 = Unbundle By Name(w1602) -> ("Automate?"=w1604:bool, "Num Parabs"=w1603:u16)
          n608 = property class="Clust (strict)"(reference=w1624) -> (reference out=w1623:refnum<vi>, "Value"=w1622:T4)  [unwired: 1 in, 1 out]
          n609 = property class="Clust (strict)"(reference=w1620) -> (reference out=w1621:refnum<vi>, "Value"=w1619:T9)  [unwired: 1 in, 1 out]
          n610 = Bundle("Collect EMG?"=w1595, "EMG Rate"=w1618) -> (w1629:cluster{"Collect EMG?":bool, "EMG Rate":u16})  [unwired: 1 in]
          n611 = in-place-cluster #17("Force TDMS File"=w1628, "NI Force Task"=w1614, "Task Selection"=w1625, "Task Info Cluster"=w1623, "DAQ Physical Channels"=w1621, "Accelerometer"=w1615, "Accel TDMS File"=w1616, "Logger"=w1613, "Final File Path"=w1611, "NI Data Subpanel"=w1609, "Auto Clust"=w1605, "Lissajou Subpanel"=w1601, "Force Calibration Cluster"=w1598, "Pot Calibration Cluster"=w1597, "Trial Num Update"=w1594) -> ()  [unwired: 1 out]
          n612 = in-place-array #18(w1614, w1615) -> ()  [unwired: 3 out]
        }
        n613 = call "Send Launch Viewer.vi"("EMG?"=w1511, "Subpanel ref lissajous"=w1516, "Collection Type"=w1524, "Subpanel ref task"=w1531, "Message Enqueuer in"=w1535) -> ("error out"=w1534:errorcluster, "Message Enqueuer out"=w1536:refnum<class "Message Enqueuer.lvclass">)  [unwired: 5 in]
        n614 = call "Send Initialize Accel Task.vi"("Accel TDMS File"=w1542, "Accel Rate"=w1552, "Message Enqueuer in"=w1520) -> ("error out"=w1532:errorcluster, "Message Enqueuer out"=w1553:refnum<class "Message Enqueuer.lvclass">)  [unwired: 7 in]
        n615 = case shown="\"Force Input\", Default" w1524 {
          selector: w1524 -> [w1572 w1584]
          tunnel: [w1581 w1593] -> w1571
          tunnel: w1536 -> [w1582 w1592]
          tunnel: w1534 -> [w1577 w1591]
          tunnel: [w1580 w1590] -> w1533
          tunnel: w1530 -> [w1576 _]
          tunnel: w1529 -> [w1579 w1589]
          tunnel: w1528 -> [w1578 w1588]
          tunnel: w1527 -> [w1575 w1587]
          tunnel: w1525 -> [w1574 w1586]
          tunnel: TRUE -> [w1573 w1585]
          tunnel: [w1572 w1584] -> w1521
          tunnel: w1512 -> [_ w1583]
          frame "Force Input", Default {
            n616 = call "Send Initialize Force Task.vi"("Task Info In"=w1574, "Scanning?"=w1573, "EMG info"=w1579, "DAQ  Channels In"=w1578, "error in (no error)"=w1577, "TDMS File"=w1575, "Force Calibration Cluster"=w1576, "Message Enqueuer in"=w1582) -> ("error out"=w1580:errorcluster, "Message Enqueuer out"=w1581:refnum<class "Message Enqueuer.lvclass">)  [unwired: 2 in]
          }
          frame "Movement Input" {
            n617 = call "Send Initialize Movement Task.vi"("Scanning?"=w1585, "Task Info In"=w1586, "EMG info"=w1589, "DAQ  Channels In"=w1588, "error in (no error)"=w1591, "TDMS File"=w1587, "Pot Calibration Cluster"=w1583, "Message Enqueuer in"=w1592) -> ("error out"=w1590:errorcluster, "Message Enqueuer out"=w1593:refnum<class "Message Enqueuer.lvclass">)  [unwired: 2 in]
          }
        }
        n618 = case shown="True" w1519 {
          tunnel: w1571 -> [w1647 w1770]
          tunnel: [w1646 w1769] -> w1566
          tunnel: w1553 -> [w1645 w1768]
          tunnel: [w1644 w1767] -> w1547
          tunnel: w1533 -> [w1634 w1759]
          tunnel: w1532 -> [w1631 w1765]
          tunnel: w1525 -> [w1640 w1758]
          tunnel: w1518 -> [w1641 _]
          tunnel: w1510 -> [w1636 w1754]
          frame True {
            n619 = property class="VI"(error in=w1634, "Front Panel.IsFrontmost"=TRUE ("Front Panel Window:Is Frontmost")) -> (error out=w1633:errorcluster)  [unwired: 1 in, 1 out]
            n620 = while {
              tunnel: w1633 -> [w1649]
              tunnel: [w1649] -> w1632
              tunnel: [w1648] -> w1630
              tunnel: w1631 -> [w1648]
              stop <- w1652 stop-if-true
              n621 = One Button Dialog(message="Ready for acquisition", button name ("OK")="Begin") -> (true=w1652:bool)
            }
            n622 = Unbundle By Name(w1640) -> ("Trial Duration (s)"=w1642:u8)
            n623 = Multiply(x=1000, y=w1642) -> (x*y=w1637:i32)
            n624 = Add(x=w1637, y=1100) -> (x+y=w1638:i32)
            n625 = for {
              N: w1641 -> [w1673]
              tunnel: w1647 -> [w1669]
              tunnel: [w1688] -> w1646
              tunnel: w1638 -> [w1686]
              tunnel: w1645 -> [w1685]
              tunnel: [w1678] -> w1644
              tunnel: w1632 -> [w1668]
              tunnel: w1630 -> [w1676]
              tunnel: w1640 -> [w1660]
              tunnel: w1636 -> [w1659]
              i -> [w1662]
              stop <- w1677 stop-if-true
              n626 = Equal To 0?(x=w1662) -> (x = 0?=w1663:bool)
              n627 = case shown="False" w1663 {
                tunnel: [FALSE ("Set Task Info?") TRUE ("Set Task Info?")] -> w1661
                frame False {
                }
                frame True {
                }
              }
              n628 = Increment(x=w1662) -> (x+1=w1658:i32)
              n629 = Generate User Event(user event=w1659, event data cluster=w1658) -> ()  [unwired: 2 in, 2 out]
              n630 = call "Send Update Template Graph.vi"("Set Task Info?"=w1661, "error in (no error)"=w1668, "Update Axes Scale"=TRUE ("Set Task Info?"), "Task Info In"=w1660, "Message Enqueuer in"=w1669) -> ("error out"=w1667:errorcluster, "Message Enqueuer out"=w1666:refnum<class "Message Enqueuer.lvclass">)  [unwired: 5 in]
              n631 = flat-sequence {
                tunnel: w1658 -> [w1700]
                tunnel: [w1713] -> w1693
                tunnel: [w1709] -> w1691
                tunnel: [w1708] -> w1687
                tunnel: w1686 -> [w1708]
                tunnel: w1685 -> [w1707]
                tunnel: [w1703] -> w1683
                tunnel: [w1702] -> w1681
                tunnel: w1676 -> [w1701]
                tunnel: [w1700] -> w1672
                tunnel: w1667 -> [w1699]
                tunnel: w1666 -> [w1698]
                tunnel: [w1721] -> w1694
                tunnel: w1693 -> [w1721]
                tunnel: [w1720] -> w1692
                tunnel: w1691 -> [w1720]
                tunnel: w1687 -> [w1716]
                tunnel: [w1719] -> w1684
                tunnel: w1683 -> [w1719]
                tunnel: [w1718] -> w1682
                tunnel: w1681 -> [w1718]
                tunnel: w1672 -> [w1715]
                tunnel: [w1715] -> w1671
                tunnel: [w1714] -> w1655
                tunnel: w1694 -> [w1738]
                tunnel: w1692 -> [w1737]
                tunnel: [w1736] -> w1690
                tunnel: [w1735] -> w1689
                tunnel: w1684 -> [w1733]
                tunnel: w1682 -> [w1732]
                tunnel: [w1731] -> w1680
                tunnel: [w1730] -> w1679
                tunnel: w1671 -> [w1729]
                tunnel: [w1729] -> w1670
                tunnel: w1655 -> [w1727]
                tunnel: [w1727] -> w1654
                tunnel: w1690 -> [w1747]
                tunnel: [w1747] -> w1675
                tunnel: [w1746] -> w1688
                tunnel: w1689 -> [w1746]
                tunnel: [w1745] -> w1674
                tunnel: w1680 -> [w1745]
                tunnel: w1679 -> [w1744]
                tunnel: [w1744] -> w1678
                tunnel: w1673 -> [w1743]
                tunnel: w1670 -> [w1742]
                tunnel: [w1740] -> w1653
                tunnel: w1654 -> [w1740]
                frame #0 {
                  n632 = call "Send Stop Trial.vi"("error in (no error)"=w1701, "Stop Acquiring"=FALSE, "Message Enqueuer in"=w1707) -> ("error out"=w1704:errorcluster, "Message Enqueuer out"=w1705:refnum<class "Message Enqueuer.lvclass">)  [unwired: 7 in]
                  n633 = call "Send Stop Trial.vi"("error in (no error)"=w1699, "DAQ Task"=TRUE, "Stop Acquiring"=FALSE, "Message Enqueuer in"=w1698) -> ("error out"=w1710:errorcluster, "Message Enqueuer out"=w1711:refnum<class "Message Enqueuer.lvclass">)  [unwired: 6 in]
                  n634 = call "Send Start Trial.vi"("error in (no error)"=w1704, "Trial Number"=w1700, "Message Enqueuer in"=w1705) -> ("error out"=w1702:errorcluster, "Message Enqueuer out"=w1703:refnum<class "Message Enqueuer.lvclass">)  [unwired: 7 in]
                  n635 = call "Send Start Trial.vi"("error in (no error)"=w1710, "Trial Number"=w1700, "Message Enqueuer in"=w1711) -> ("error out"=w1709:errorcluster, "Message Enqueuer out"=w1713:refnum<class "Message Enqueuer.lvclass">)  [unwired: 7 in]
                }
                frame #1 {
                  n636 = while {
                    shift-right: [w1725] -> _
                    shift-left: TRUE ("Triggered") -> [w1724]
                    tunnel: w1716 -> [w1723]
                    tunnel: [w1722] -> w1714
                    stop <- w1726 stop-if-true
                    n637 = local read "Abort Signal"() -> (w1722:bool)
                    n638 = call <userlib>:"Periodic Trigger__ogtk.vi"("time (ms)"=w1723, "reset"=w1724) -> ("Triggered"=w1725:bool)  [unwired: 11 in, 2 out]
                    n639 = Or(x=w1725, y=w1722) -> (x .or. y?=w1726:bool)
                  }
                }
                frame #2 {
                  w1728 = TRUE ("Stop Acquiring")
                  n640 = call "Send Stop Trial.vi"("error in (no error)"=w1732, "Stop Acquiring"=TRUE, "Message Enqueuer in"=w1733) -> ("error out"=w1731:errorcluster, "Message Enqueuer out"=w1730:refnum<class "Message Enqueuer.lvclass">)  [unwired: 7 in]
                  n641 = call "Send Stop Trial.vi"("error in (no error)"=w1737, "DAQ Task"=w1728, "Stop Acquiring"=w1728, "Message Enqueuer in"=w1738) -> ("error out"=w1736:errorcluster, "Message Enqueuer out"=w1735:refnum<class "Message Enqueuer.lvclass">)  [unwired: 6 in]
                }
                frame #3 {
                  n642 = Equal?(x=w1743, y=w1742) -> (x = y?=w1739:bool)
                  n643 = Or(x=w1739, y=w1740) -> (x .or. y?=w1741:bool)
                  n644 = case shown="False" w1741 {
                    frame False {
                      n645 = while {
                        stop <- w1752 stop-if-true
                        n646 = local read "Abort Signal"() -> (w1751:bool)
                        n647 = One Button Dialog(message="Press \"Next\" button or Enter key to continue", button name ("OK")="Next") -> (true=w1748:bool)
                        n648 = Or(x=w1748, y=w1751) -> (x .or. y?=w1752:bool)
                      }
                    }
                    frame True {
                      n649 = Wait (ms)(milliseconds to wait=u32 2000) -> ()  [unwired: 1 out]
                    }
                  }
                }
              }
              n650 = Merge Errors(w1675, w1674) -> (w1665:errorcluster)
              n651 = Select(t=w1653, s=w1653, f=FALSE) -> (s? t:f=w1656:bool)
              n652 = Or(x=w1665, y=w1656) -> (x .or. y?=w1677:bool)
            }
          }
          frame False {
            n653 = Unbundle By Name(w1758) -> ("Number of Trials"=w1766:u8, "Trial Duration (s)"=w1762:u8, "Time Between Trials (s)"=w1761:u8)
            n654 = Multiply(x=1000, y=w1762) -> (x*y=w1756:i32)
            n655 = Multiply(x=1000, y=w1761) -> (x*y=w1760:i32)
            n656 = Add(x=w1756, y=1100) -> (x+y=w1755:i32)
            n657 = for {
              N: w1766 -> [w1790]
              tunnel: w1770 -> [w1783]
              tunnel: [w1811] -> w1769
              tunnel: w1755 -> [w1809]
              tunnel: w1760 -> [w1807]
              tunnel: w1768 -> [w1804]
              tunnel: [w1797] -> w1767
              tunnel: w1765 -> [w1795]
              tunnel: w1759 -> [w1782]
              tunnel: w1758 -> [w1779]
              tunnel: w1754 -> [w1777]
              i -> [w1778]
              stop <- w1796 stop-if-true
              n658 = Increment(x=w1778) -> (x+1=w1776:i32)
              n659 = Equal To 0?(x=w1778) -> (x = 0?=w1785:bool)
              n660 = Generate User Event(user event=w1777, event data cluster=w1776) -> ()  [unwired: 2 in, 2 out]
              n661 = case shown="False" w1785 {
                tunnel: [FALSE ("Set Task Info?") TRUE ("Set Task Info?")] -> w1784
                frame False {
                }
                frame True {
                }
              }
              n662 = call "Send Update Template Graph.vi"("Set Task Info?"=w1784, "error in (no error)"=w1782, "Update Axes Scale"=TRUE ("Set Task Info?"), "Task Info In"=w1779, "Message Enqueuer in"=w1783) -> ("error out"=w1781:errorcluster, "Message Enqueuer out"=w1780:refnum<class "Message Enqueuer.lvclass">)  [unwired: 5 in]
              n663 = flat-sequence {
                tunnel: w1776 -> [w1823]
                tunnel: [w1837] -> w1816
                tunnel: [w1833] -> w1814
                tunnel: [w1832] -> w1810
                tunnel: w1809 -> [w1832]
                tunnel: [w1831] -> w1808
                tunnel: w1807 -> [w1831]
                tunnel: w1804 -> [w1830]
                tunnel: [w1826] -> w1802
                tunnel: [w1825] -> w1800
                tunnel: w1795 -> [w1824]
                tunnel: [w1823] -> w1789
                tunnel: w1781 -> [w1822]
                tunnel: w1780 -> [w1821]
                tunnel: [w1846] -> w1817
                tunnel: w1816 -> [w1846]
                tunnel: [w1845] -> w1815
                tunnel: w1814 -> [w1845]
                tunnel: w1810 -> [w1840]
                tunnel: w1808 -> [w1844]
                tunnel: [w1844] -> w1805
                tunnel: [w1843] -> w1803
                tunnel: w1802 -> [w1843]
                tunnel: [w1842] -> w1801
                tunnel: w1800 -> [w1842]
                tunnel: w1789 -> [w1839]
                tunnel: [w1839] -> w1788
                tunnel: [w1838] -> w1773
                tunnel: w1817 -> [w1864]
                tunnel: w1815 -> [w1863]
                tunnel: [w1862] -> w1813
                tunnel: [w1861] -> w1812
                tunnel: [w1860] -> w1806
                tunnel: w1805 -> [w1860]
                tunnel: w1803 -> [w1858]
                tunnel: w1801 -> [w1857]
                tunnel: [w1856] -> w1799
                tunnel: [w1855] -> w1798
                tunnel: w1788 -> [w1854]
                tunnel: [w1854] -> w1787
                tunnel: w1773 -> [w1852]
                tunnel: [w1852] -> w1772
                tunnel: w1813 -> [w1874]
                tunnel: [w1874] -> w1794
                tunnel: [w1873] -> w1811
                tunnel: w1812 -> [w1873]
                tunnel: w1806 -> [w1868]
                tunnel: [w1872] -> w1793
                tunnel: w1799 -> [w1872]
                tunnel: w1798 -> [w1871]
                tunnel: [w1871] -> w1797
                tunnel: w1790 -> [w1870]
                tunnel: w1787 -> [w1869]
                tunnel: [w1865] -> w1771
                tunnel: w1772 -> [w1865]
                frame #0 {
                  n664 = call "Send Stop Trial.vi"("error in (no error)"=w1824, "Stop Acquiring"=FALSE, "Message Enqueuer in"=w1830) -> ("error out"=w1827:errorcluster, "Message Enqueuer out"=w1828:refnum<class "Message Enqueuer.lvclass">)  [unwired: 7 in]
                  n665 = call "Send Stop Trial.vi"("error in (no error)"=w1822, "DAQ Task"=TRUE, "Stop Acquiring"=FALSE, "Message Enqueuer in"=w1821) -> ("error out"=w1834:errorcluster, "Message Enqueuer out"=w1835:refnum<class "Message Enqueuer.lvclass">)  [unwired: 6 in]
                  n666 = call "Send Start Trial.vi"("error in (no error)"=w1827, "Trial Number"=w1823, "Message Enqueuer in"=w1828) -> ("error out"=w1825:errorcluster, "Message Enqueuer out"=w1826:refnum<class "Message Enqueuer.lvclass">)  [unwired: 7 in]
                  n667 = call "Send Start Trial.vi"("error in (no error)"=w1834, "Trial Number"=w1823, "Message Enqueuer in"=w1835) -> ("error out"=w1833:errorcluster, "Message Enqueuer out"=w1837:refnum<class "Message Enqueuer.lvclass">)  [unwired: 7 in]
                }
                frame #1 {
                  n668 = while {
                    shift-right: [w1850] -> _
                    shift-left: TRUE ("Triggered") -> [w1849]
                    tunnel: w1840 -> [w1848]
                    tunnel: [w1847] -> w1838
                    stop <- w1851 stop-if-true
                    n669 = local read "Abort Signal"() -> (w1847:bool)
                    n670 = call <userlib>:"Periodic Trigger__ogtk.vi"("time (ms)"=w1848, "reset"=w1849) -> ("Triggered"=w1850:bool)  [unwired: 11 in, 2 out]
                    n671 = Or(x=w1850, y=w1847) -> (x .or. y?=w1851:bool)
                  }
                }
                frame #2 {
                  w1853 = TRUE ("Stop Acquiring")
                  n672 = call "Send Stop Trial.vi"("error in (no error)"=w1857, "Stop Acquiring"=TRUE, "Message Enqueuer in"=w1858) -> ("error out"=w1856:errorcluster, "Message Enqueuer out"=w1855:refnum<class "Message Enqueuer.lvclass">)  [unwired: 7 in]
                  n673 = call "Send Stop Trial.vi"("error in (no error)"=w1863, "DAQ Task"=w1853, "Stop Acquiring"=w1853, "Message Enqueuer in"=w1864) -> ("error out"=w1862:errorcluster, "Message Enqueuer out"=w1861:refnum<class "Message Enqueuer.lvclass">)  [unwired: 6 in]
                }
                frame #3 {
                  n674 = Equal?(x=w1870, y=w1869) -> (x = y?=w1866:bool)
                  n675 = Or(x=w1866, y=w1865) -> (x .or. y?=w1867:bool)
                  n676 = case shown="True" w1867 {
                    tunnel: w1868 -> [w1875 _]
                    frame False {
                      n677 = while {
                        shift-right: [w1880] -> _
                        shift-left: TRUE ("Triggered") -> [w1879]
                        tunnel: w1875 -> [w1877]
                        stop <- w1881 stop-if-true
                        n678 = local read "Abort Signal"() -> (w1878:bool)
                        n679 = call <userlib>:"Periodic Trigger__ogtk.vi"("time (ms)"=w1877, "reset"=w1879) -> ("Triggered"=w1880:bool)  [unwired: 11 in, 2 out]
                        n680 = Or(x=w1880, y=w1878) -> (x .or. y?=w1881:bool)
                      }
                    }
                    frame True {
                      n681 = Wait (ms)(milliseconds to wait=u32 1000) -> ()  [unwired: 1 out]
                    }
                  }
                }
              }
              n682 = Merge Errors(w1794, w1793) -> (w1792:errorcluster)
              n683 = Unbundle By Name(w1792) -> ("status"=w1791:bool)
              n684 = Select(t=w1771, s=w1771, f=FALSE) -> (s? t:f=w1774:bool)
              n685 = Or(x=w1791, y=w1774) -> (x .or. y?=w1796:bool)
            }
          }
        }
        n686 = case shown="\"Movement Input\"" w1521 {
          tunnel: [FALSE ("Movement?") TRUE ("Movement?")] -> w1522
          frame "Force Input", Default {
          }
          frame "Movement Input" {
          }
        }
        n687 = call "Send External Shutdown.vi"("Message Enqueuer in"=w1566) -> ("error out"=w1543:errorcluster)  [unwired: 9 in, 1 out]
        n688 = call "Send External Shutdown.vi"("Message Enqueuer in"=w1547) -> ()  [unwired: 9 in, 2 out]
        n689 = call "Send TDMS Cleanup.vi"("Auto Clust"=w1517, "Movement?"=w1522, "Task info"=w1525, "Force TDMS File"=w1527, "Task Selection"=w1526, "error in (no error)"=w1543, "Accel TDMS File"=w1542, "TDMS File"=w1541, "Message Enqueuer in"=w1546) -> ("error out"=w1537:errorcluster)  [unwired: 1 in, 1 out]
        n690 = Enqueue Element(queue=w1539, element=Task_Active_Enum_df."Idle", error in (no error)=w1537) -> ()  [unwired: 1 in, 3 out]
      }
      frame "EMG Mode" {
        w1905 = refnum<class "NI Force Task.lvclass"> refnum  # Force Task
        n691 = call <vilib>:"Application Directory.vi"() -> ("Application Directory"=w1919:path)
        n692 = Build Path(base path=w1919, name or relative path=path "temp_ni.tdms") -> (appended path=w1917:path)
        n693 = call-poly <vilib>:"Panel Type Selector.vi"("Autoshow? (T)"=FALSE, "Default Title"="Task Window") -> ("Window out"=w1911:refnum<class "Window.lvclass">)  [unwired: 8 in, 1 out]
        n694 = TDMS Open(10:T21."create or replace" ("operation (0:open)"), 11:w1917) -> (3:w1912:refnum<k34>)  [unwired: 5 in, 1 out]
        n695 = call <vilib>:"Launch Nested Panel.vi"("Panel"=w1911, "Nested Panel Actor"=w1905, "Panel Actor in"=w1898) -> ("Nested Actor's Enqueuer"=w1909:refnum<class "Message Enqueuer.lvclass">, "Panel Actor out"=w1910:refnum<class "GUI.lvclass">)  [unwired: 5 in, 2 out]
        n696 = in-place {
          in-place-border: [w1947] -> w1895
          in-place-border: w1912 -> [w1922]
          in-place-border: [w1922] -> _
          in-place-border: [w1942] -> w1885
          in-place-border: [w1939] -> _
          in-place-border: [w1936] -> _
          in-place-border: [w1935] -> w1913
          in-place-border: [w1921] -> _
          in-place-border: w1909 -> [w1932]
          in-place-border: [w1932] -> w1904
          in-place-border: [w1931] -> w1903
          in-place-border: [w1930] -> _
          in-place-border: [w1929] -> _
          in-place-border: [w1926] -> w1901
          in-place-border: [w1925] -> w1900
          in-place-border: [w1924] -> _
          in-place-border: [w1923] -> w1899
          in-place-border: [w1922] -> w1890
          in-place-border: [w1921] -> w1889
          in-place-border: [w1920] -> w1886
          n697 = in-place-cluster #19(w1910) -> ("Task Selection"=w1946:refnum<vi>, "Task Info Cluster"=w1944:refnum<vi>, "DAQ Physical Channels"=w1940:refnum<vi>, "Logger"=w1935:refnum<class "Message Enqueuer.lvclass">, "Final File Path"=w1934:refnum<vi>, "NI Data Subpanel"=w1931:refnum<vi>, "Auto Clust"=w1928:refnum<vi>, "Lissajou Subpanel"=w1923:refnum<vi>, "Trial Num Update"=w1920:refnum<user-event>)  [unwired: 2 out]
          n698 = property class="Clust (strict)"(reference=w1946) -> (reference out=w1945:refnum<vi>, "Value"=w1930:T3)  [unwired: 1 in, 1 out]
          n699 = property class="Clust (strict)"(reference=w1928) -> (reference out=w1927:refnum<vi>, "Value"=w1924:T11)  [unwired: 1 in, 1 out]
          n700 = property class="Path"(reference=w1934) -> (reference out=w1933:refnum<vi>, "Value"=w1921:path)  [unwired: 1 in, 1 out]
          n701 = Unbundle By Name(w1930) -> ("Collect EMG?"=w1938:bool, "EMG Rate"=w1937:u16, "Acceleration Rate"=w1936:u16, "Input Select Type"=w1929:enum32{"Force Input", "Movement Input"})
          n702 = Unbundle By Name(w1924) -> ("Automate?"=w1926:bool, "Num Parabs"=w1925:u16)
          n703 = property class="Clust (strict)"(reference=w1944) -> (reference out=w1943:refnum<vi>, "Value"=w1942:T4)  [unwired: 1 in, 1 out]
          n704 = property class="Clust (strict)"(reference=w1940) -> (reference out=w1941:refnum<vi>, "Value"=w1939:T9)  [unwired: 1 in, 1 out]
          n705 = Bundle("Collect EMG?"=w1938, "EMG Rate"=w1937) -> (w1947:cluster{"Collect EMG?":bool, "EMG Rate":u16})  [unwired: 1 in]
          n706 = in-place-cluster #19("Force TDMS File"=w1922, "NI Force Task"=w1932, "Task Selection"=w1945, "Task Info Cluster"=w1943, "DAQ Physical Channels"=w1941, "Logger"=w1935, "Final File Path"=w1933, "NI Data Subpanel"=w1931, "Auto Clust"=w1927, "Lissajou Subpanel"=w1923, "Trial Num Update"=w1920) -> ()  [unwired: 1 out]
        }
        n707 = local read "EMG Master Config"() -> (w1894:T8)
        n708 = call "Send Launch Viewer.vi"("EMG?"=FALSE, "Subpanel ref lissajous"=w1899, "Collection Type"=Collection_Type_df."EMG only" ("Collection mode"), "Subpanel ref task"=w1903, "Message Enqueuer in"=w1904) -> ("error out"=w1893:errorcluster, "Message Enqueuer out"=w1896:refnum<class "Message Enqueuer.lvclass">)  [unwired: 5 in]
        n709 = call "Send Initiallize EMG Task.vi"("TDMS File"=w1890, "error in (no error)"=w1893, "EMG Master Config"=w1894, "EMG info"=w1895, "Message Enqueuer in"=w1896) -> ("error out"=w1891:errorcluster, "Message Enqueuer out"=w1892:refnum<class "Message Enqueuer.lvclass">)  [unwired: 5 in]
        n710 = case shown="True" w1901 {
          tunnel: [w1961 w2046] -> w1914
          tunnel: w1885 -> [w1957 w2044]
          tunnel: w1900 -> [w1958 _]
          tunnel: w1892 -> [w1956 w2038]
          tunnel: w1891 -> [w1950 w2037]
          tunnel: w1886 -> [w1952 w2033]
          frame True {
            n711 = property class="VI"(error in=w1950, "Front Panel.IsFrontmost"=TRUE ("Front Panel Window:Is Frontmost")) -> (error out=w1949:errorcluster)  [unwired: 1 in, 1 out]
            n712 = while {
              tunnel: w1949 -> [w1962]
              tunnel: [w1962] -> w1948
              stop <- w1965 stop-if-true
              n713 = One Button Dialog(message="Ready for acquisition", button name ("OK")="Begin") -> (true=w1965:bool)
            }
            n714 = Unbundle By Name(w1957) -> ("Trial Duration (s)"=w1959:u8)
            n715 = Multiply(x=1000, y=w1959) -> (x*y=w1955:i32)
            n716 = Add(x=w1955, y=1100) -> (x+y=w1954:i32)
            n717 = for {
              N: w1958 -> [w1975]
              tunnel: [w1983] -> w1961
              tunnel: w1954 -> [w1981]
              tunnel: w1956 -> [w1974]
              tunnel: w1948 -> [w1973]
              tunnel: w1952 -> [w1972]
              i -> [w1991]
              stop <- w1979 stop-if-true
              n718 = Increment(x=w1991) -> (x+1=w1971:i32)
              n719 = Generate User Event(user event=w1972, event data cluster=w1971) -> ()  [unwired: 2 in, 2 out]
              n720 = flat-sequence {
                tunnel: w1971 -> [w1995]
                tunnel: [w2001] -> w1989
                tunnel: [w1997] -> w1987
                tunnel: [w1996] -> w1982
                tunnel: w1981 -> [w1996]
                tunnel: [w1995] -> w1976
                tunnel: w1974 -> [w1993]
                tunnel: w1973 -> [w1992]
                tunnel: [w2007] -> w1990
                tunnel: w1989 -> [w2007]
                tunnel: [w2006] -> w1988
                tunnel: w1987 -> [w2006]
                tunnel: w1982 -> [w2005]
                tunnel: [w2003] -> w1977
                tunnel: w1976 -> [w2003]
                tunnel: [w2002] -> w1968
                tunnel: w1990 -> [w2019]
                tunnel: w1988 -> [w2018]
                tunnel: [w2017] -> w1986
                tunnel: [w2016] -> w1984
                tunnel: [w2015] -> w1978
                tunnel: w1977 -> [w2015]
                tunnel: w1968 -> [w2013]
                tunnel: [w2013] -> w1967
                tunnel: w1986 -> [w2026]
                tunnel: [w2026] -> w1985
                tunnel: [w2025] -> w1983
                tunnel: w1984 -> [w2025]
                tunnel: w1978 -> [w2023]
                tunnel: w1975 -> [w2024]
                tunnel: [w2020] -> w1966
                tunnel: w1967 -> [w2020]
                frame #0 {
                  n721 = call "Send Stop Trial.vi"("error in (no error)"=w1992, "DAQ Task"=TRUE, "Stop Acquiring"=FALSE, "Message Enqueuer in"=w1993) -> ("error out"=w1998:errorcluster, "Message Enqueuer out"=w1999:refnum<class "Message Enqueuer.lvclass">)  [unwired: 6 in]
                  n722 = call "Send Start Trial.vi"("error in (no error)"=w1998, "Trial Number"=w1995, "Message Enqueuer in"=w1999) -> ("error out"=w1997:errorcluster, "Message Enqueuer out"=w2001:refnum<class "Message Enqueuer.lvclass">)  [unwired: 7 in]
                }
                frame #1 {
                  n723 = while {
                    tunnel: w2005 -> [w2012]
                    shift-right: [w2010] -> _
                    shift-left: TRUE ("reset") -> [w2011]
                    tunnel: [w2008] -> w2002
                    stop <- w2009 stop-if-true
                    n724 = call <userlib>:"Periodic Trigger__ogtk.vi"("time (ms)"=w2012, "reset"=w2011) -> ("Triggered"=w2010:bool)  [unwired: 11 in, 2 out]
                    n725 = local read "Abort Signal"() -> (w2008:bool)
                    n726 = Or(x=w2010, y=w2008) -> (x .or. y?=w2009:bool)
                  }
                }
                frame #2 {
                  w2014 = TRUE ("Stop Acquiring")
                  n727 = call "Send Stop Trial.vi"("error in (no error)"=w2018, "DAQ Task"=w2014, "Stop Acquiring"=w2014, "Message Enqueuer in"=w2019) -> ("error out"=w2017:errorcluster, "Message Enqueuer out"=w2016:refnum<class "Message Enqueuer.lvclass">)  [unwired: 6 in]
                }
                frame #3 {
                  n728 = Equal?(x=w2024, y=w2023) -> (x = y?=w2022:bool)
                  n729 = Or(x=w2022, y=w2020) -> (x .or. y?=w2021:bool)
                  n730 = case shown="False" w2021 {
                    frame False {
                      n731 = while {
                        stop <- w2030 stop-if-true
                        n732 = local read "Abort Signal"() -> (w2031:bool)
                        n733 = One Button Dialog(message="Press \"Next\" button or Enter key to continue", button name ("OK")="Next") -> (true=w2029:bool)
                        n734 = Or(x=w2029, y=w2031) -> (x .or. y?=w2030:bool)
                      }
                    }
                    frame True {
                      n735 = Wait (ms)(milliseconds to wait=u32 2000) -> ()  [unwired: 1 out]
                    }
                  }
                }
              }
              n736 = Select(t=w1966, s=w1966, f=FALSE) -> (s? t:f=w1969:bool)
              n737 = Unbundle By Name(w1985) -> ("status"=w1980:bool)
              n738 = Or(x=w1980, y=w1969) -> (x .or. y?=w1979:bool)
            }
          }
          frame False {
            n739 = Unbundle By Name(w2044) -> ("Number of Trials"=w2045:u8, "Trial Duration (s)"=w2042:u8, "Time Between Trials (s)"=w2041:u8)
            n740 = Multiply(x=1000, y=w2042) -> (x*y=w2036:i32)
            n741 = Add(x=w2036, y=1100) -> (x+y=w2035:i32)
            n742 = Multiply(x=1000, y=w2041) -> (x*y=w2039:i32)
            n743 = for {
              N: w2045 -> [w2056]
              tunnel: [w2068] -> w2046
              tunnel: w2035 -> [w2066]
              tunnel: w2039 -> [w2064]
              tunnel: w2038 -> [w2055]
              tunnel: w2037 -> [w2054]
              tunnel: w2033 -> [w2053]
              i -> [w2076]
              stop <- w2060 stop-if-true
              n744 = Increment(x=w2076) -> (x+1=w2052:i32)
              n745 = Generate User Event(user event=w2053, event data cluster=w2052) -> ()  [unwired: 2 in, 2 out]
              n746 = flat-sequence {
                tunnel: w2052 -> [w2080]
                tunnel: [w2087] -> w2074
                tunnel: [w2083] -> w2072
                tunnel: [w2082] -> w2067
                tunnel: w2066 -> [w2082]
                tunnel: [w2081] -> w2065
                tunnel: w2064 -> [w2081]
                tunnel: [w2080] -> w2057
                tunnel: w2055 -> [w2078]
                tunnel: w2054 -> [w2077]
                tunnel: [w2094] -> w2075
                tunnel: w2074 -> [w2094]
                tunnel: [w2093] -> w2073
                tunnel: w2072 -> [w2093]
                tunnel: w2067 -> [w2091]
                tunnel: w2065 -> [w2092]
                tunnel: [w2092] -> w2062
                tunnel: [w2089] -> w2058
                tunnel: w2057 -> [w2089]
                tunnel: [w2088] -> w2049
                tunnel: w2075 -> [w2107]
                tunnel: w2073 -> [w2106]
                tunnel: [w2105] -> w2071
                tunnel: [w2104] -> w2069
                tunnel: [w2103] -> w2063
                tunnel: w2062 -> [w2103]
                tunnel: [w2102] -> w2059
                tunnel: w2058 -> [w2102]
                tunnel: w2049 -> [w2100]
                tunnel: [w2100] -> w2048
                tunnel: w2071 -> [w2115]
                tunnel: [w2115] -> w2070
                tunnel: [w2114] -> w2068
                tunnel: w2069 -> [w2114]
                tunnel: w2063 -> [w2111]
                tunnel: w2059 -> [w2112]
                tunnel: w2056 -> [w2113]
                tunnel: [w2108] -> w2047
                tunnel: w2048 -> [w2108]
                frame #0 {
                  n747 = call "Send Stop Trial.vi"("error in (no error)"=w2077, "DAQ Task"=TRUE, "Stop Acquiring"=FALSE, "Message Enqueuer in"=w2078) -> ("error out"=w2084:errorcluster, "Message Enqueuer out"=w2085:refnum<class "Message Enqueuer.lvclass">)  [unwired: 6 in]
                  n748 = call "Send Start Trial.vi"("error in (no error)"=w2084, "Trial Number"=w2080, "Message Enqueuer in"=w2085) -> ("error out"=w2083:errorcluster, "Message Enqueuer out"=w2087:refnum<class "Message Enqueuer.lvclass">)  [unwired: 7 in]
                }
                frame #1 {
                  n749 = while {
                    tunnel: w2091 -> [w2099]
                    shift-right: [w2097] -> _
                    shift-left: TRUE ("reset") -> [w2098]
                    tunnel: [w2095] -> w2088
                    stop <- w2096 stop-if-true
                    n750 = call <userlib>:"Periodic Trigger__ogtk.vi"("time (ms)"=w2099, "reset"=w2098) -> ("Triggered"=w2097:bool)  [unwired: 11 in, 2 out]
                    n751 = local read "Abort Signal"() -> (w2095:bool)
                    n752 = Or(x=w2097, y=w2095) -> (x .or. y?=w2096:bool)
                  }
                }
                frame #2 {
                  w2101 = TRUE ("Stop Acquiring")
                  n753 = call "Send Stop Trial.vi"("error in (no error)"=w2106, "DAQ Task"=w2101, "Stop Acquiring"=w2101, "Message Enqueuer in"=w2107) -> ("error out"=w2105:errorcluster, "Message Enqueuer out"=w2104:refnum<class "Message Enqueuer.lvclass">)  [unwired: 6 in]
                }
                frame #3 {
                  n754 = Equal?(x=w2113, y=w2112) -> (x = y?=w2109:bool)
                  n755 = Or(x=w2109, y=w2108) -> (x .or. y?=w2110:bool)
                  n756 = case shown="True" w2110 {
                    tunnel: w2111 -> [w2117 _]
                    frame False {
                      n757 = while {
                        tunnel: w2117 -> [w2122]
                        shift-right: [w2120] -> _
                        shift-left: TRUE ("reset") -> [w2121]
                        stop <- w2118 stop-if-true
                        n758 = local read "Abort Signal"() -> (w2119:bool)
                        n759 = call <userlib>:"Periodic Trigger__ogtk.vi"("time (ms)"=w2122, "reset"=w2121) -> ("Triggered"=w2120:bool)  [unwired: 11 in, 2 out]
                        n760 = Or(x=w2120, y=w2119) -> (x .or. y?=w2118:bool)
                      }
                    }
                    frame True {
                      n761 = Wait (ms)(milliseconds to wait=u32 2000) -> ()  [unwired: 1 out]
                    }
                  }
                }
              }
              n762 = Unbundle By Name(w2070) -> ("status"=w2061:bool)
              n763 = Select(t=w2047, s=w2047, f=FALSE) -> (s? t:f=w2050:bool)
              n764 = Or(x=w2061, y=w2050) -> (x .or. y?=w2060:bool)
            }
          }
        }
        n765 = call "Send External Shutdown.vi"("Message Enqueuer in"=w1914) -> ("error out"=w1902:errorcluster)  [unwired: 9 in, 1 out]
        n766 = call "Send TDMS Cleanup EMG only.vi"("error in (no error)"=w1902, "Force TDMS File"=w1890, "TDMS File"=w1889, "Message Enqueuer in"=w1913) -> ("error out"=w1906:errorcluster)  [unwired: 6 in, 1 out]
        n767 = Enqueue Element(queue=w1907, element=Task_Active_Enum_df."Idle", error in (no error)=w1906) -> ()  [unwired: 1 in, 3 out]
      }
      frame "EMG and Accel Mode" {
        w2144 = refnum<class "Accelerometer.lvclass"> refnum  # Accelerometer
        w2137 = refnum<class "NI Force Task.lvclass"> refnum  # Force Task
        n768 = control-ref of="Accelerometer Data"() -> (w2125:refnum<vi>)
        n769 = call-poly <vilib>:"Panel Type Selector.vi"("Autoshow? (T)"=FALSE, "Default Title"="Task Window") -> ("Window out"=w2141:refnum<class "Window.lvclass">)  [unwired: 8 in, 1 out]
        n770 = call-poly <vilib>:"Panel Type Selector.vi"("Sub Panel"=w2125) -> ("Subpanel Out"=w2145:refnum<class "Subpanel.lvclass">)  [unwired: 9 in, 1 out]
        n771 = call <vilib>:"Application Directory.vi"() -> ("Application Directory"=w2150:path)
        n772 = call <vilib>:"Application Directory.vi"() -> ("Application Directory"=w2177:path)
        n773 = Build Path(base path=w2150, name or relative path=path "temp_accel.tdms") -> (appended path=w2148:path)
        n774 = Bundle("Force Task"=w2137, "Window out"=w2141) -> (w2140:T23)  [unwired: 1 in]
        n775 = Build Path(base path=w2177, name or relative path=path "temp_ni.tdms") -> (appended path=w2175:path)
        n776 = Bundle("Accelerometer"=w2144, "Subpanel Out"=w2145) -> (w2139:T24)  [unwired: 1 in]
        n777 = Build Array(w2140, w2139) -> (w2138:T25)
        n778 = TDMS Open(10:T21."create or replace" ("operation (0:open)"), 11:w2148) -> (3:w2146:refnum<k34>)  [unwired: 5 in, 1 out]
        n779 = TDMS Open(10:T21."create or replace" ("operation (0:open)"), 11:w2175) -> (3:w2170:refnum<k34>)  [unwired: 5 in, 1 out]
        n780 = call <vilib>:"Launch Nested Panels.vi"("Nested Panel Actors"=w2138, "Panel Actor in"=w2143) -> ("Nested Actor's Enqueuers"=w2136:refnum<class "Message Enqueuer.lvclass">[], "Panel Actor out"=w2142:refnum<class "GUI.lvclass">)  [unwired: 6 in, 2 out]
        n781 = in-place {
          in-place-border: [w2207] -> w2158
          in-place-border: w2170 -> [w2184]
          in-place-border: [w2184] -> _
          in-place-border: [w2202] -> w2165
          in-place-border: [w2199] -> _
          in-place-border: [w2196] -> w2171
          in-place-border: [w2183] -> _
          in-place-border: [w2193] -> w2166
          in-place-border: [w2192] -> _
          in-place-border: [w2191] -> _
          in-place-border: [w2188] -> w2163
          in-place-border: [w2187] -> w2162
          in-place-border: [w2186] -> _
          in-place-border: [w2185] -> w2161
          in-place-border: [w2184] -> w2153
          in-place-border: [w2183] -> w2152
          in-place-border: w2146 -> [w2180]
          in-place-border: [w2182] -> w2133
          in-place-border: [w2181] -> w2132
          in-place-border: [w2180] -> w2126
          in-place-border: [w2179] -> w2128
          in-place-border: [w2178] -> w2124
          n782 = in-place-cluster #20(w2142) -> ("Task Selection"=w2206:refnum<vi>, "Task Info Cluster"=w2204:refnum<vi>, "DAQ Physical Channels"=w2200:refnum<vi>, "Logger"=w2196:refnum<class "Message Enqueuer.lvclass">, "Final File Path"=w2195:refnum<vi>, "NI Data Subpanel"=w2193:refnum<vi>, "Auto Clust"=w2190:refnum<vi>, "Lissajou Subpanel"=w2185:refnum<vi>, "Trial Num Update"=w2178:refnum<user-event>)  [unwired: 4 out]
          n783 = in-place-array #21(w2136, 0, 1) -> (w2179:refnum<class "Message Enqueuer.lvclass">, w2182:refnum<class "Message Enqueuer.lvclass">)
          n784 = property class="Clust (strict)"(reference=w2206) -> (reference out=w2205:refnum<vi>, "Value"=w2192:T3)  [unwired: 1 in, 1 out]
          n785 = property class="Clust (strict)"(reference=w2190) -> (reference out=w2189:refnum<vi>, "Value"=w2186:T11)  [unwired: 1 in, 1 out]
          n786 = property class="Path"(reference=w2195) -> (reference out=w2194:refnum<vi>, "Value"=w2183:path)  [unwired: 1 in, 1 out]
          n787 = Unbundle By Name(w2192) -> ("Collect EMG?"=w2198:bool, "EMG Rate"=w2197:u16, "Acceleration Rate"=w2181:u16, "Input Select Type"=w2191:enum32{"Force Input", "Movement Input"})
          n788 = Unbundle By Name(w2186) -> ("Automate?"=w2188:bool, "Num Parabs"=w2187:u16)
          n789 = property class="Clust (strict)"(reference=w2204) -> (reference out=w2203:refnum<vi>, "Value"=w2202:T4)  [unwired: 1 in, 1 out]
          n790 = property class="Clust (strict)"(reference=w2200) -> (reference out=w2201:refnum<vi>, "Value"=w2199:T9)  [unwired: 1 in, 1 out]
          n791 = Bundle("Collect EMG?"=w2198, "EMG Rate"=w2197) -> (w2207:cluster{"Collect EMG?":bool, "EMG Rate":u16})  [unwired: 1 in]
          n792 = in-place-cluster #20("Force TDMS File"=w2184, "NI Force Task"=w2179, "Task Selection"=w2205, "Task Info Cluster"=w2203, "DAQ Physical Channels"=w2201, "Logger"=w2196, "Final File Path"=w2194, "NI Data Subpanel"=w2193, "Auto Clust"=w2189, "Lissajou Subpanel"=w2185, "Accel TDMS File"=w2180, "Accelerometer"=w2182, "Trial Num Update"=w2178) -> ()  [unwired: 1 out]
          n793 = in-place-array #21(w2179, w2182) -> ()  [unwired: 3 out]
        }
        n794 = call "Send Initialize Accel Task.vi"("Accel TDMS File"=w2126, "Accel Rate"=w2132, "Message Enqueuer in"=w2133) -> ("error out"=w2130:errorcluster, "Message Enqueuer out"=w2131:refnum<class "Message Enqueuer.lvclass">)  [unwired: 7 in]
        n795 = local read "EMG Master Config"() -> (w2157:T8)
        n796 = call "Send Launch Viewer.vi"("EMG?"=FALSE, "Subpanel ref lissajous"=w2161, "Collection Type"=Collection_Type_df."EMG only" ("Collection mode"), "Subpanel ref task"=w2166, "Message Enqueuer in"=w2128) -> ("error out"=w2156:errorcluster, "Message Enqueuer out"=w2159:refnum<class "Message Enqueuer.lvclass">)  [unwired: 5 in]
        n797 = call "Send Initiallize EMG Task.vi"("TDMS File"=w2153, "error in (no error)"=w2156, "EMG Master Config"=w2157, "EMG info"=w2158, "Message Enqueuer in"=w2159) -> ("error out"=w2154:errorcluster, "Message Enqueuer out"=w2155:refnum<class "Message Enqueuer.lvclass">)  [unwired: 5 in]
        n798 = case shown="True" w2163 {
          tunnel: [w2225 w2336] -> w2172
          tunnel: w2165 -> [w2221 w2334]
          tunnel: w2162 -> [w2222 _]
          tunnel: w2155 -> [w2220 w2328]
          tunnel: w2154 -> [w2212 w2327]
          tunnel: w2131 -> [w2219 w2326]
          tunnel: w2130 -> [w2209 w2325]
          tunnel: [w2218 w2324] -> w2129
          tunnel: w2124 -> [w2214 w2320]
          frame True {
            n799 = property class="VI"(error in=w2212, "Front Panel.IsFrontmost"=TRUE ("Front Panel Window:Is Frontmost")) -> (error out=w2211:errorcluster)  [unwired: 1 in, 1 out]
            n800 = while {
              tunnel: w2211 -> [w2227]
              tunnel: [w2227] -> w2210
              tunnel: [w2226] -> w2208
              tunnel: w2209 -> [w2226]
              stop <- w2230 stop-if-true
              n801 = One Button Dialog(message="Ready for acquisition", button name ("OK")="Begin") -> (true=w2230:bool)
            }
            n802 = Unbundle By Name(w2221) -> ("Trial Duration (s)"=w2223:u8)
            n803 = Multiply(x=1000, y=w2223) -> (x*y=w2216:i32)
            n804 = Add(x=1100 ("y"), y=w2216) -> (x+y=w2215:i32)
            n805 = for {
              N: w2222 -> [w2248]
              tunnel: [w2256] -> w2225
              tunnel: w2215 -> [w2254]
              tunnel: w2220 -> [w2247]
              tunnel: w2210 -> [w2246]
              tunnel: w2219 -> [w2245]
              tunnel: w2208 -> [w2244]
              tunnel: [w2238] -> w2218
              tunnel: w2214 -> [w2237]
              i -> [w2264]
              stop <- w2252 stop-if-true
              n806 = Increment(x=w2264) -> (x+1=w2236:i32)
              n807 = Generate User Event(user event=w2237, event data cluster=w2236) -> ()  [unwired: 2 in, 2 out]
              n808 = flat-sequence {
                tunnel: w2236 -> [w2265]
                tunnel: [w2281] -> w2262
                tunnel: [w2277] -> w2260
                tunnel: [w2276] -> w2255
                tunnel: w2254 -> [w2276]
                tunnel: [w2265] -> w2249
                tunnel: w2247 -> [w2274]
                tunnel: w2246 -> [w2273]
                tunnel: w2245 -> [w2269]
                tunnel: w2244 -> [w2268]
                tunnel: [w2267] -> w2242
                tunnel: [w2266] -> w2241
                tunnel: [w2289] -> w2263
                tunnel: w2262 -> [w2289]
                tunnel: [w2288] -> w2261
                tunnel: w2260 -> [w2288]
                tunnel: w2255 -> [w2287]
                tunnel: [w2285] -> w2250
                tunnel: w2249 -> [w2285]
                tunnel: [w2284] -> w2243
                tunnel: w2242 -> [w2284]
                tunnel: w2241 -> [w2283]
                tunnel: [w2283] -> w2240
                tunnel: [w2282] -> w2233
                tunnel: w2263 -> [w2305]
                tunnel: w2261 -> [w2304]
                tunnel: [w2303] -> w2259
                tunnel: [w2302] -> w2257
                tunnel: [w2301] -> w2251
                tunnel: w2250 -> [w2301]
                tunnel: w2243 -> [w2298]
                tunnel: w2240 -> [w2297]
                tunnel: [w2296] -> w2239
                tunnel: w2233 -> [w2295]
                tunnel: [w2295] -> w2232
                tunnel: w2259 -> [w2313]
                tunnel: [w2313] -> w2258
                tunnel: [w2312] -> w2256
                tunnel: w2257 -> [w2312]
                tunnel: w2251 -> [w2310]
                tunnel: w2248 -> [w2311]
                tunnel: [w2309] -> w2238
                tunnel: w2239 -> [w2309]
                tunnel: [w2306] -> w2231
                tunnel: w2232 -> [w2306]
                frame #0 {
                  n809 = call "Send Stop Trial.vi"("error in (no error)"=w2273, "DAQ Task"=TRUE, "Stop Acquiring"=FALSE, "Message Enqueuer in"=w2274) -> ("error out"=w2278:errorcluster, "Message Enqueuer out"=w2279:refnum<class "Message Enqueuer.lvclass">)  [unwired: 6 in]
                  n810 = call "Send Stop Trial.vi"("error in (no error)"=w2268, "Stop Acquiring"=FALSE, "Message Enqueuer in"=w2269) -> ("error out"=w2270:errorcluster, "Message Enqueuer out"=w2272:refnum<class "Message Enqueuer.lvclass">)  [unwired: 7 in]
                  n811 = call "Send Start Trial.vi"("error in (no error)"=w2278, "Trial Number"=w2265, "Message Enqueuer in"=w2279) -> ("error out"=w2277:errorcluster, "Message Enqueuer out"=w2281:refnum<class "Message Enqueuer.lvclass">)  [unwired: 7 in]
                  n812 = call "Send Start Trial.vi"("error in (no error)"=w2270, "Trial Number"=w2265, "Message Enqueuer in"=w2272) -> ("error out"=w2266:errorcluster, "Message Enqueuer out"=w2267:refnum<class "Message Enqueuer.lvclass">)  [unwired: 7 in]
                }
                frame #1 {
                  n813 = while {
                    tunnel: w2287 -> [w2294]
                    shift-right: [w2292] -> _
                    shift-left: TRUE ("reset") -> [w2293]
                    tunnel: [w2290] -> w2282
                    stop <- w2291 stop-if-true
                    n814 = call <userlib>:"Periodic Trigger__ogtk.vi"("time (ms)"=w2294, "reset"=w2293) -> ("Triggered"=w2292:bool)  [unwired: 11 in, 2 out]
                    n815 = local read "Abort Signal"() -> (w2290:bool)
                    n816 = Or(x=w2292, y=w2290) -> (x .or. y?=w2291:bool)
                  }
                }
                frame #2 {
                  w2300 = TRUE ("Stop Acquiring")
                  n817 = call "Send Stop Trial.vi"("error in (no error)"=w2304, "DAQ Task"=w2300, "Stop Acquiring"=w2300, "Message Enqueuer in"=w2305) -> ("error out"=w2303:errorcluster, "Message Enqueuer out"=w2302:refnum<class "Message Enqueuer.lvclass">)  [unwired: 6 in]
                  n818 = call "Send Stop Trial.vi"("error in (no error)"=w2297, "Stop Acquiring"=TRUE, "Message Enqueuer in"=w2298) -> ("Message Enqueuer out"=w2296:refnum<class "Message Enqueuer.lvclass">)  [unwired: 7 in, 1 out]
                }
                frame #3 {
                  n819 = Equal?(x=w2311, y=w2310) -> (x = y?=w2307:bool)
                  n820 = Or(x=w2307, y=w2306) -> (x .or. y?=w2308:bool)
                  n821 = case shown="False" w2308 {
                    frame False {
                      n822 = while {
                        stop <- w2317 stop-if-true
                        n823 = local read "Abort Signal"() -> (w2318:bool)
                        n824 = One Button Dialog(message="Press \"Next\" button or Enter key to continue", button name ("OK")="Next") -> (true=w2316:bool)
                        n825 = Or(x=w2316, y=w2318) -> (x .or. y?=w2317:bool)
                      }
                    }
                    frame True {
                      n826 = Wait (ms)(milliseconds to wait=u32 2000) -> ()  [unwired: 1 out]
                    }
                  }
                }
              }
              n827 = Unbundle By Name(w2258) -> ("status"=w2253:bool)
              n828 = Select(t=w2231, s=w2231, f=FALSE) -> (s? t:f=w2234:bool)
              n829 = Or(x=w2253, y=w2234) -> (x .or. y?=w2252:bool)
            }
          }
          frame False {
            n830 = Unbundle By Name(w2334) -> ("Number of Trials"=w2335:u8, "Trial Duration (s)"=w2332:u8, "Time Between Trials (s)"=w2331:u8)
            n831 = Multiply(x=1000, y=w2332) -> (x*y=w2323:i32)
            n832 = Add(x=1100 ("y"), y=w2323) -> (x+y=w2321:i32)
            n833 = Multiply(x=1000, y=w2331) -> (x*y=w2329:i32)
            n834 = for {
              N: w2335 -> [w2358]
              tunnel: [w2369] -> w2336
              tunnel: w2321 -> [w2367]
              tunnel: w2329 -> [w2365]
              tunnel: w2328 -> [w2357]
              tunnel: w2327 -> [w2356]
              tunnel: w2326 -> [w2355]
              tunnel: w2325 -> [w2354]
              tunnel: [w2344] -> w2324
              tunnel: w2320 -> [w2343]
              i -> [w2376]
              stop <- w2362 stop-if-true
              n835 = Increment(x=w2376) -> (x+1=w2342:i32)
              n836 = Generate User Event(user event=w2343, event data cluster=w2342) -> ()  [unwired: 2 in, 2 out]
              n837 = flat-sequence {
                tunnel: w2342 -> [w2379]
                tunnel: [w2394] -> w2374
                tunnel: [w2390] -> w2372
                tunnel: [w2389] -> w2368
                tunnel: w2367 -> [w2389]
                tunnel: [w2388] -> w2366
                tunnel: w2365 -> [w2388]
                tunnel: [w2379] -> w2359
                tunnel: w2357 -> [w2386]
                tunnel: w2356 -> [w2385]
                tunnel: w2355 -> [w2384]
                tunnel: w2354 -> [w2381]
                tunnel: [w2378] -> w2352
                tunnel: [w2377] -> w2351
                tunnel: [w2403] -> w2375
                tunnel: w2374 -> [w2403]
                tunnel: [w2402] -> w2373
                tunnel: w2372 -> [w2402]
                tunnel: w2368 -> [w2400]
                tunnel: w2366 -> [w2401]
                tunnel: [w2401] -> w2363
                tunnel: [w2398] -> w2360
                tunnel: w2359 -> [w2398]
                tunnel: [w2397] -> w2353
                tunnel: w2352 -> [w2397]
                tunnel: w2351 -> [w2396]
                tunnel: [w2396] -> w2350
                tunnel: [w2395] -> w2339
                tunnel: w2375 -> [w2421]
                tunnel: w2373 -> [w2420]
                tunnel: [w2419] -> w2371
                tunnel: [w2418] -> w2370
                tunnel: [w2417] -> w2364
                tunnel: w2363 -> [w2417]
                tunnel: [w2416] -> w2361
                tunnel: w2360 -> [w2416]
                tunnel: w2353 -> [w2414]
                tunnel: w2350 -> [w2413]
                tunnel: [w2411] -> w2348
                tunnel: [w2410] -> w2347
                tunnel: w2339 -> [w2409]
                tunnel: [w2409] -> w2338
                tunnel: w2371 -> [w2431]
                tunnel: [w2431] -> w2349
                tunnel: [w2430] -> w2369
                tunnel: w2370 -> [w2430]
                tunnel: w2364 -> [w2427]
                tunnel: w2361 -> [w2428]
                tunnel: w2358 -> [w2429]
                tunnel: [w2426] -> w2346
                tunnel: w2348 -> [w2426]
                tunnel: [w2425] -> w2344
                tunnel: w2347 -> [w2425]
                tunnel: [w2422] -> w2337
                tunnel: w2338 -> [w2422]
                frame #0 {
                  n838 = call "Send Stop Trial.vi"("error in (no error)"=w2385, "DAQ Task"=TRUE, "Stop Acquiring"=FALSE, "Message Enqueuer in"=w2386) -> ("error out"=w2391:errorcluster, "Message Enqueuer out"=w2392:refnum<class "Message Enqueuer.lvclass">)  [unwired: 6 in]
                  n839 = call "Send Stop Trial.vi"("error in (no error)"=w2381, "Stop Acquiring"=FALSE, "Message Enqueuer in"=w2384) -> ("error out"=w2380:errorcluster, "Message Enqueuer out"=w2383:refnum<class "Message Enqueuer.lvclass">)  [unwired: 7 in]
                  n840 = call "Send Start Trial.vi"("error in (no error)"=w2391, "Trial Number"=w2379, "Message Enqueuer in"=w2392) -> ("error out"=w2390:errorcluster, "Message Enqueuer out"=w2394:refnum<class "Message Enqueuer.lvclass">)  [unwired: 7 in]
                  n841 = call "Send Start Trial.vi"("error in (no error)"=w2380, "Trial Number"=w2379, "Message Enqueuer in"=w2383) -> ("error out"=w2377:errorcluster, "Message Enqueuer out"=w2378:refnum<class "Message Enqueuer.lvclass">)  [unwired: 7 in]
                }
                frame #1 {
                  n842 = while {
                    tunnel: w2400 -> [w2408]
                    shift-right: [w2406] -> _
                    shift-left: TRUE ("reset") -> [w2407]
                    tunnel: [w2404] -> w2395
                    stop <- w2405 stop-if-true
                    n843 = call <userlib>:"Periodic Trigger__ogtk.vi"("time (ms)"=w2408, "reset"=w2407) -> ("Triggered"=w2406:bool)  [unwired: 11 in, 2 out]
                    n844 = local read "Abort Signal"() -> (w2404:bool)
                    n845 = Or(x=w2406, y=w2404) -> (x .or. y?=w2405:bool)
                  }
                }
                frame #2 {
                  w2415 = TRUE ("Stop Acquiring")
                  n846 = call "Send Stop Trial.vi"("error in (no error)"=w2420, "DAQ Task"=w2415, "Stop Acquiring"=w2415, "Message Enqueuer in"=w2421) -> ("error out"=w2419:errorcluster, "Message Enqueuer out"=w2418:refnum<class "Message Enqueuer.lvclass">)  [unwired: 6 in]
                  n847 = call "Send Stop Trial.vi"("error in (no error)"=w2413, "Stop Acquiring"=TRUE, "Message Enqueuer in"=w2414) -> ("error out"=w2411:errorcluster, "Message Enqueuer out"=w2410:refnum<class "Message Enqueuer.lvclass">)  [unwired: 7 in]
                }
                frame #3 {
                  n848 = Equal?(x=w2429, y=w2428) -> (x = y?=w2424:bool)
                  n849 = Or(x=w2424, y=w2422) -> (x .or. y?=w2423:bool)
                  n850 = case shown="True" w2423 {
                    tunnel: w2427 -> [w2433 _]
                    frame False {
                      n851 = while {
                        tunnel: w2433 -> [w2438]
                        shift-right: [w2436] -> _
                        shift-left: TRUE ("reset") -> [w2437]
                        stop <- w2434 stop-if-true
                        n852 = local read "Abort Signal"() -> (w2435:bool)
                        n853 = call <userlib>:"Periodic Trigger__ogtk.vi"("time (ms)"=w2438, "reset"=w2437) -> ("Triggered"=w2436:bool)  [unwired: 11 in, 2 out]
                        n854 = Or(x=w2436, y=w2435) -> (x .or. y?=w2434:bool)
                      }
                    }
                    frame True {
                      n855 = Wait (ms)(milliseconds to wait=u32 2000) -> ()  [unwired: 1 out]
                    }
                  }
                }
              }
              n856 = Merge Errors(w2349, w2346) -> (w2345:errorcluster)
              n857 = Select(t=w2337, s=w2337, f=FALSE) -> (s? t:f=w2340:bool)
              n858 = Or(x=w2345, y=w2340) -> (x .or. y?=w2362:bool)
            }
          }
        }
        n859 = call "Send External Shutdown.vi"("Message Enqueuer in"=w2129) -> ()  [unwired: 9 in, 2 out]
        n860 = call "Send External Shutdown.vi"("Message Enqueuer in"=w2172) -> ("error out"=w2164:errorcluster)  [unwired: 9 in, 1 out]
        n861 = call "Send TDMS Cleanup EMG only.vi"("Accel TDMS File"=w2126, "error in (no error)"=w2164, "Force TDMS File"=w2153, "TDMS File"=w2152, "Message Enqueuer in"=w2171) -> ("error out"=w2167:errorcluster)  [unwired: 5 in, 1 out]
        n862 = Enqueue Element(queue=w2168, element=Task_Active_Enum_df."Idle", error in (no error)=w2167) -> ()  [unwired: 1 in, 3 out]
      }
      frame "Stop Helper" {
      }
      frame "Task Config Update" {
        n863 = property on="Task Selection" class="Clust (strict)"() -> ("Controls[]"=w2445:refnum<vi>[])  [unwired: 2 in, 2 out]
        n864 = property on="Auto Clust" class="Clust (strict)"() -> ("Controls[]"=w2444:refnum<vi>[])  [unwired: 2 in, 2 out]
        n865 = property on="MVC Temp" class="DigNum (strict)"() -> (error out=w2442:errorcluster, "Value"=w2441:dbl)  [unwired: 2 in, 1 out]
        n866 = in-place {
          n867 = in-place-array #22(w2445, 0, 1) -> (w2459:refnum<vi>, w2449:refnum<vi>)
          n868 = in-place-array #23(w2444, 0) -> (w2455:refnum<vi>)
          n869 = property class="Ctl"(reference=w2455) -> (reference out=w2454:refnum<vi>, "Value"=w2452:variant)  [unwired: 1 in, 1 out]
          n870 = property class="Ctl"(reference=w2459) -> (reference out=w2458:refnum<vi>, "Value"=w2456:variant)  [unwired: 1 in, 1 out]
          n871 = property class="Ctl"(reference=w2449) -> (reference out=w2448:refnum<vi>, "Value"=w2451:variant)  [unwired: 1 in, 1 out]
          n872 = property class="Ctl"(reference=w2454, "Val(Sgnl)"=w2452) -> (reference out=w2453:refnum<vi>)  [unwired: 1 in, 1 out]
          n873 = property class="Ctl"(reference=w2458, "Val(Sgnl)"=w2456) -> (reference out=w2457:refnum<vi>)  [unwired: 1 in, 1 out]
          n874 = property class="Ctl"(reference=w2448, "Val(Sgnl)"=w2451) -> (reference out=w2450:refnum<vi>)  [unwired: 1 in, 1 out]
          n875 = in-place-array #22(w2457, w2450) -> ()  [unwired: 3 out]
          n876 = in-place-array #23(w2453) -> ()  [unwired: 2 out]
        }
        n877 = property on="Adjusted MVC (N)" class="DigNum (strict)"(error in=w2442, "Val(Sgnl)"=w2441) -> ()  [unwired: 1 in, 2 out]
      }
    }
  }
  n878 = Unregister For Events(event registration refnum=w33) -> ()  [unwired: 1 in, 1 out]
  n879 = Release Queue(queue=w21) -> ()  [unwired: 2 in, 3 out]
